vi "Main (1366x768).vi"() -> ()   [LabVIEW 2013]
uses:
  Controls/Enum - SRTRS State.ctl
  <vilib>/Utility/miscctls.llb/LVRowAndColumnTypeDef.ctl
  <vilib>/Utility/config.llb/NI_LVConfig.lvlib
  <vilib>/Utility/miscctls.llb/LVPointTypeDef.ctl
  Controls/Combo Box.ctl
  Controls/ET3500 Program Status.ctl
  <vilib>/nisyscfg/nisyscfg.lvlib
  <vilib>/Utility/miscctls.llb/LVRowAndColumnUnsignedTypeDef.ctl
  <vilib>/event_ctls.llb/eventvkey.ctl
  <vilib>/Utility/miscctls.llb/LVSelectionTypeDef.ctl
  <vilib>/nisyscfg/Close (System).vi
  <vilib>/Utility/config.llb/Write Key (String).vi
panel:
  in  "Tab Header":enum32{"Page 1"}(tab)
  in  "Close":bool
  out "Plant and Furnace Name":string="OneSubsea, Johor / BH0277."
  in  "Setup Load Debug":bool
  in  "Debug Close":bool
  in  "Tab Footer":enum32{"Page 2"}(tab)
  out "date/time string":string="Jan 25, 2014  09:14:11"
  out "File Version":string
  in  "Tab Body":T1(tab)=enum."Master Data"
  in  "User":string
  in  "Setup New":bool
  in  "Setup Edit":bool
  out "Transaction No":string caption="Transaction No."
  in  "Tab Setup":enum32{"Part Details", "Furnace Settings"}(tab)=enum."Furnace Settings" caption="Setup"
  in  "Channel Mapping":T2 caption="Channels Mapping"
  in  "Item Details":T3={"Order No."="", "Oper. No."="", "Qty."=1, "NCR No."="", "NCR Boolean"=FALSE, "Customer No."="", "Customer Name"="", "Project"="", "Sales Order"="", "Item No."="", "Material"="", "Revision"="", "Material Description"="", "Serial No."="", "Material Filename"=""} {"Qty." min=1 max=99}
  in  "Part Details Delete":bool
  in  "Part Details Add":bool
  in  "Notes":string
  in  "No.":i32=1 caption="Item Number" min=1 max=100
  out "Setup Thermocouple Location":picture caption="Thermocouples Position: Outline"
  in  "Part Details":i32(listbox)=-1
  in  "FHS Ramp Rate Units":string="°C"
  in  "cRIO Set Time":bool
  in  "Read ET3500 Program":bool
  in  "FHS Target Temp Units":string="°C"
  in  "MCListBox AWPS Remove Button":bool
  in  "MCListBox AWPS Add Button":bool
  out "CompactRIO Module Details":i32(listbox)=-1
  out "Furnace Calibration":T4={"Furnace Serial No"="100", "Last Inspection Date"="2013-12-05", "Next Inspection Due Date"="2014-12-05"} caption="Furnace Details"
  in  "Additional WPS/Ref":T6 caption="Additional WPS"
  in  "WPS Details Setup":T7={"WPS/Ref"="", "Rev"="", "Hold Temperature"="", "WPS Details Temperature Units"="°C", "Hold Time (HH:MM)"="", "Extra WPS"="", "Extra Rev"=""} caption="WPS Details"
  in  "MCListBox AWPS":i32(listbox)=-1 caption="Additional WPS/Ref MCListBox"
  out "MCListBox FHS Setup":i32(listbox)=-1 caption="Furnace Heating Sequence"
  in  "MCListBox FHS Setup Add Button":bool
  in  "MCListBox FHS Setup Remove Button":bool
  in  "Setup Save":bool
  in  "Parameter":bool
  out "ET3504 Status":string="Offline."
  out "Info.":T8={"Variant Allowed +/-"=5.0, "Hold. Time (hour:minute)"="00:00", "Hold. Temp."="0", "Info. Temperature Units"="°C", "Info. WPS/Ref."="", "Info. Temperature Units 2"="°C", "Variant Allowed"=FALSE} {"Variant Allowed +/-" format="%.1f"}
  out "Hold Time Completed":bool
  out "Process Completed":bool
  out "% Hold. Time Completed":dbl(slide) scale=0.0..100.0
  out "Transaction No 2":string caption="Transaction No."
  out "Key Values":T9={"Recording Duration"=0.0, "Remaining Hold Time"=0.0, "Current Temp"=0.0, "Key Values Temperature Units"="°C"} {"Current Temp" format="%#_4f"; "Remaining Hold Time" format="%<%H:%M>t"; "Recording Duration" format="%<%H:%M:%S>t"}
  out "No. of Items":i32
  out "Raw Data File":string
  out "Chart":dynamicdata(graph)
  in  "Recipe Start":bool
  in  "Recipe Stop":bool
  out "cRIO Status":string="Offline."
  in  "Report Open":bool caption="Report Execute Search"
  in  "Report List":i32(listbox)=-1 caption="List"
  in  "Report Generate":bool
  in  "Raw Data File":path
  in  "Report Selection":T10={"Date Start"=timestamp(0 s since 1904-01-01), "Date End"=timestamp(0 s since 1904-01-01), "Selection Transaction No"="009.*", "Selection Order No"="", "Report Execute Search "=FALSE} caption="Selection" {"Date End" format="%<%d/%m/%Y>T"; "Date Start" format="%<%d/%m/%Y>T"}
  in  "Tab Master Data":enum32{"Material", "WPS"}(tab)
  in  "Material":T11 caption="Header"
  in  "Material New":bool
  in  "Material Browse":bool
  in  "Material Delete":bool
  in  "Material Save":bool caption="Material Add"
  out "Master Data Thermocouple Location":picture caption="Thermocouples Position: Outline"
  in  "MasterData FHS Target Temp Units":string="°C"
  in  "MasterData FHS Ramp Rate Temp Units":string="°C"
  in  "WPS Details Master Data":T12={"Master Data WPS/Ref"="", "Master Data Rev"="", "Master Data Hold Temperature"="", "Master Data Temperature Units"="°C", "Master Data Hold Time (HH:MM)"=""} caption="Header"
  in  "MCListBox FHS Master Data":i32(listbox)=-1 caption="Furnance Heating Sequence"
  in  "Master Data New":bool
  in  "Master Data Save":bool
  in  "MCListBox FHS Master Data Remove Button":bool
  in  "MCListBox FHS Master Data Add Button":bool
  in  "Master Data Delete":bool
  out "Property Node Error":errorcluster
  in  "Mytab":T13(tab)
  in  "Setup":path=path "c:/temp/SRTRS4070/Setup"
  in  "MasterData\\WPS":path=path "c:/temp/SRTRS4070/MasterData/WPS" caption="Master Data WPS"
  in  "MasterData\\JPG":path=path "c:/temp/SRTRS4070/MasterData/JPG"
  in  "Data":path=path "c:/temp/SRTRS4070/Data" caption="Folder Data"
  in  "Excel":path=path "c:/temp/SRTRS4070/Excel" caption="Folder Excel"
  in  "Logs":path=path "c:/temp/SRTRS4070/Logs"
  in  "Reports":path=path "c:/temp/SRTRS4070/Reports" caption="Folder Report"
  in  "Data_Host":path=path "c:/temp/SRTRS4070_Host/Data_Host" caption="Folder Data"
  in  "Logs_Host":path=path "c:/temp/SRTRS4070_Host/Logs_Host"
  out "Lite Version":bool=TRUE
  out "stp file Error Out":errorcluster
  out "Temperature Units (ini)":string="°C"
  out "Furnace Number":string="03"
  out "Running Number":i32=515
  out "Show Debug Tab":bool=TRUE
  out "Show LabVIEW Error":bool
  out "Application:Name":string="LabVIEW.exe"
  out "Metrics:Code Size":u32=647236 format="%#.3p"
  out "MCListBox Ref":refnum<vi>[](array[refnum])
  in  "CellBG ColHdrs":u32(colorbox)=11776947
  in  "CellBG Unused Cells":u32(colorbox)=16777238
  in  "CellBG New Cells":u32(colorbox)=16777225
  out "Latest stp file":path
  out "Channel to Probe Mapping":cluster{"Channel to Probe Mapping":string}={"Channel to Probe Mapping"="1,2,3,0,0,0,0,4,0,0,0,0,0,0,0,0"}
  out "Probe List":i32[](array[numeric])
  out "Probe List Valid":bool
  out "cRIO Channel List":i32[](array[numeric])
  out "Empty String in Mandatory Field":bool
  out "All Cells Filled":bool
  out "FHS Last Row":i32
  out "Final Target Temperature":cluster{"Final Target Temperature":string}
  in  "Parameter Buffer":T14
  out "Parameter (End Dwell Time)":timestamp
  out "Parameter (Start Dwell Time)":timestamp
  out "ET3500 Error":errorcluster
  in  "Simulate ET3500":bool=TRUE
  out "Parameter Cluster (Scaled)":T15={"ProgramNumber"=1, "CurProg"=33, "CurSeg"=1, "ProgStatus"=1, "ProgTimeLeft (min)"=0.0, "PVIn (DegC)"=12000.0, "SPIn (s)"=0.0, "SegTimeLeft (min)"=0.0}
  in  "Simulate ET3500 Error":bool
  in  "Final Target Temp Offset":i32
  in  "Stop On Final Target Temperature":bool
  out "Final Target + Offset\n(Updated Only when active)":i32
  in  "Simulate cRIO No Data":bool
  out "cRIO DAQ Start":bool
  out "cRIO Error":errorcluster
  out "cRIO Cycle Count":i32
  out "cRIO shared variable RT Library":string="ni.var.psp://192.168.1.50/RT Library"
  out "VISA resource name RS232":string="visa://192.168.1.50/ASRL1::INSTR"
  out "Samples/ch Count":i32
  out "Start Cycle":u32
  out "cRIO COM Port":string="visa://192.168.1.50/ASRL1::INSTR"
  out "Host COM Port":string="COM3"
  out "cRIO IP":string="192.168.1.50"
  out "cRIO Folder":string="/c/ni-rt/LabVIEW Data/SRTRS4070"
  in  "Simulate cRIO":bool=TRUE caption="Simulate cRIO Data"
  in  "Use Local COM Port":bool caption="Use Host COM Port"
  out "cRIO Data Retention":i32=3
  out "cRIO Timestamp (only updated when a Shared Variable is Read)":timestamp
  in  "Simulate cRIO Comm Error":bool
  out "Data Path Name":string
  in  "Simulate cRIO Started":bool
  out "Data File Error":errorcluster
  out "Logged File Ref":refnum<file>
  out "Time to next sample (s)":dbl
  out "Host Sampling Interval (s)":dbl=0.1
  in  "Time Target (s)":dbl format="%#_13g"
  out "Data File":path
  out "List Of Files From Selected Reports":string[](array[string])
  out "YYYYmm":string
  out "Details From .stp and Parameters":string[](array[string])
  out "Order No":string[](array[string])
  in  "Report.Create.PDF":bool=TRUE caption="Create PDF file at end of Recipe"
  in  "Report.Create.Excel":bool=TRUE caption="Create EXCEL file at end of Recipe"
  in  "---------------------------------       Master Data (Material)      -----------------------------":string
  out "Temp Array":string[](array[string])
  out "Time has Elapsed":bool
  out "Quit Flag":bool
  out "Recipe Start Flag":bool
  out "Recipe Stop Flag":bool
  out "Time":u32
  out "Process 2 t0":u32=72507500
  out "Process 1 t0":u32=72487300
  out "Image File Path":path
  in  "------------------------------------        Master Data       -----------------------------------":string
  in  "------------------------------------        MCListBox       ------------------------------------":string
  in  "------------------------------------             Report          ------------------------------------":string
  in  "------------------------------------        Part Details       ------------------------------------":string
  out "Enum":T16=enum."QUIT"
  out "Show Scrollbars":bool=TRUE
  out "State":string="QUIT"
  in  "WPS Details Buffer":T7={"WPS/Ref"="", "Rev"="", "Hold Temperature"="", "WPS Details Temperature Units"="°C", "Hold Time (HH:MM)"="", "Extra WPS"="", "Extra Rev"=""}
  out "MessageQ":string="000003\t20140125_091408\t[QUIT] Clicked By User.\n000002\t20140125_091406\t\"c:\\temp\\SRTRS4070_Host\\Logs_Host\\2014\\01\\20140125_091406.log\" Event File Created.\n000001\t20140125_091406\tReady to Start.\n000000\t20140125_091406\t\"C:\\Users\\CK\\workspace\\LabVIEW\\Stress Relief Temperature Recording\\MyEXE.ini\" is Loaded. 27 out of 27 Keys are FOUND.  Code Size = 647236.\n\n\n\n\n\n\n\n\n\n\n\n\n\n\n\n\r\n"
  out "State Machine Error Out":errorcluster
  out "Event File Error":errorcluster
  out "MessageQ Error":errorcluster
  # "Stress Relief Temperature Recording System"
  # "Thermocouple"
  # "Probe No."
  # "EA"
  # "(     )"
  # "(     / Hour )"
  # "System Status"
  # "(hh:mm:ss)"
  # "(hh:mm)"
  # "Probe Number"
  # "Create Report"
  # "Display Report"
  # "to"
  # "Date"
  # "OR"
  # "Material Details"
  # "WPS Details"
  # "(      / Hour )"
  # "(      )"
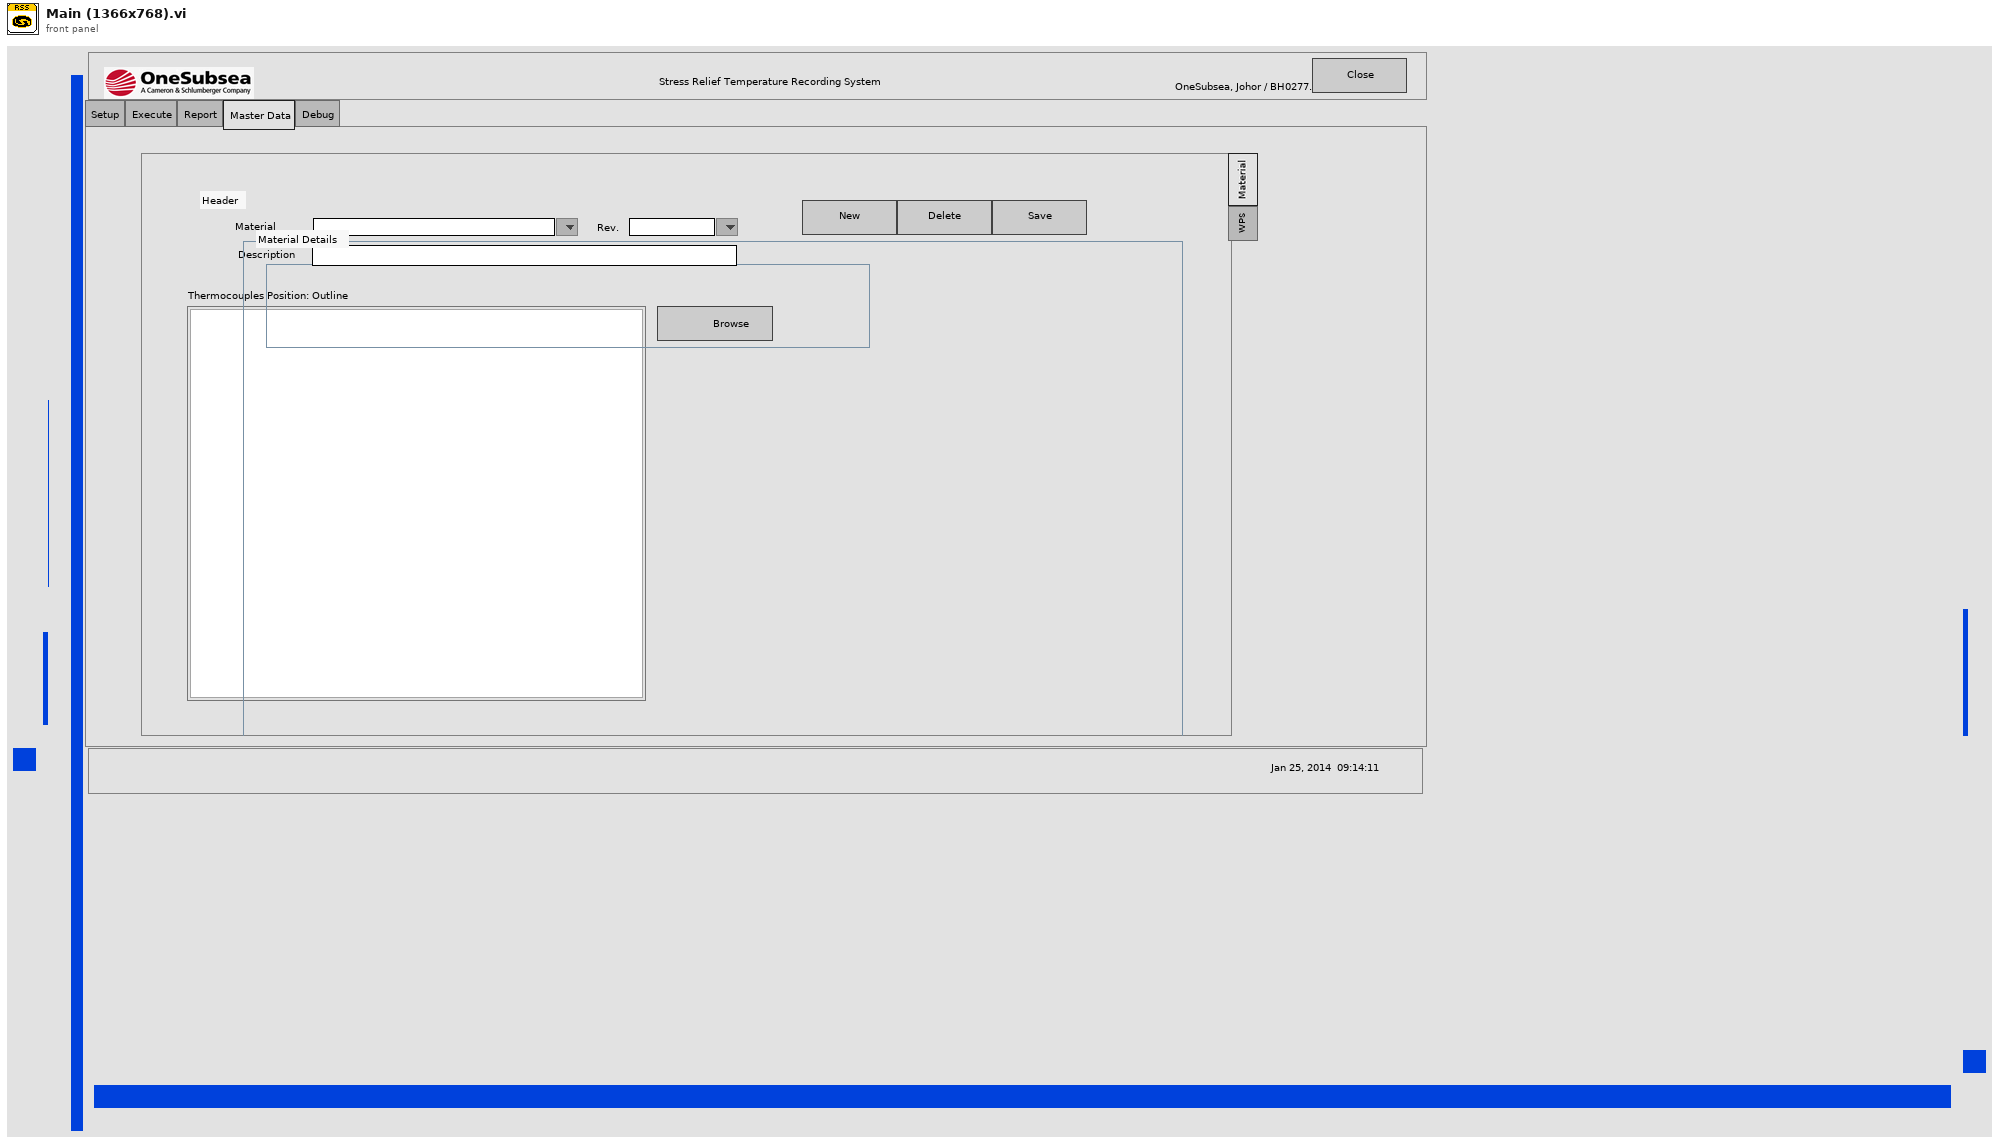
[diagram p1: front panel]
types:
  T1 = enum32{"Setup", "Execute", "Report", "Master Data", "Debug"}
  T2 = cluster{"TC1":string, "TC2":string, "TC3":string, "TC4":string, "TC5":string, "TC6":string}
  T3 = cluster{"Order No.":string, "Oper. No.":string, "Qty.":i32, "NCR No.":string, "NCR Boolean":bool, "Customer No.":string, "Customer Name":string, "Project":string, "Sales Order":string, "Item No.":string, "Material":string, "Revision":string, "Material Description":string, "Serial No.":string, "Material Filename":string}
  T4 = cluster{"Furnace Serial No":string, "Last Inspection Date":string, "Next Inspection Due Date":string}
  T5 = typedef "Combo Box.ctl" = string
  T6 = cluster{"Additional WPS/Ref":T5, "Additional Rev":T5}
  T7 = cluster{"WPS/Ref":T5, "Rev":T5, "Hold Temperature":string, "WPS Details Temperature Units":string, "Hold Time (HH:MM)":string, "Extra WPS":string, "Extra Rev":string}
  T8 = cluster{"Variant Allowed +/-":dbl, "Hold. Time (hour:minute)":string, "Hold. Temp.":string, "Info. Temperature Units":string, "Info. WPS/Ref.":string, "Info. Temperature Units 2":string, "Variant Allowed":bool}
  T9 = cluster{"Recording Duration":dbl, "Remaining Hold Time":dbl, "Current Temp":dbl, "Key Values Temperature Units":string}
  T10 = cluster{"Date Start":timestamp, "Date End":timestamp, "Selection Transaction No":string, "Selection Order No":string, "Report Execute Search ":bool}
  T11 = cluster{"Master Data Material":string, "Master Data Rev":string, "Master Data Material Description":string}
  T12 = cluster{"Master Data WPS/Ref":T5, "Master Data Rev":T5, "Master Data Hold Temperature":string, "Master Data Temperature Units":string, "Master Data Hold Time (HH:MM)":string}
  T13 = enum32{"Paths", "Host Paths", "Settings", "Part Details Add/Edit", "ET3500", "cRIO", "Data File", "Report", "Others", "Recovery"}
  T14 = cluster{"Start Holding Time and Date":string, "End Holding Time and Date":string, "Start Holding Temperature":string, "End Holding Temperature":string}
  T15 = cluster{"ProgramNumber":i16, "CurProg":i16, "CurSeg":i16, "ProgStatus":i16, "ProgTimeLeft (min)":dbl, "PVIn (DegC)":dbl, "SPIn (s)":dbl, "SegTimeLeft (min)":dbl}
  T16 = typedef "Enum - SRTRS State.ctl" = enum16{"READY TO START", "START Recipe", "START Recovery", "BEGIN Process", "RUNNING Process", "END Process", "Spare Enum", "END Recipe", "ERROR Handling", "QUIT"}
  T17 = typedef "ET3500 Program Status.ctl" = enum16{"Wait For RUN", "Running", "Stopped"}
  T18 = enum16{"Always On", "Always Off", "Off While Running"}
  T19 = cluster{"Variant Allowed +/-":dbl, "Hold Time (HH:MM)":string, "Hold Temp.":string, "Info. Temperature Units":string, "Info. WPS/Ref.":string, "Info. Temperature Units 2":string, "Variant Allowed":bool}
  T20 = typedef "LVPointTypeDef.ctl" = cluster{"Horizontal":i16, "Vertical":i16}
  T21 = typedef "LVRowAndColumnTypeDef.ctl" = cluster{"Row":i32, "Column":i32}
  T22 = typedef "LVRowAndColumnUnsignedTypeDef.ctl" = cluster{"Row":u32, "Column":u32}
  T23 = enum32{"Page Enabled", "Page Disabled", "Page Disabled & Grayed"}[]
  T24 = cluster{"SRTRS4070 Folder":string, "cRIO Folder":string, "cRIO IP":string, "Temperature Units":string, "Furnace Number":string, "Plant and Furnace Name":string, "LogoFile":string, "Software Solution Name":string, "Channel to Probe Mapping":string, "Running Number":string, "Permitted Temperature Difference":string, "Permitted Time Difference":string, "Host COM Port":string, "Host Sampling Interval":string, "cRIO Data Retention":string, "cRIO Time Sync Schedule":string, "cRIO Time Sync Tolerance":string, "Date Format":string, "SRTRS4070 Host Folder":string, "Latest stp File":string, "Log Off Timer":string, "Raw Data File":string, "Layout Details":string}
  T25 = cluster{"Furnace Serial No":string, "Last Calibration Date":string, "Next Calibration Due Date":string}
  T26 = typedef "Connection Information Cluster.ctl" = cluster{"Connection ":string, "Username":string, "Password":string}
  T27 = enum8{"Enabled", "Disabled", "Disabled and Grayed Out"}
  T28 = enum16{"open", "replace", "create", "open or create", "replace or create", "replace or create with confirmation"}
  T29 = enum16{"Blank Cells Only", "Exisiting and Blank Cells"}
  T30 = cluster{"Show":bool, "Priority":i32, "Message":string}
  T31 = typedef "eventvkey.ctl" = enum16{"ASCII", "Enter", "Return", "Shift", "Ctrl", "Alt", "Cmd", "Opt", "Caps", "NumLock", "Clear", "Break", "Up", "Down", "Left", "Right", "Insert", "Delete", "Home", "End", "PageUp", "PageDown", "Escape", "Help", "Pause", "ScrollLock", "F1", "F2", "F3", "F4", "F5", "F6", "F7", "F8", "F9", "F10", "F11", "F12", "F13", "F14", "F15", "F16", "F17", "F18", "F19", "F20", "F21", "F22", "F23", "F24", "Play", "VolumeUp", "VolumeDown", "Mute", "Two Byte Char"}
  T32 = typedef "LVSelectionTypeDef.ctl" = cluster{"Selection Start":u32, "Selection End":u32}
  T33 = typedef "NI_LVConfig.lvlib/Config Data RefNum.ctl" = refnum<k1>
  T34 = typedef "imagedata.ctl" = cluster{"image type":i32, "image depth":i32, "image":u8[], "mask":u8[], "colors":u32[], "Rectangle":cluster{"left":i16, "top":i16, "right":i16, "bottom":i16}}
  T35 = cluster{"Numeric Control":i32, "Numeric Control":i32}
  T36 = cluster{"ProgramNumber":i16, "CurProg":i16, "CurSeg":i16, "ProgStatus":i16, "ProgTimeLeft (min)":dbl, "PVIn (degC)":dbl, "SPIn (NA)":dbl, "SegTimeLeft (min)":dbl}
  T37 = cluster{"Start Holding Time & Date":string, "End Holding Time & Date":string, "Start Holding Temperature":string, "End Holding Temperature":string}
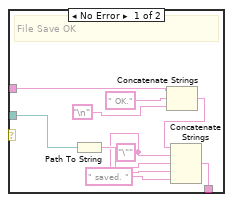
[diagram p2: hidden frame]
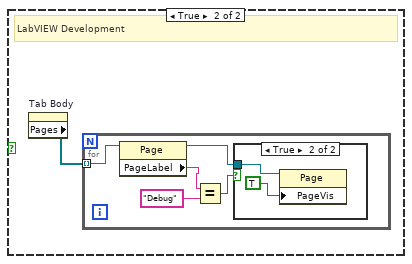
[diagram p4: hidden frame]
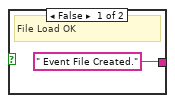
[diagram p6: hidden frame]
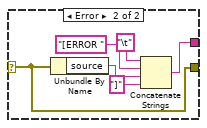
[diagram p9: hidden frame]
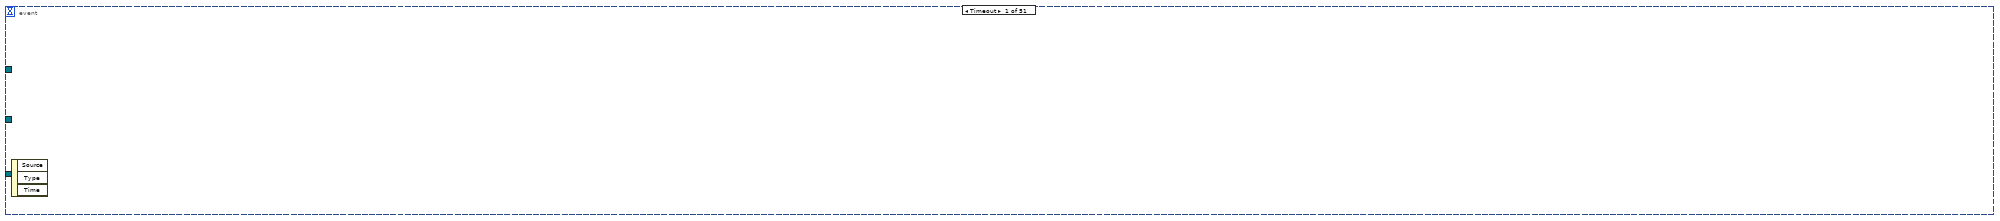
[diagram p10: hidden frame]
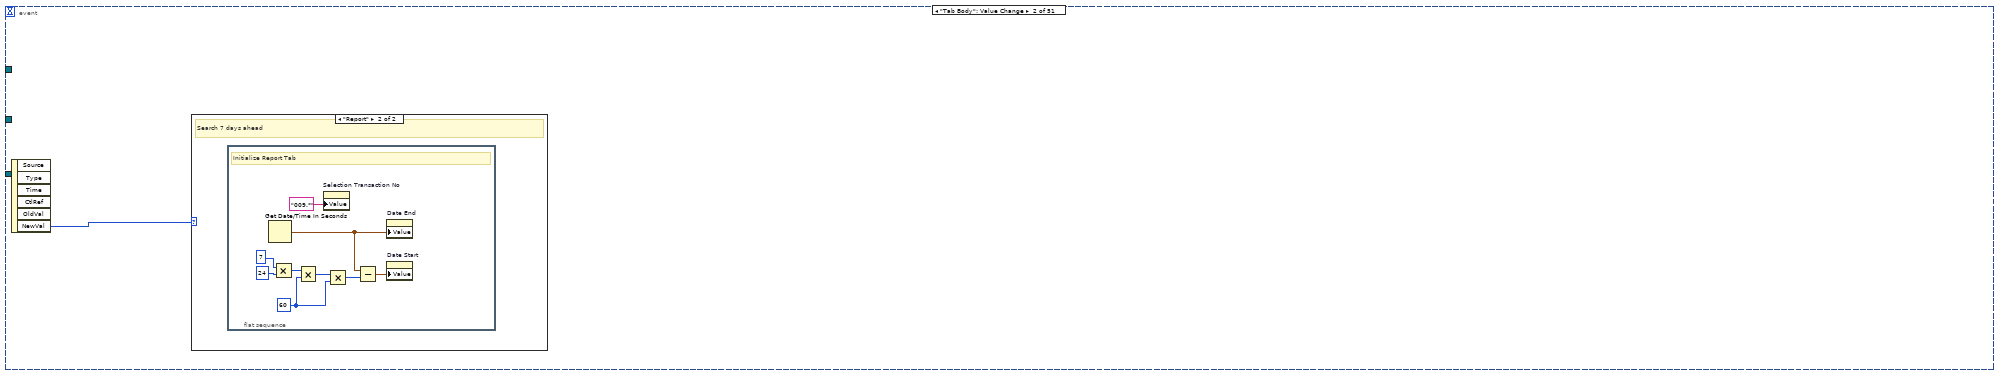
[diagram p11: hidden frame]
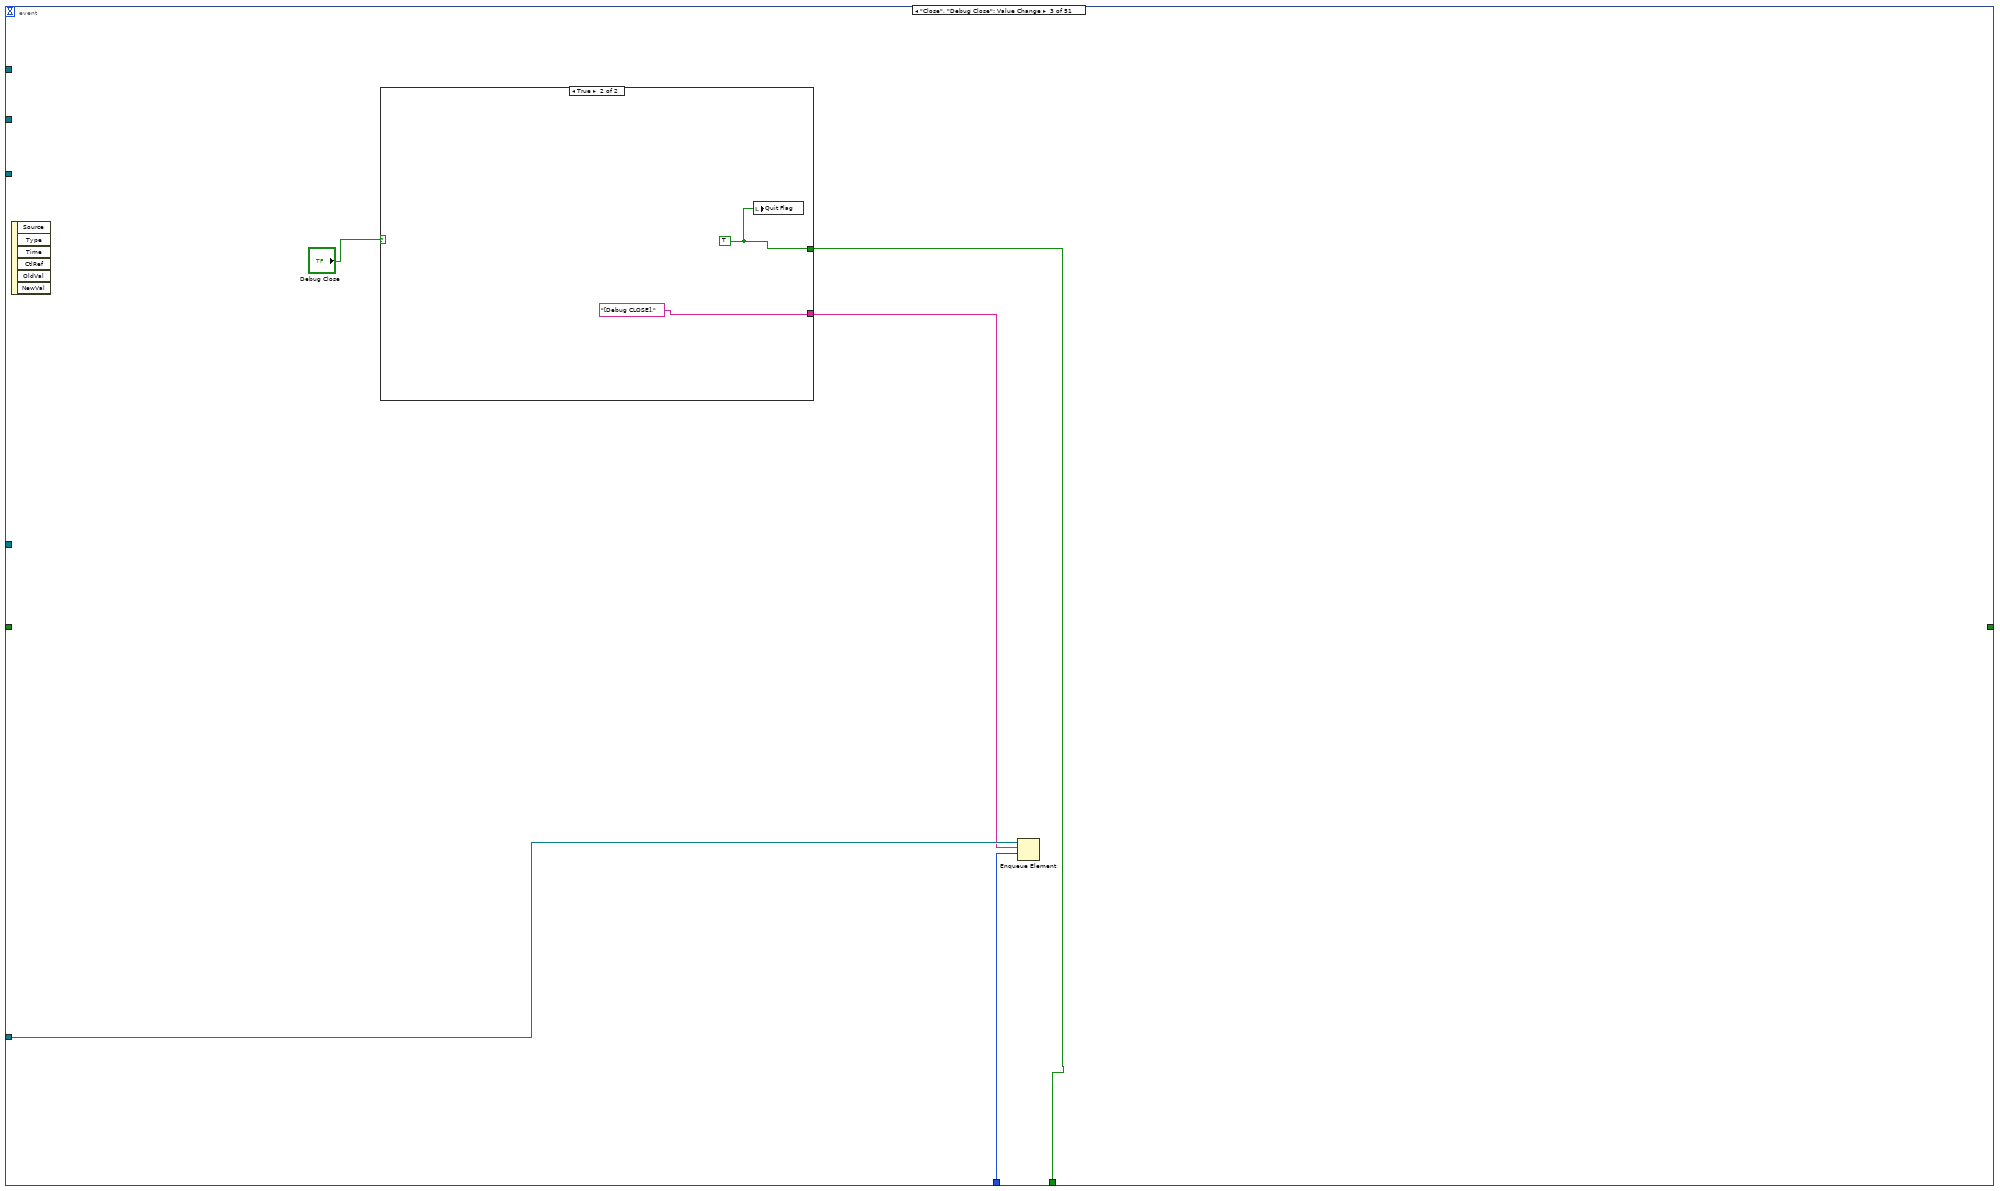
[diagram p13: hidden frame]
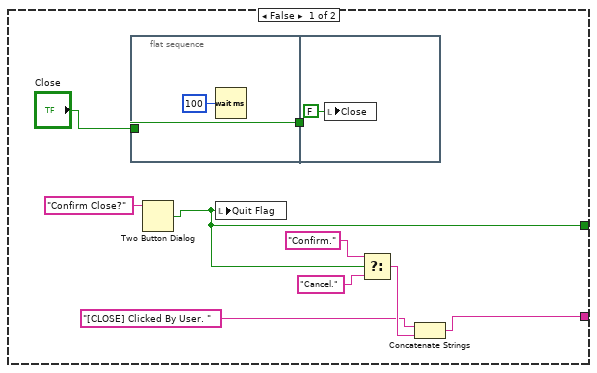
[diagram p14: hidden frame]
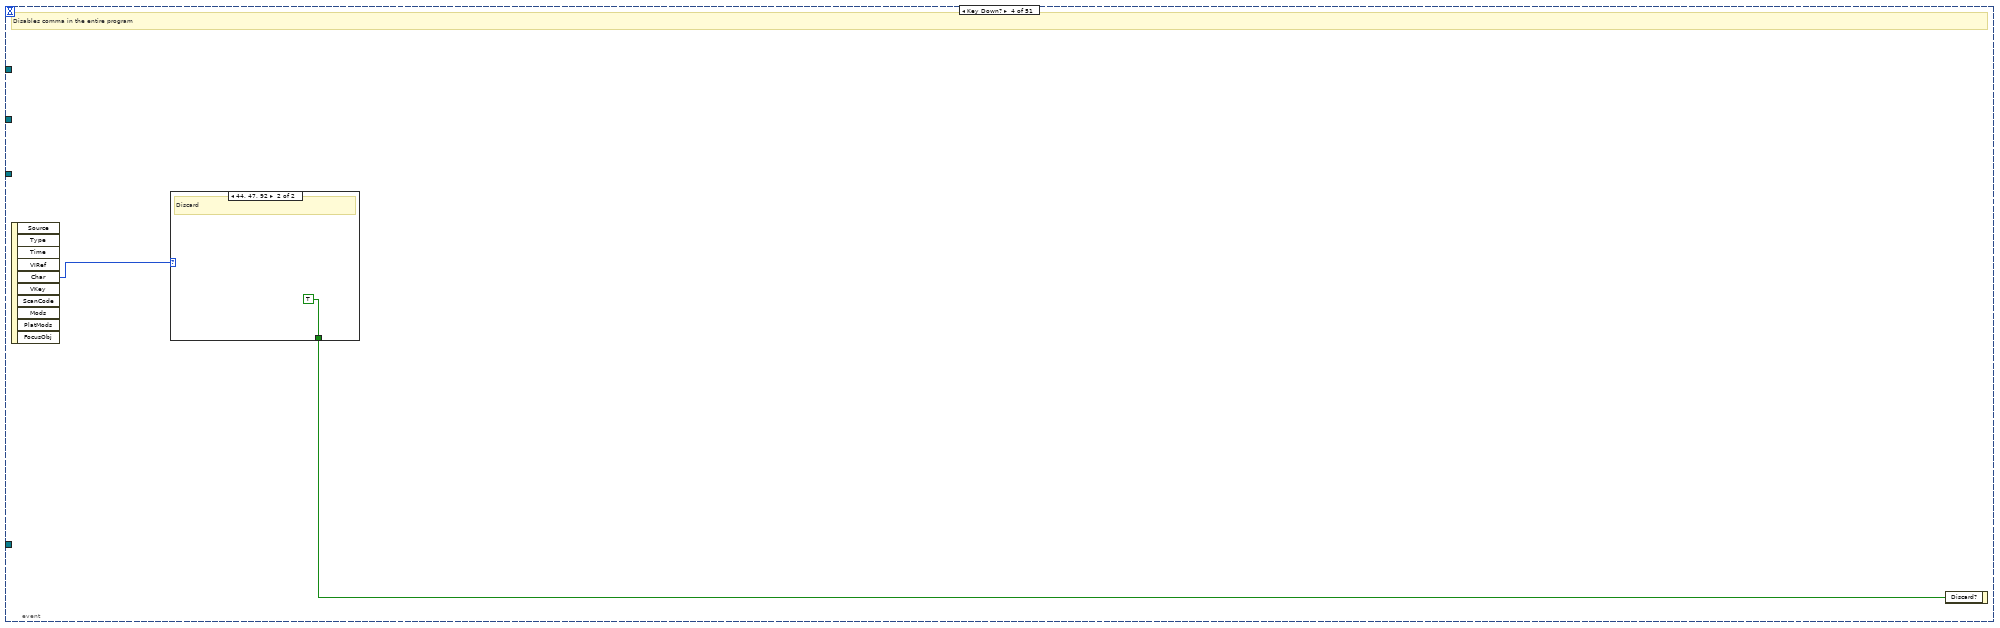
[diagram p15: hidden frame]
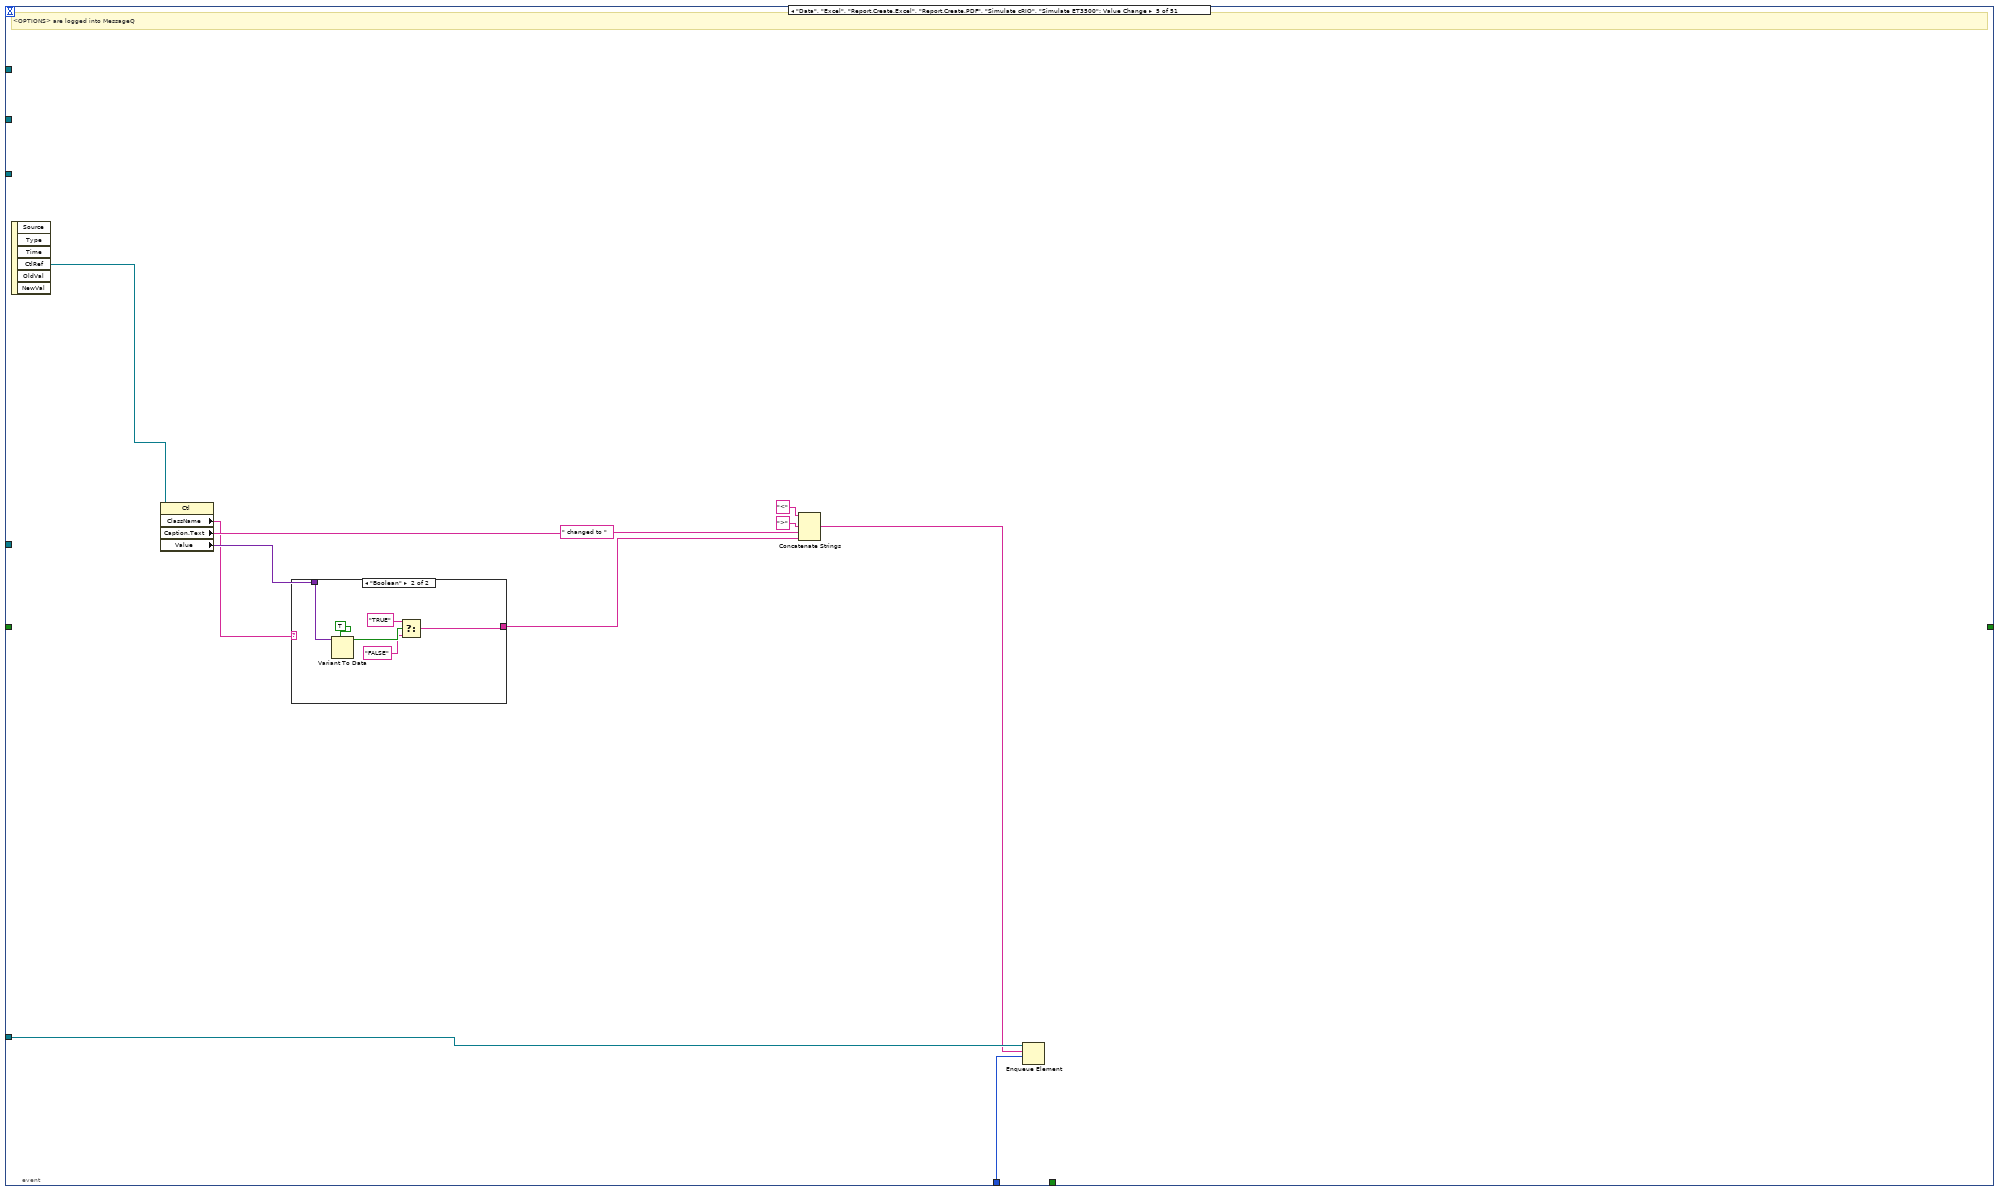
[diagram p17: hidden frame]
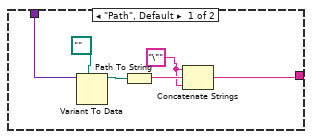
[diagram p18: hidden frame]
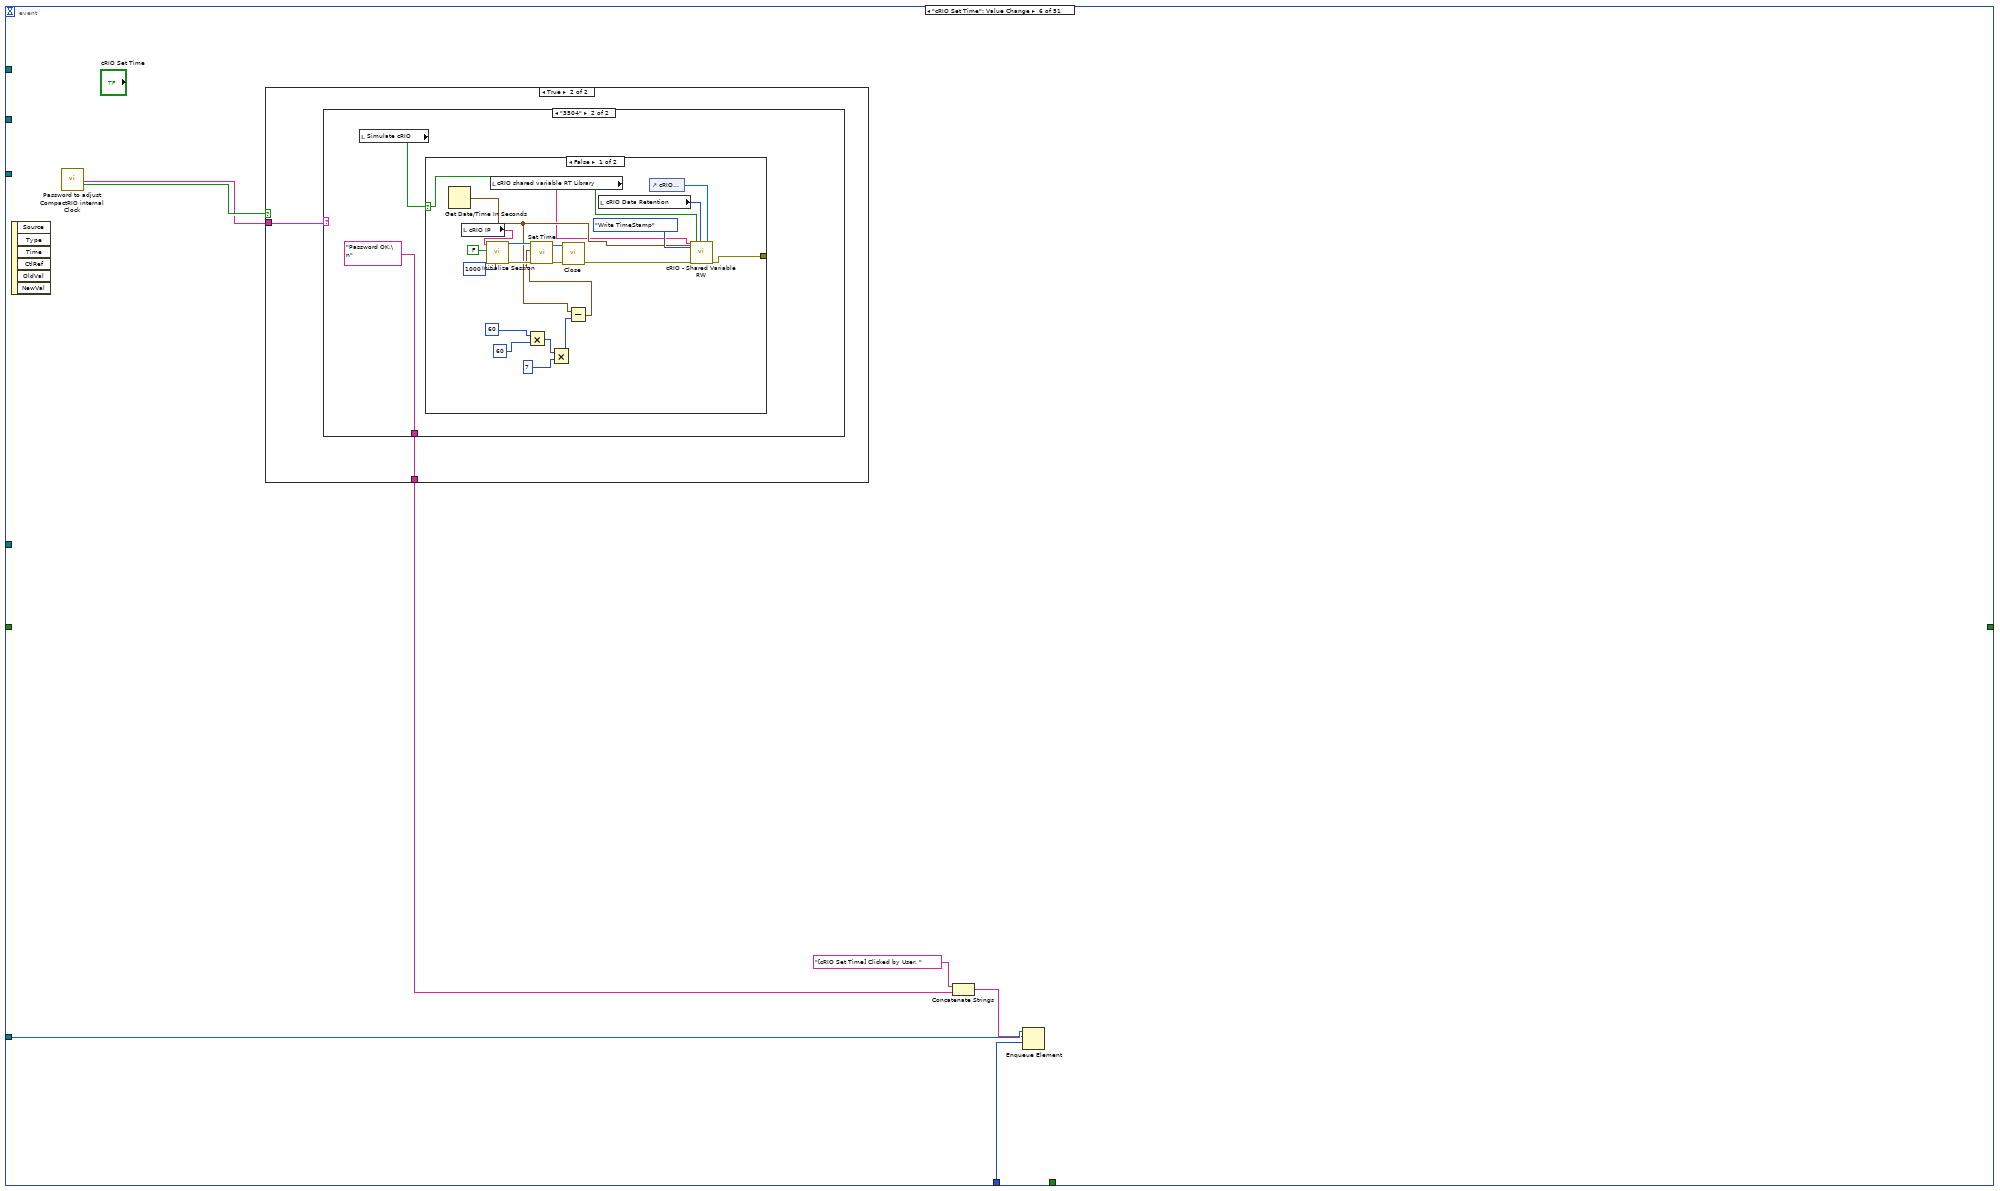
[diagram p19: hidden frame]
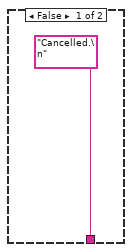
[diagram p20: hidden frame]
diagram:
  w5 = i16 -1  # Segment.Type (unknown)
  w8 = 0  # Sample/ch Count
  w9 = 0  # Cycle Count
  w19 = 20  # Shows Last 20 Events
  n1 = flat-sequence {
    frame #0 {
      # "References [<Functional Specification version>][<Section>]"
    }
  }
  n2 = control-ref of="This VI"() -> (w3:refnum<vi>)
  n3 = invoke class="VI" method="Default Vals.Reinit All"(reference=w3) -> (reference out=w1:refnum<vi>, error out=w7:errorcluster)  [unwired: 2 in, 1 out]
  n4 = flat-sequence {
    tunnel: [errorcluster {"status"=FALSE, "code"=0, "source"=""} ("error out")] -> w24
    tunnel: [w181] -> w17
    tunnel: [w178] -> w13
    tunnel: w7 -> [_]
    tunnel: w1 -> [w78]
    frame #0 {
      w27 = FALSE ("Show Scrollbars")
      w79 = FALSE ("Visible")
      w43 = u32 3 ("Number of Rows")
      w91 = T22 {"Row"=0, "Column"=0} ("Top Left Visible Cell")
      w88 = refnum<vi>[] [] ("ControlsOnPage")
      w123 = string[] ["Sequence Number", "Ramp Rate", "Target Temperature"] ("Column Header Strings[]")
      w126 = T23 [enum."Page Enabled", enum."Page Enabled", enum."Page Enabled", enum."Page Enabled", enum."Page Enabled"] items=["Page Enabled", "Page Disabled", "Page Disabled & Grayed"]
      w160 = 3 ("dimension size")
      w42 = 2 ("dimension size")
      # "Initialization"
      n5 = property class="VI"(reference=w78) -> (reference out=w76:refnum<vi>, "Panel"=w77:refnum<vi>)  [unwired: 1 in, 1 out]
      n6 = control-ref of="MCListBox FHS Setup Remove Button"() -> (w81:refnum<vi>)
      n7 = control-ref of="MCListBox FHS Setup Add Button"() -> (w80:refnum<vi>)
      n8 = property class="Pnl"(reference=w77) -> ("Panes[]"=w75:refnum<vi>[])  [unwired: 1 in, 2 out]
      n9 = Select(t=T18."Always On" ("Vertical Scrollbar Visibility"), s=w27, f=T18."Off While Running" ("Vertical Scrollbar Visibility")) -> (s? t:f=w71:T18)
      n10 = Index Array(array=w75) -> (element=w74:refnum<vi>)  [unwired: 1 in]
      n11 = property class="Bool"(reference=w81, "Visible"=w79) -> ()  [unwired: 1 in, 2 out]
      n12 = property class="Bool"(reference=w80, "Visible"=w79) -> ()  [unwired: 1 in, 2 out]
      n13 = property class="VI"(reference=w76) -> ("Metric.CodeSize"=w104:u32)  [unwired: 1 in, 2 out]
      "Metrics:Code Size" <- w104
      n14 = property class="Pane"(reference=w74, "HorizScrollbarVisibility"=w71, "VertScrollbarVisibility"=w71) -> ()  [unwired: 1 in, 2 out]
      n15 = case shown="\"Debug\"" enum16{"Header", "Body", "Debug"}."Header" {
        tunnel: [T20 {"Horizontal"=0, "Vertical"=0} ("Origin") T20 {"Horizontal"=0, "Vertical"=75} ("Origin") T20 {"Horizontal"=0, "Vertical"=200} ("Origin")] -> w169
        frame "Header", Default {
        }
        frame "Body" {
        }
        frame "Debug" {
        }
      }
      n16 = local write "CompactRIO Module Details"(-1 ("Temperature Module Calibration")) -> ()
      n17 = property on="Tab Body" class="TabCtl (strict)"() -> ("Pages"=w127:refnum<vi>[])  [unwired: 2 in, 2 out]
      n18 = local write "Report Generate"(FALSE ("Report Generate")) -> ()
      n19 = local write "Close"(FALSE ("Quit")) -> ()
      n20 = property on="Pane" class="Pane"("Origin"=w169) -> ()  [unwired: 2 in, 2 out]
      n21 = control-ref of="This Application"() -> (w108:refnum<vi>)
      n22 = for {
        tunnel: w127 -> [w281] mode=indexing
        tunnel: w126 -> [w280] mode=indexing
        n23 = property class="Page"(reference=w281, "PageEnb"=w280) -> ()  [unwired: 1 in, 2 out]
      }
      n24 = Format Into String(format string="%d.", initial string="Code Size = ", w104) -> (resulting string=w101:string)  [unwired: 1 in, 1 out]
      n25 = disable-structure shown="Disabled" {
        frame Disabled {
          n26 = property on="Tab Setup" class="TabCtl (strict)"() -> ("Pages"=w247:refnum<vi>[])  [unwired: 2 in, 2 out]
          n27 = property on="Tab Master Data" class="TabCtl (strict)"() -> ("Pages"=w246:refnum<vi>[])  [unwired: 2 in, 2 out]
          n28 = Build Array (concatenate)(w247, w246) -> (w245:refnum<vi>[])
          n29 = for {
            tunnel: w245 -> [w249] mode=indexing
            tunnel: [w248] -> w244 mode=concatenating
            n30 = property class="Page"(reference=w249) -> ("ControlsOnPage"=w248:refnum<vi>[])  [unwired: 1 in, 2 out]
          }
          n31 = for {
            tunnel: w244 -> [w251] mode=indexing
            # "Show/Hide All Labels"
            n32 = property class="Ctl"(reference=w251, "Label.Visible"=FALSE) -> ()  [unwired: 1 in, 2 out]
          }
        }
        frame Enabled {
        }
      }
      n33 = Initialize Array("", 3 ("dimension size")) -> (w175:string[])
      n34 = Initialize Array("", w160) -> (w163:string[])
      n35 = property class="App"(reference=w108) -> (error out=w51:errorcluster, "App.Dir"=w58:path, "App.Name"=w57:string)  [unwired: 1 in, 1 out]
      "Application:Name" <- w57
      n36 = Initialize Array("", w42) -> (w173:string[])
      n37 = property on="Tab Body" class="TabCtl (strict)" props=["Pages"]() -> ()  [unwired: 2 in, 3 out]
      n38 = property on="Tab Setup" class="TabCtl (strict)" props=["Pages"]() -> ()  [unwired: 2 in, 3 out]
      n39 = property on="Tab Master Data" class="TabCtl (strict)" props=["Pages"]() -> ()  [unwired: 2 in, 3 out]
      n40 = Build Array(w175) -> (w176:string[][])
      n41 = Build Array(w163) -> (w162:string[][])
      n42 = Build Array(w173) -> (w41:string[][])
      n43 = control-ref of="CompactRIO Module Details"() -> (w66:refnum<vi>)
      n44 = control-ref of="Report List"() -> (w62:refnum<vi>)
      n45 = control-ref of="Part Details"() -> (w165:refnum<vi>)
      n46 = property on="MCListBox FHS Setup" class="MCListbox (strict)"("ItemNames"=w162, "NumCols"=w160, "ColHdrString"=w123) -> ()  [unwired: 2 in, 2 out]
      n47 = property on="MCListBox FHS Master Data" class="MCListbox (strict)"("ItemNames"=w176, "NumCols"=3 ("dimension size"), "ColHdrString"=w123) -> ()  [unwired: 2 in, 2 out]
      n48 = property on="MCListBox AWPS" class="MCListbox (strict)"("ItemNames"=w41, "NumCols"=w42) -> ()  [unwired: 2 in, 2 out]
      n49 = Build Path(base path=w58, name or relative path=w57) -> (appended path=w56:path)
      n50 = Path To String(path=w56) -> (string=w55:string)
      n51 = control-ref of="MCListBox FHS Setup"() -> (w90:refnum<vi>)
      n52 = control-ref of="MCListBox FHS Master Data"() -> (w39:refnum<vi>)
      n53 = control-ref of="MCListBox AWPS"() -> (w98:refnum<vi>)
      n54 = invoke class="FileVersionInfo" method="GetVersionInfo"(error in=w51, "fileName"=w55) -> (reference out=w52:refnum<k24>, error out=w50:errorcluster, "GetVersionInfo"=w54:refnum<k24>)  [unwired: 2 in, 1 out]
      n55 = property class="MCListbox (strict)"(reference=w165, "ColHdrString"=string[] ["No.", "Order No.", "Oper. No.", "Qty.", "NCR No.", "Customer Name", "Project", "Sales Order", "Item No.", "Material", "Material Description", "Revision", "Serial No.", "TC1", "TC2", "TC3", "TC4", "TC5", "TC6", "Notes", "User", "Customer No.", "NCR Boolean"] ("Column Header Strings[]"), "NumRows"=w43) -> (reference out=w44:refnum<vi>)  [unwired: 1 in, 1 out]
      n56 = for {
        N: w43 -> [_]
        tunnel: w44 -> [w211]
        i -> [w210]
        n57 = for {
          N: 6 -> [_]
          tunnel: w211 -> [w218]
          tunnel: w210 -> [w215]
          tunnel: 13 -> [w214]
          i -> [w213]
          n58 = Add(x=w214, y=w213) -> (x+y=w212:i32)
          n59 = Bundle(w215, w212) -> (w216:cluster{i32, i32})  [unwired: 1 in]
          n60 = property class="MCListbox (strict)"(reference=w218, "ActiveCell"=w216, "Justify"=enum16{"Left", "Center", "Right"}."Center" ("Active Cell:Cell Justification")) -> ()  [unwired: 1 in, 2 out]
        }
      }
      n61 = property class="MCListbox (strict)"(reference=w62, "ColHdrString"=string[] ["Date and Time", "Transaction No.", "Order No."] ("Column Header Strings[]"), "NumRows"=u32 5 ("Number of Rows")) -> (reference out=w61:refnum<vi>)  [unwired: 1 in, 1 out]
      n62 = property class="MCListbox (strict)"(reference=w66, "ColHdrString"=string[] ["Module Serial No.", "Last Calibration Date", "Next Calibration Due Date"] ("Column Header Strings[]"), "NumRows"=u32 4 ("Number of Rows")) -> (reference out=w65:refnum<vi>)  [unwired: 1 in, 1 out]
      n63 = property on="Part Details Add" class="Bool (strict)"("BoolText.Text"="Add" ("Boolean Text.Text")) -> ()  [unwired: 2 in, 2 out]
      n64 = property on="Property Node" class="MCListbox (strict)"(reference=w39, "NumRows"=6 ("Multicolumn Listbox"), "TopLeft"=w91) -> ()  [unwired: 1 in, 2 out]
      n65 = property on="Property Node" class="MCListbox (strict)"(reference=w90, "NumRows"=6 ("Multicolumn Listbox"), "TopLeft"=w91) -> ()  [unwired: 1 in, 2 out]
      n66 = Build Array(w90, w39, w98) -> (w113:refnum<vi>[])
      "MCListBox Ref" <- w113
      n67 = property class="FileVersionInfo"(reference=w54, error in=w50) -> (reference out=w53:refnum<k24>, error out=w49:errorcluster, "FileVersion"=w46:string)
      n68 = property on="Mytab" class="TabCtl (strict)"() -> ("Pages"=w144:refnum<vi>[])  [unwired: 2 in, 2 out]
      n69 = Concatenate Strings("ver. ", w46) -> (→"File Version":string)
      n70 = for {
        tunnel: w144 -> [w288] mode=indexing
        shift-right: [w282] -> w97
        shift-left: w88 -> [w285]
        shift-right: [w284] -> w86
        shift-left: w88 -> [w283]
        # "Get all Paths's Ref"
        n71 = property class="Page"(reference=w288) -> ("ControlsOnPage"=w286:refnum<vi>[], "PageLabel"=w287:string)  [unwired: 1 in, 2 out]
        n72 = case shown="\"Paths\"" w287 {
          tunnel: w286 -> [_ w292 w294]
          tunnel: w285 -> [w289 _ w293]
          tunnel: [w290 w291 w294] -> w284
          tunnel: w283 -> [w290 w291 _]
          tunnel: [w289 w292 w293] -> w282
          frame "False", Default {
          }
          frame "Paths" {
          }
          frame "Host Paths" {
          }
        }
      }
      n73 = for {
        tunnel: w113 -> [w302] mode=indexing
        tunnel: "CellBG Unused Cells" -> [w305]
        tunnel: "CellBG ColHdrs" -> [w304]
        tunnel: "CellBG New Cells" -> [_]
        n74 = property on="Property Node" class="MCListbox (strict)"(reference=w302, "RowHdrs[]"=string[] ["-1,-1", "", "0,0", "-1,-1", "7"]) -> (reference out=w301:refnum<vi>)  [unwired: 1 in, 1 out]
        n75 = property on="Property Node" class="MCListbox (strict)"(reference=w301, "ActiveCell"=T21 {"Row"=-2, "Column"=-2}, "CellBG"=w305, "ActiveCell"=T21 {"Row"=-1, "Column"=-2}, "CellBG"=w304, "Value"=-1 ("Multicolumn Listbox")) -> ()  [unwired: 1 in, 2 out]
      }
      n76 = local read "CellBG Unused Cells"() -> (w166:u32)
      n77 = Close Reference(reference=w53, error in (no error)=w49) -> (error out=w48:errorcluster)
      n78 = Close Reference(reference=w52, error in (no error)=w48) -> ()  [unwired: 1 out]
      n79 = call "Get INFO from ini FILE - SRTRS.vi"("ini Name"="MyEXE.ini") -> ("Settings"=w141:T24, "Equipment Details (MCListBox)"=w139:string[][], "Furnace Details"=→"Furnace Calibration":T25, "AMS Connection Information"=w128:T26, "MessageQ"=w105:string, "Error Out"=w179:errorcluster)  [unwired: 5 in, 4 out]
      n80 = Unbundle By Name(w141) -> ("cRIO IP"=w120:string, "Host COM Port"=w118:string, "Temperature Units"=w68:string, "cRIO Folder"=→"cRIO Folder":string, "cRIO Data Retention"=w95:string, "Furnace Number"=→"Furnace Number":string, "Plant and Furnace Name"=→"Plant and Furnace Name":string, "Channel to Probe Mapping"=w136:string, "Running Number"=w138:string, "Permitted Temperature Difference"=w125:string, "Host Sampling Interval"=w111:string, "SRTRS4070 Host Folder"=w87:string, "SRTRS4070 Folder"=w89:string, "Latest stp File"=w36:string)
      "cRIO IP" <- w120
      "Temperature Units (ini)" <- w68
      "Host COM Port" <- w118
      n81 = Build Array(w44, w65, w61) -> (w177:refnum<vi>[])
      n82 = Concatenate Strings(w105, " " ("string"), w101) -> (w100:string)
      n83 = Unbundle By Name(w128) -> ("Create EXCEL"=w130:bool, "Create PDF"=w129:bool, "Simulate cRIO"=w31:bool, "Simulate ET3500"=w29:bool, "Use Host COM Port"=w119:bool, "Show LabVIEW Error"=→"Show LabVIEW Error":bool, "Stop On Final Target Temperature"=w34:bool, "Lite Version"=w32:bool)  [unwired: 2 out]
      "Lite Version" <- w32
      n84 = property on="Tab Body" class="TabCtl (strict)"() -> ("Pages"=w107:refnum<vi>[])  [unwired: 2 in, 2 out]
      n85 = flat-sequence "EXECUTE TAB (13 Controls)" {
        frame #0 {
          w223 = T27."Disabled and Grayed Out" ("Disabled")
          # "Initialize"
          n86 = flat-sequence {
            frame #0 {
              n87 = property on="Variant Allowed" class="Bool (strict)"("Colors [4]"=cluster{"Color Box":u32, "Color Box 2":u32}[] [{"Color Box"=16711680, "Color Box 2"=16711680}, {"Color Box"=9868950, "Color Box 2"=9868950}, {"Color Box"=4934475, "Color Box 2"=4934475}, {"Color Box"=6618880, "Color Box 2"=6618880}], "Value"=TRUE) -> ()  [unwired: 2 in, 2 out]
              "Info." <- T19 {"Variant Allowed +/-"=0.0, "Hold Time (HH:MM)"="00:00", "Hold Temp."="0", "Info. Temperature Units"="°C", "Info. WPS/Ref."="", "Info. Temperature Units 2"="°C", "Variant Allowed"=FALSE} ("Info.")
            }
          }
          n88 = control-ref of="ET3504 Status"() -> (w222:refnum<vi>)
          n89 = property class="Str"(reference=w222, "Text.BG Color"=u32 16777216 ("ET3500 Transparent Color")) -> ()  [unwired: 1 in, 2 out]
          n90 = control-ref of="cRIO Status"() -> (w219:refnum<vi>)
          n91 = property class="Str"(reference=w219, "Text.BG Color"=u32 16777216 ("ET3500 Transparent Color")) -> ()  [unwired: 1 in, 2 out]
          n92 = flat-sequence {
            frame #0 {
              n93 = property on="% Hold. Time Completed" class="Slide (strict)"("Scale.Maximum"=100.0 ("Scale.Range:Maximum"), "Scale.Minimum"=0.0 ("Scale.Range:Minimum"), "Fill Color"=u32 16777216 ("Color Box 2"), "Value"=0.0 ("% Hold Time Completed")) -> ()  [unwired: 2 in, 2 out]
              "% Hold. Time Completed" <- 0.0 ("% Hold Time Completed")
            }
          }
          n94 = flat-sequence {
            frame #0 {
              w232 = 12  # 12 Probes Max
              n95 = property on="Chart" class="WFChart (strict)"("History Data"=dynamicdata[] [[{"t0"=timestamp(3471350400 s since 1904-01-01), "dt"=1.0, "Y"=[0.0, 0.0]}]]) -> ()  [unwired: 2 in, 2 out]
              n96 = for {
                N: w232 -> [_]
                i -> [w235]
                n97 = property on="Chart" class="WFChart (strict)"("Active Plot"=w235, "Plot.Plot Name"="") -> ()  [unwired: 2 in, 2 out]
              }
            }
          }
          n98 = property on="Recipe Start" class="Bool"("DisabledEnum"=w223) -> ()  [unwired: 2 in, 2 out]
          n99 = property on="Recipe Stop" class="Bool"("DisabledEnum"=w223) -> ()  [unwired: 2 in, 2 out]
          "Transaction No 2" <- "" ("Transaction No 2")
          "Key Values" <- T9 {"Recording Duration"=0.0, "Remaining Hold Time"=0.0, "Current Temp"=0.0, "Key Values Temperature Units"="°C"} ("Key Values")
          "ET3504 Status" <- "Offline." ("ET3500 Program Status")
          "cRIO Status" <- "Offline." ("cRIO Status")
          "Raw Data File" <- "" ("Raw Data File")
          "Process Completed" <- FALSE ("Overall Status")
          "Hold Time Completed" <- FALSE ("Hold Time Completed")
          "No. of Items" <- 0 ("No. of Items")
        }
      }
      n100 = flat-sequence "RSS Copyright" {
        frame #0 {
          # "Copyright (c) 2014, Reinehold Systems Solutions Pte Ltd. All Rights Reserved.\n\nThis application code (VI) is confidential and/or proprietary and is intended for the express use of the copyright owner and/or IP owner. This code is delivered as part of the Stress Relief Recording System. Any unauthorized re-use of this code outside of the Stress Relief Recording System is prohibited and punishable by law."
        }
      }
      n101 = for {
        tunnel: w177 -> [w329] mode=indexing
        tunnel: w166 -> [w328]
        tunnel: i32[] [19, 3, 3] -> [w327] mode=indexing
        tunnel: string[][] [] ("Item Names") -> [w326]
        w331 = T21 {"Row"=-1, "Column"=-2}  # All ColHdrs
        w332 = T21 {"Row"=-2, "Column"=-2}  # All Rows & Columns (Including Headers)
        n102 = property on="Property Node" class="MCListbox (strict)"(reference=w329, "ActiveCell"=w332, "CellBG"=w328, "ActiveCell"=w331, "CellBG"=u32 12105912, "ItemNames"=w326, "NumCols"=w327) -> ()  [unwired: 1 in, 2 out]
      }
      n103 = for {
        tunnel: w87 -> [w263]
        tunnel: w86 -> [w262] mode=indexing
        tunnel: [w253] -> _
        w260 = refnum<vi> refnum  # Path
        # "Host Paths"
        n104 = property class="Ctl"(reference=w262) -> (reference out=w259:refnum<vi>, "Label.Text"=w261:string)  [unwired: 1 in, 1 out]
        n105 = String To Path(string=w263) -> (path=w252:path)
        n106 = Build Path(base path=w252, name or relative path=w261) -> (appended path=w254:path)
        n107 = To More Specific Class(target class=w260, reference=w259) -> (specific class reference=w258:refnum<vi>)  [unwired: 1 in, 1 out]
        n108 = property class="Path"(reference=w258, "Value"=w254) -> ()  [unwired: 1 in, 2 out]
        n109 = call <vilib>:"Check if File or Folder Exists.vi"("path"=w254) -> ("error out"=w255:errorcluster, "file or folder exists?"=w257:bool, "dup path"=w256:path)  [unwired: 8 in]
        n110 = case shown="False" w257 {
          tunnel: w256 -> [w267 w269]
          tunnel: [w266 w269] -> _
          tunnel: [w265 w268] -> w253
          tunnel: w255 -> [w264 w268]
          frame False {
            # "Create Folder if NOT found\nCreate NEW"
            n111 = Create Folder(path (use dialog)=w267, error in=w264) -> (created path=w266:path, error out=w265:errorcluster)  [unwired: 1 in, 1 out]
          }
          frame True {
            # "Folder Found"
          }
        }
      }
      n112 = for {
        tunnel: w107 -> [w275] mode=indexing
        tunnel: w27 -> [w274]
        tunnel: w32 -> [w271]
        (unwired) "Debug" ("y")
        n113 = property class="Page"(reference=w275) -> (reference out=w270:refnum<vi>, "PageLabel"=w273:string)  [unwired: 1 in, 1 out]
        n114 = case shown="\"Execute\", \"Setup\", Default" w273 {
          tunnel: w274 -> [_ w278 _]
          tunnel: [w276 w278 TRUE] -> w272
          tunnel: w271 -> [w277 _ _]
          frame "Execute", "Setup", Default {
            # "If Lite Version\nthese TAB will be hidden"
            n115 = Not(x=w277) -> (.not. x?=w276:bool)
          }
          frame "Debug" {
            # "Debug dependent of \"Show Report Tab ONLY\""
          }
          frame "Master Data", "Report" {
            # "These Tabs ALWAYS shown"
          }
        }
        n116 = property class="Page"(reference=w270, "PageVis"=w272) -> ()  [unwired: 1 in, 2 out]
      }
      n117 = for {
        tunnel: w89 -> [w319]
        tunnel: w97 -> [w318] mode=indexing
        tunnel: [w309] -> w146
        w316 = refnum<vi> refnum  # Path
        # "Paths"
        n118 = property class="Ctl"(reference=w318) -> (reference out=w315:refnum<vi>, "Label.Text"=w317:string)  [unwired: 1 in, 1 out]
        n119 = String To Path(string=w319) -> (path=w308:path)
        n120 = Build Path(base path=w308, name or relative path=w317) -> (appended path=w310:path)
        n121 = To More Specific Class(target class=w316, reference=w315) -> (specific class reference=w314:refnum<vi>)  [unwired: 1 in, 1 out]
        n122 = property class="Path"(reference=w314, "Value"=w310) -> ()  [unwired: 1 in, 2 out]
        n123 = call <vilib>:"Check if File or Folder Exists.vi"("path"=w310) -> ("error out"=w311:errorcluster, "file or folder exists?"=w313:bool, "dup path"=w312:path)  [unwired: 8 in]
        n124 = case shown="False" w313 {
          tunnel: w312 -> [w323 w325]
          tunnel: [w322 w325] -> _
          tunnel: [w321 w324] -> w309
          tunnel: w311 -> [w320 w324]
          frame False {
            # "Create Folder if NOT found\nCreate NEW"
            n125 = Create Folder(path (use dialog)=w323, error in=w320) -> (created path=w322:path, error out=w321:errorcluster)  [unwired: 1 in, 1 out]
          }
          frame True {
            # "Folder Found"
          }
        }
      }
      n126 = Search and Replace String(input string="ni.var.psp://cRIO IP/RT Library" ("String"), search string="cRIO IP" ("String"), replace string=w120) -> (result string=→"cRIO shared variable RT Library":string)  [unwired: 5 in, 3 out]
      n127 = Search and Replace String(input string="visa://cRIO IP/ASRL1::INSTR" ("String"), search string="cRIO IP" ("String"), replace string=w120) -> (result string=w117:string)  [unwired: 5 in, 3 out]
      "cRIO COM Port" <- w117
      n128 = String To Path(string=w36) -> (path=→"Latest stp file":path)
      n129 = local write "Report.Create.Excel"(w130) -> ()
      n130 = local write "Report.Create.PDF"(w129) -> ()
      n131 = local write "Use Local COM Port"(w119) -> ()
      n132 = property on="CompactRIO Module Details" class="MCListbox (strict)"("ItemNames"=w139) -> ()  [unwired: 2 in, 2 out]
      n133 = Decimal String To Number(string=w95) -> (number=→"cRIO Data Retention":i32)  [unwired: 2 in, 1 out]
      n134 = Decimal String To Number(string=w138) -> (number=→"Running Number":i32)  [unwired: 2 in, 1 out]
      n135 = Fract/Exp String To Number(string=w125) -> (number=w124:dbl)  [unwired: 3 in, 1 out]
      n136 = Fract/Exp String To Number(string=w111, default (0 dbl)=0.0) -> (number=→"Host Sampling Interval (s)":dbl)  [unwired: 2 in, 1 out]
      n137 = property on="Variant Allowed +/-" class="DigNum (strict)"("Value"=w124) -> ()  [unwired: 2 in, 2 out]
      n138 = local write "Stop On Final Target Temperature"(w34) -> ()
      n139 = property on="Property Node" class="MCListbox (strict)"(reference=w39) -> (reference out=w38:refnum<vi>, "NumCols"=w37:u32)  [unwired: 1 in, 1 out]
      n140 = control-ref of="Master Data Temperature Units"() -> (w159:refnum<vi>)
      n141 = control-ref of="Key Values Temperature Units"() -> (w158:refnum<vi>)
      n142 = control-ref of="WPS Details Temperature Units"() -> (w157:refnum<vi>)
      n143 = control-ref of="Info. Temperature Units"() -> (w155:refnum<vi>)
      n144 = control-ref of="Info. Temperature Units 2"() -> (w154:refnum<vi>)
      n145 = control-ref of="FHS Ramp Rate Units"() -> (w134:refnum<vi>)
      n146 = control-ref of="FHS Target Temp Units"() -> (w133:refnum<vi>)
      n147 = control-ref of="MasterData FHS Ramp Rate Temp Units"() -> (w132:refnum<vi>)
      n148 = control-ref of="MasterData FHS Target Temp Units"() -> (w131:refnum<vi>)
      n149 = Bundle("Channel to Probe Mapping"=w136) -> (w84:cluster{"Channel to Probe Mapping":string})  [unwired: 1 in]
      n150 = Select(t=w118, s=w119, f=w117) -> (s? t:f=→"VISA resource name RS232":string)
      n151 = property on="Data" class="Path"(error in=w146) -> (error out=w112:errorcluster, "Value"=w147:path)  [unwired: 1 in, 1 out]
      n152 = property on="Channel to Probe Mapping" class="Clust (strict)"("Value"=w84) -> ()  [unwired: 2 in, 2 out]
      n153 = property on="Setup Load Debug" class="Bool"("Visible"=TRUE) -> ()  [unwired: 2 in, 2 out]
      n154 = flat-sequence {
        frame #0 {
          w192 = 60 ("y")
          # "Initialize Report Tab"
          n155 = Get Date/Time In Seconds() -> (seconds since 1Jan1904=w195:timestamp)
          n156 = Multiply(x=7, y=24) -> (x*y=w190:i32)
          n157 = Multiply(x=w190, y=w192) -> (x*y=w191:i32)
          n158 = property on="Selection Transaction No" class="Str"("Value"="009.*") -> ()  [unwired: 2 in, 2 out]
          n159 = Multiply(x=w191, y=w192) -> (x*y=w193:i32)
          n160 = Subtract(x=w195, y=w193) -> (x-y=w194:timestamp)
          n161 = property on="Date End" class="AbsTime (strict)"("Value"=w195) -> ()  [unwired: 2 in, 2 out]
          n162 = property on="Date Start" class="AbsTime (strict)"("Value"=w194) -> ()  [unwired: 2 in, 2 out]
        }
      }
      n163 = case shown="True" w32 {
        tunnel: [T1."Setup" ("Tab Body") T1."Report" ("Tab Body")] -> w33
        tunnel: w31 -> [w198 _]
        tunnel: [w198 w201] -> w30
        tunnel: w29 -> [w197 _]
        tunnel: [w197 w201] -> w28
        frame False {
          # "Full Version"
          n164 = property on="Tab Setup" class="TabCtl (strict)"("Value"=enum32{"Part Details", "Furnace Settings"}."Part Details" ("Tab Setup")) -> ()  [unwired: 2 in, 2 out]
        }
        frame True {
          w201 = TRUE ("Simulate cRIO")
          # "Lite Version"
        }
      }
      n165 = property on="Raw Data File" class="Path"(error in=w112, "StartPath"=w147) -> ()  [unwired: 1 in, 2 out]
      n166 = for {
        N: w37 -> [_]
        tunnel: "CellBG New Cells" -> [w204]
        tunnel: w38 -> [w203]
        i -> [w206]
        n167 = Bundle("Multicolumn Listbox"=0, w206) -> (w205:cluster{"Multicolumn Listbox":i32, i32})  [unwired: 1 in]
        n168 = property on="Property Node" class="MCListbox (strict)"(reference=w203, "ActiveCell"=w205, "CellBG"=w204) -> ()  [unwired: 1 in, 2 out]
      }
      n169 = Concatenate Strings("Temperature " ("string"), w68) -> (w67:string)
      n170 = Build Array(w159, w158, w157, w155, w154, w134, w133, w132, w131) -> (w156:refnum<vi>[])
      n171 = property on="Chart" class="WFChart (strict)"("YScale.NameLbl.Text"=w67) -> ()  [unwired: 2 in, 2 out]
      n172 = for {
        tunnel: w156 -> [w296] mode=indexing
        tunnel: w68 -> [w295]
        n173 = property class="Str"(reference=w296, "Value"=w295) -> ()  [unwired: 1 in, 2 out]
      }
      n174 = local write "Simulate cRIO"(w30) -> ()
      n175 = local write "Simulate ET3500"(w28) -> ()
      n176 = Obtain Queue(max queue size (-1, unlimited)=10, name (unnamed)="MessageQ", element data type="", error in (no error)=w179) -> (queue out=w182:refnum<queue>, error out=w180:errorcluster)  [unwired: 1 in, 1 out]
      n177 = property on="Tab Body" class="TabCtl (strict)"("Value"=w33) -> ()  [unwired: 2 in, 2 out]
      n178 = Enqueue Element(queue=w182, element=w100, error in (no error)=w180) -> (queue out=w181:refnum<queue>, error out=w178:errorcluster)  [unwired: 1 in, 1 out]
      "Transaction No" <- "" ("Transaction No 2")
      "Recipe Start Flag" <- FALSE ("Recipe Start Flag")
      "Recipe Stop Flag" <- FALSE ("Recipe Stop Flag")
      "Quit Flag" <- FALSE ("Quit Flag")
      "Show Debug Tab" <- w27
      "Show Scrollbars" <- w27
    }
  }
  n179 = Initialize Array("", w19) -> (w18:string[])
  n180 = while {
    tunnel: w17 -> [w340]
    shift-right: [w360] -> _
    shift-left: w18 -> [w362]
    shift-right: [w348] -> w15
    shift-left: _ -> [w347]
    shift-right: [w346] -> w14
    shift-left: _ -> [w345]
    tunnel: w13 -> [w341]
    tunnel: [w338] -> w12
    tunnel: [w333] -> w2
    i -> [w352]
    stop <- w333 stop-if-true
    # "Event Structure For MessageQ"
    n181 = Dequeue Element(queue=w340, error in (no error)=w341) -> (element=w335:string, error out=w339:errorcluster)  [unwired: 1 in, 2 out]
    n182 = flat-sequence {
      tunnel: w352 -> [w414]
      tunnel: [w409] -> w359
      tunnel: w339 -> [w408]
      tunnel: [w408] -> w354
      tunnel: [w407] -> w351
      frame #0 {
        # "SERIAL No + Time Stamp"
        n183 = Format Date/Time String(time format string (%c)="%Y%m%d_%H%M%S") -> (date/time string=w407:string)  [unwired: 2 in]
        n184 = Format Into String(format string="%06d", w414) -> (resulting string=w411:string)  [unwired: 2 in, 1 out]
        n185 = Concatenate Strings(w411, "\t", w407) -> (w409:string)
      }
    }
    n186 = case shown="0" w352 {
      tunnel: w351 -> [w387 _]
      tunnel: [w378 w399] -> w350
      tunnel: [w384 w398] -> w349
      tunnel: w347 -> [_ w399]
      tunnel: w345 -> [_ w398]
      tunnel: w340 -> [w371 _]
      frame 0 {
        w375 = "\"" ("string")
        # "Create .log Event File for 1st and only time"
        n187 = local read "Logs_Host"() -> (w367:path)
        n188 = Format Date/Time String(time format string (%c)="%Y\\%m") -> (date/time string=w370:string)  [unwired: 2 in]
        n189 = Build Path(base path=w367, name or relative path=w370) -> (appended path=w368:path)
        n190 = call <vilib>:"Check if File or Folder Exists.vi"("path"=w368) -> ("error out"=w381:errorcluster, "file or folder exists?"=w383:bool, "dup path"=w382:path)  [unwired: 8 in]
        n191 = case shown="False" w383 {
          tunnel: w382 -> [w395 w397]
          tunnel: [w394 w397] -> w380
          tunnel: [w393 w396] -> w379
          tunnel: w381 -> [w392 w396]
          frame False {
            # "Create Folder if NOT found\nCreate NEW"
            n192 = Create Folder(path (use dialog)=w395, error in=w392) -> (created path=w394:path, error out=w393:errorcluster)  [unwired: 1 in, 1 out]
          }
          frame True {
            # "Folder Found"
          }
        }
        n193 = Concatenate Strings(w387, ".log" ("string")) -> (w385:string)
        n194 = Build Path(base path=w380, name or relative path=w385) -> (appended path=w374:path)
        n195 = Open/Create/Replace File(file path (use dialog)=w374, error in=w379, operation (0:open)=T28."replace or create", access (0:read/write)=enum16{"read/write", "read-only", "write-only"}."write-only") -> (refnum out=w378:refnum<file>, error out=w384:errorcluster)  [unwired: 2 in, 1 out]
        n196 = Not A Number/Path/Refnum?(number/path/refnum=w378) -> (NaN/Path/Refnum?=w377:bool)
        n197 = case shown="True" w377 {
          tunnel: [" Event File Created." ("string") " Event File Not Created." ("string")] -> w373
          frame False {
            # "File Load OK"
          }
          frame True {
            # "File Not Loaded"
          }
        }
        n198 = Path To String(path=w374) -> (string=w376:string)
        n199 = Concatenate Strings(w375, w376, w375, w373) -> (w372:string)
        n200 = Enqueue Element(queue=w371, element=w372) -> ()  [unwired: 2 in, 3 out]
      }
      frame 1, Default {
      }
    }
    n201 = call <vilib>:"Search and Replace Pattern.vi"("string"=w335, "regular expression (\"\")"="\n", "replace all? (F)"=TRUE) -> ("result string"=w334:string)  [unwired: 2 in, 1 out]
    n202 = case shown="No Error" w354 {
      selector: w354 -> [w400 w401]
      tunnel: [_ w402] -> w357
      tunnel: [w400 w401] -> w338
      frame No Error {
      }
      frame Error {
        n203 = Unbundle By Name(w401) -> ("source"=w406:string)
        n204 = Concatenate Strings("\t" ("string"), "[ERROR " ("format string"), w406, "]" ("string")) -> (w402:string)
      }
    }
    n205 = Rotate 1D Array(1:w362, 2:1 ("n")) -> (0:w365:string[])
    n206 = Match Pattern "QUIT is ISSUED"(string=w334, regular expression="QUIT") -> (offset past match=w355:i32)  [unwired: 1 in, 3 out]
    n207 = Concatenate Strings(w359, "\t" ("string"), w334, w357) -> (w344:string)
    n208 = Greater Or Equal To 0?(x=w355) -> (x >= 0?=w353:bool)
    n209 = Replace Array Subset(array=w365, new element=w344) -> (w360:string[])  [unwired: 1 in]
    n210 = Concatenate Strings(w344, "\n" ("delimiter (Tab)")) -> (w342:string)
    n211 = Array To Spreadsheet String(delimiter (Tab)="\n", array=w360, 3:"" ("format string")) -> (spreadsheet string=→"MessageQ":string)
    n212 = Write to Text File(file (use dialog)=w350, text=w342, error in=w349) -> (refnum out=w348:refnum<file>, error out=w346:errorcluster)  [unwired: 1 in, 1 out]
    n213 = Or(x=w338, y=w353) -> (x .or. y?=w333:bool)
  }
  "MessageQ Error" <- w12
  n214 = while {
    tunnel: [w429] -> w23
    tunnel: w17 -> [w428]
    shift-right: [w425] -> _
    shift-left: FALSE -> [w426]
    stop <- w429 stop-if-true
    w427 = 1000  # Timeout for MessageQ
    # "Event Structure For UIEvents"
    n215 = control-ref of="Part Details"() -> (w417:refnum<vi>)
    n216 = control-ref of="MCListBox FHS Setup"() -> (w424:refnum<vi>)
    n217 = control-ref of="MCListBox AWPS"() -> (w423:refnum<vi>)
    n218 = control-ref of="CompactRIO Module Details"() -> (w422:refnum<vi>)
    n219 = control-ref of="WPS Details Setup"() -> (w419:refnum<vi>)
    n220 = control-ref of="Additional WPS/Ref"() -> ()  [unwired: 1 out]
    n221 = control-ref of="Furnace Calibration"() -> (w420:refnum<vi>)
    n222 = control-ref of="Channel to Probe Mapping"() -> (w416:refnum<vi>)
    n223 = local read "MCListBox Ref"() -> (w415:refnum<vi>[])
    n224 = Build Array "Part Details \nMCListbox"(w417, w424, w423, w422) -> (w421:refnum<vi>[])
    n225 = Build Array "Part Details\nClusters"(w419, w420, w416) -> (w418:refnum<vi>[])
    n226 = event shown="[8] \"Setup Load Debug\": Value Change" {
      selector: _ -> [_ _ _ _ _ _ _ _ _ _ _ _ _ _ _ _ _ _ _ _ _ _ _ _ _ _ _ _ _ _ _ _ _ _ _ _ _ _ _ _ _ _ _ _ _ _ _ _ _ _ _]
      dyn-events: _ -> [_ _ _ _ _ _ _ _ _ _ _ _ _ _ _ _ _ _ _ _ _ _ _ _ _ _ _ _ _ _ _ _ _ _ _ _ _ _ _ _ _ _ _ _ _ _ _ _ _ _ _]
      timeout: _ -> [_ _ _ _ _ _ _ _ _ _ _ _ _ _ _ _ _ _ _ _ _ _ _ _ _ _ _ _ _ _ _ _ _ _ _ _ _ _ _ _ _ _ _ _ _ _ _ _ _ _ _]
      tunnel: [_ _ w441 _ _ _ _ _ _ _ _ _ _ _ _ _ _ _ _ _ _ _ _ _ _ _ _ _ _ _ _ _ _ _ _ _ _ _ _ _ _ _ _ _ _ _ _ _ _ _ _] -> w429
      tunnel: w428 -> [_ _ w444 _ w472 w488 w529 w560 w752 _ w795 w820 _ _ w848 w919 w966 _ _ _ _ _ _ _ _ _ _ _ _ _ _ _ _ _ _ _ _ w1567 _ _ _ _ _ _ _ _ w1929 _ _ _ _]
      tunnel: w427 -> [_ _ w443 _ w471 w489 w528 w568 w751 _ w796 w821 _ _ w849 w920 w967 _ _ _ _ _ _ _ _ _ _ _ _ _ _ _ _ _ _ _ _ w1568 _ _ _ _ _ _ _ _ w1930 _ _ _ _]
      tunnel: w426 -> [_ _ _ _ _ _ _ _ _ _ _ _ _ _ _ _ _ _ _ w1174 _ _ _ _ _ _ _ _ _ _ _ _ _ _ _ _ _ _ _ _ _ _ _ _ _ _ _ _ _ _ _]
      tunnel: [_ _ _ _ _ _ _ _ _ _ _ _ _ _ _ _ _ _ _ TRUE _ _ _ _ _ _ _ _ _ _ _ _ _ _ _ _ _ _ _ _ _ _ _ _ _ _ _ _ _ _ _] -> w425
      tunnel: w421 -> [_ _ _ _ _ _ _ w556 w728 _ _ _ _ _ _ _ w993 _ _ _ _ _ _ _ _ _ _ _ _ _ _ _ _ _ _ _ _ _ _ _ _ _ _ _ _ _ _ _ _ _ _]
      tunnel: w418 -> [_ _ _ _ _ _ _ w565 _ _ _ _ _ _ _ _ w979 _ _ _ _ _ _ _ _ _ _ _ _ _ _ _ _ _ _ _ _ _ _ _ _ _ _ _ _ _ _ _ _ _ _]
      tunnel: w417 -> [_ _ _ _ _ _ _ _ _ _ _ _ _ _ _ _ _ _ _ _ _ _ _ _ _ _ w1444 _ _ _ _ _ _ _ _ _ _ _ _ _ _ _ _ _ _ _ _ _ _ _ _]
      tunnel: w415 -> [_ _ _ _ _ _ _ _ _ _ _ _ _ _ _ _ _ _ w1151 _ _ _ _ _ _ _ _ _ _ _ _ _ _ _ _ _ _ _ _ _ _ _ _ _ _ _ _ _ _ _ _]
      event Timeout {
        n227 = event-data() -> ()  [unwired: 1 in, 3 out]
      }
      event "Tab Body": Value Change {
        n228 = event-data() -> ("NewVal"=w430:T1)  [unwired: 1 in, 5 out]
        n229 = case shown="\"Report\"" w430 {
          frame "Setup", Default {
          }
          frame "Report" {
            # "Search 7 days ahead"
            n230 = flat-sequence {
              frame #0 {
                w435 = 60 ("y")
                # "Initialize Report Tab"
                n231 = Get Date/Time In Seconds() -> (seconds since 1Jan1904=w438:timestamp)
                n232 = Multiply(x=7, y=24) -> (x*y=w433:i32)
                n233 = Multiply(x=w433, y=w435) -> (x*y=w434:i32)
                n234 = property on="Selection Transaction No" class="Str"("Value"="009.*") -> ()  [unwired: 2 in, 2 out]
                n235 = Multiply(x=w434, y=w435) -> (x*y=w436:i32)
                n236 = Subtract(x=w438, y=w436) -> (x-y=w437:timestamp)
                n237 = property on="Date End" class="AbsTime (strict)"("Value"=w438) -> ()  [unwired: 2 in, 2 out]
                n238 = property on="Date Start" class="AbsTime (strict)"("Value"=w437) -> ()  [unwired: 2 in, 2 out]
              }
            }
          }
        }
      }
      event "Close", "Debug Close": Value Change {
        n239 = event-data() -> ()  [unwired: 1 in, 6 out]
        n240 = case shown="True" "Debug Close" {
          tunnel: [w447 "[Debug CLOSE]." ("string")] -> w442
          tunnel: [w445 w457] -> w441
          frame False {
            n241 = flat-sequence {
              tunnel: [w454] -> w453
              tunnel: "Close" -> [w454]
              tunnel: w453 -> [_]
              frame #0 {
                n242 = Wait (ms)(milliseconds to wait=u32 100) -> ()  [unwired: 1 out]
              }
              frame #1 {
                n243 = local write "Close"(FALSE ("Quit")) -> ()
              }
            }
            n244 = Two Button Dialog(message="Confirm Close?") -> (T button?=w445:bool)  [unwired: 2 in]
            n245 = local write "Quit Flag"(w445) -> ()
            n246 = Select(t="Confirm." ("string"), s=w445, f="Cancel." ("string")) -> (s? t:f=w449:string)
            n247 = Concatenate Strings("[CLOSE] Clicked By User. " ("string"), w449) -> (w447:string)
          }
          frame True {
            w457 = TRUE ("T button?")
            n248 = local write "Quit Flag"(w457) -> ()
          }
        }
        n249 = Enqueue Element(queue=w444, element=w442, timeout in ms (-1)=w443) -> ()  [unwired: 1 in, 3 out]
      }
      event Key Down? {
        # "Disables comma in the entire program"
        n250 = event-data() -> ("Char"=w460:i16)  [unwired: 1 in, 9 out]
        n251 = case shown="44, 47, 92" w460 {
          tunnel: [_ TRUE] -> w459
          frame 0, Default {
          }
          frame 44, 47, 92 {
            # "Discard"
          }
        }
        n252 = event-data("Discard?"=w459) -> ()  [unwired: 1 in, 1 out]
      }
      event "Data", "Excel", "Report.Create.Excel", "Report.Create.PDF", "Simulate cRIO", "Simulate ET3500": Value Change {
        # "<OPTIONS> are logged into MessageQ"
        n253 = event-data() -> ("CtlRef"=w470:refnum<vi>)  [unwired: 1 in, 5 out]
        n254 = property class="Ctl"(reference=w470) -> ("ClassName"=w462:string, "Caption.Text"=w463:string, "Value"=w467:variant)  [unwired: 1 in, 2 out]
        n255 = case shown="\"Boolean\"" w462 {
          tunnel: w467 -> [w478 w484]
          tunnel: [w473 w479] -> w466
          frame "Path", Default {
            w474 = "\"" ("string")
            n256 = Variant To Data(type=path "", Variant=w478) -> (data=w476:path)  [unwired: 1 in, 1 out]
            n257 = Path To String(path=w476) -> (string=w475:string)
            n258 = Concatenate Strings(w474, w475, w474) -> (w473:string)
          }
          frame "Boolean" {
            n259 = Variant To Data(type=TRUE, Variant=w484) -> (data=w482:bool)  [unwired: 1 in, 1 out]
            n260 = Select(t="TRUE" ("string"), s=w482, f="FALSE" ("string")) -> (s? t:f=w479:string)
          }
        }
        n261 = Concatenate Strings("<", w463, ">", " changed to " ("string"), w466) -> (w468:string)
        n262 = Enqueue Element(queue=w472, element=w468, timeout in ms (-1)=w471) -> ()  [unwired: 1 in, 3 out]
      }
      event "cRIO Set Time": Value Change {
        n263 = event-data() -> ()  [unwired: 1 in, 6 out]
        n264 = call "Password to adjust CompactRIO internal Clock"() -> ("Password"=w490:string, "OK"=w491:bool)  [unwired: 17 in, 1 out]
        n265 = case shown="True" w491 {
          tunnel: w490 -> [_ w494]
          tunnel: ["Cancelled.\n" ("message") w493] -> w487
          frame False {
          }
          frame True {
            n266 = case shown="\"3504\"" w494 {
              tunnel: [w495 "Password OK.\n"] -> w493
              frame "False", Default {
                w495 = "Wrong Password.\n" ("message")
                n267 = One Button Dialog(message=w495) -> ()  [unwired: 1 in, 1 out]
              }
              frame "3504" {
                n268 = local read "Simulate cRIO"() -> (w497:bool)
                n269 = case shown="False" w497 {
                  selector: w497 -> [w507 _]
                  tunnel: [w508 _] -> _
                  frame False {
                    n270 = Get Date/Time In Seconds() -> (seconds since 1Jan1904=w501:timestamp)
                    n271 = local read "cRIO IP"() -> (w512:string)
                    n272 = call <vilib>:"Initialize Session.vi"("connect timeout in ms (4s)"=u32 1000, "force property refresh (T)"=FALSE, "target (localhost)"=w512) -> ("error out"=w516:errorcluster, "session out"=w517:refnum<k21>)  [unwired: 7 in]
                    n273 = local read "cRIO shared variable RT Library"() -> (w498:string)
                    n274 = Multiply(x=60, y=60) -> (x*y=w504:i32)
                    n275 = Multiply(x=w504, y=7) -> (x*y=w502:i32)
                    n276 = Subtract(x=w501, y=w502) -> (x-y=w500:timestamp)
                    n277 = call <vilib>:"Set Time.vi"("error in (no error)"=w516, "time"=w500, "session in (localhost)"=w517) -> ("error out"=w515:errorcluster, "session out"=w518:refnum<k21>)  [unwired: 5 in, 2 out]
                    n278 = call-poly <vilib>:"Close.vi"("error in (no error)"=w515, "session in"=w518) -> ("error out"=w509:errorcluster)  [unwired: 9 in]
                    n279 = local read "cRIO Data Retention"() -> (w511:i32)
                    n280 = control-ref of="cRIO Status"() -> (w499:refnum<vi>)
                    n281 = call "cRIO - Shared Variable RW.vi"("shared variable RT Library"=w498, "Read/Write"=enum16{"Write", "Read", "Write TimeStamp"}."Write TimeStamp", 2:w501, "Error In"=w509, "Simulate cRIO"=w507, "cRIO Data Retention"=w511, "cRIO Status"=w499) -> ("Error Out"=w508:errorcluster)  [unwired: 4 in, 8 out]
                  }
                  frame True {
                    n282 = One Button Dialog(message="cRIO Simulate Set Time OK.") -> ()  [unwired: 1 in, 1 out]
                  }
                }
              }
            }
          }
        }
        n283 = Concatenate Strings("[cRIO Set Time] Clicked by User. " ("element"), w487) -> (w485:string)
        n284 = Enqueue Element(queue=w488, element=w485, timeout in ms (-1)=w489) -> ()  [unwired: 1 in, 3 out]
      }
      event "Recipe Stop", "Recipe Start": Value Change {
        # "[BUTTON ACTIONS] are logged into MessageQ"
        n285 = event-data() -> ("CtlRef"=w527:refnum<vi>)  [unwired: 1 in, 5 out]
        n286 = property class="Bool"(reference=w527) -> ("Label.Text"=w524:string)  [unwired: 1 in, 2 out]
        n287 = local write "Recipe Start Flag"("Recipe Start") -> ()
        n288 = local write "Recipe Stop Flag"("Recipe Stop") -> ()
        n289 = Concatenate Strings("[" ("string"), w524, "]" ("string"), " Clicked By User." ("string")) -> (w522:string)
        n290 = Enqueue Element(queue=w529, element=w522, timeout in ms (-1)=w528) -> ()  [unwired: 1 in, 3 out]
      }
      event "Setup Save": Value Change {
        n291 = event-data() -> ()  [unwired: 1 in, 1 out]
        n292 = Index Array "MCListBox Part Details"(array=w556, index=0) -> (element=w558:refnum<vi>)
        n293 = Index Array "MCListBox FHS Setup"(array=w556, index=1) -> (element=w555:refnum<vi>)
        n294 = property class="MCListbox (strict)"(reference=w555) -> (reference out=w549:refnum<vi>, "ItemNames"=w540:string[][])  [unwired: 1 in, 1 out]
        n295 = property class="MCListbox (strict)"(reference=w558) -> ("ItemNames"=w564:string[][])  [unwired: 1 in, 2 out]
        n296 = Array Size(array=w540) -> (size(s)=w554:i32[])
        n297 = Array Size(array=w564) -> (size(s)=w562:i32[])
        n298 = Index Array(array=w554) -> (element #1=w553:i32, element #2=w552:i32)  [unwired: 2 in]
        n299 = Decrement(x=w553) -> (x-1=w541:i32)
        "FHS Last Row" <- w541
        n300 = Initialize Array("", w552) -> (w550:string[])
        n301 = Index Array(array=w562, index=0) -> (element=w561:i32)
        n302 = Replace Array Subset(array=w540, new element=w550, index (row)=w541) -> (w537:string[][])  [unwired: 1 in]
        n303 = Greater Than 0?(x=w561) -> (x > 0?=w547:bool)
        n304 = local read "WPS Details Setup"() -> (w536:T7)
        n305 = property class="MCListbox (strict)"(reference=w549, "ItemNames"=w537) -> (reference out=w545:refnum<vi>)  [unwired: 1 in, 1 out]
        n306 = Unbundle By Name(w536) -> ("Hold Temperature"=w535:string, "Hold Time (HH:MM)"=w534:string)
        n307 = call "String - Check Hold Parameters.vi"("Master Data Hold Time (HH:MM)"=w534, "Master Data Hold Temperature"=w535, "2D Array in"=w537) -> ("Found"=w533:bool, "Message"=w532:string)  [unwired: 6 in, 1 out]
        n308 = call "String - Check Empty Cells.vi"("ItemNames"=w540) -> ("Empty Cell(s)"=w539:bool)  [unwired: 8 in, 2 out]
        n309 = Greater Than 0?(x=w541) -> (x > 0?=w544:bool)
        n310 = Not(x=w539) -> (.not. x?=w538:bool)
        "All Cells Filled" <- w538
        n311 = Compound Arithmetic op=AND(w538, w547, w544, w533) -> (w548:bool)
        n312 = case shown="True" w548 {
          tunnel: [TRUE w643] -> w569
          tunnel: [_ w637] -> w566
          tunnel: w556 -> [_ w636]
          tunnel: w565 -> [_ w600]
          tunnel: w538 -> [w582 _]
          tunnel: w547 -> [w573 _]
          tunnel: w545 -> [_ w614]
          tunnel: [w583 w615] -> w542
          tunnel: w544 -> [w576 _]
          tunnel: w533 -> [_ _]
          tunnel: w532 -> [w570 _]
          frame False {
            # "Not Valid"
            n313 = Select(t="", s=w573, f="Part Details Table is Empty. \n" ("message")) -> (s? t:f=w575:string)
            n314 = Select(t="", s=w576, f="Furnance Heating Sequence has insufficient Sequences. \n" ("message")) -> (s? t:f=w578:string)
            n315 = Select(t="", s=w582, f="Furnance Heating Sequence contains incomplete Sequence.\n" ("message")) -> (s? t:f=w577:string)
            n316 = Concatenate Strings(w577, w578, w575, w570) -> (w583:string)
          }
          frame True {
            w592 = "Settings" ("section")
            # "All Cells Filled, MCListBox Part Details >0, MCListBox FHS Setup>0, Hold Parameters Valid"
            n317 = local read "VISA resource name RS232"() -> (w613:string)
            n318 = local read "Furnace Number"() -> (w634:string)
            n319 = local read "Running Number"() -> (w631:i32)
            n320 = local read "WPS Details Setup"() -> (w616:T7)
            n321 = local read "Simulate ET3500"() -> (w612:bool)
            n322 = Increment(x=w631) -> (x+1=w619:i32)
            n323 = Format Into String(format string="%05d", w631) -> (resulting string=w632:string)  [unwired: 2 in, 1 out]
            n324 = control-ref of="Parameter Buffer"() -> (w599:refnum<vi>)
            n325 = Format Date/Time String(time format string (%c)="%Y%m%d_%H%M%S") -> (date/time string=w622:string)  [unwired: 2 in]
            n326 = call "ET3500 - Write Program.vi"("Simulate"=w612, 7:TRUE ("subVI"), "MCListBox FHS Setup"=w614, "WPS Details Setup"=w616, "VISA resource name RS232"=w613) -> ("ET3500"=w611:errorcluster, "Final Target Temperture"=w588:i32)  [unwired: 1 in, 4 out]
            n327 = Concatenate Strings("009" ("string"), w634, w632) -> (w610:string)
            n328 = Build Array (concatenate)(w600, w599, w585) -> (w598:refnum<vi>[])
            n329 = flat-sequence {
              tunnel: w588 -> [w647]
              tunnel: [w644] -> w585
              frame #0 {
                n330 = Number To Decimal String(number=w647) -> (decimal integer string=w646:string)  [unwired: 1 in]
                n331 = Bundle(w646) -> (→"Final Target Temperature":cluster{string})  [unwired: 1 in]
                n332 = control-ref of="Final Target Temperature"() -> (w644:refnum<vi>)
              }
            }
            n333 = Concatenate Strings(w610, "_" ("string"), w622, ".stp" ("string")) -> (w642:string)
            n334 = local write "Transaction No 2"(w610) -> ()
            n335 = local write "Transaction No"(w610) -> ()
            n336 = call "Folder - Create Year-Month.vi"("Folder Name"="Setup") -> ("Folder with Year\\Month"=w608:path)  [unwired: 9 in, 1 out]
            n337 = Build Path(base path=w608, name or relative path=w642) -> (appended path=w590:path)
            n338 = call <vilib>:"Open Config Data.vi"("configuration file path"=w590) -> ("error out"=w640:errorcluster, "refnum"=w641:T33)  [unwired: 8 in, 1 out]
            n339 = for {
              tunnel: w641 -> [w680]
              tunnel: w640 -> [w679]
              tunnel: [w678] -> w638
              tunnel: [w677] -> w639
              tunnel: w636 -> [w676] mode=indexing
              n340 = call "Key - MCListbox Write.vi"("error in (no error)"=w679, "MulticolumnListbox Ref in"=w676, "refnum"=w680) -> ("error out"=w677:errorcluster, "Refnum out"=w678:T33)  [unwired: 5 in, 2 out]
            }
            n341 = for {
              tunnel: w598 -> [w675] mode=indexing
              tunnel: w639 -> [w674]
              tunnel: w638 -> [w673]
              tunnel: [w672] -> w587
              tunnel: [w671] -> w586
              n342 = call "Key - Cluster Write.vi"("error in (no error)"=w674, "Cluster Ref in"=w675, "Refnum in"=w673) -> ("error out"=w671:errorcluster, "Refnum out"=w672:T33)  [unwired: 7 in]
            }
            n343 = local write "Latest stp file"(w590) -> ()
            n344 = local write "Running Number"(w619) -> ()
            n345 = call <vilib>:"Application Directory.vi"() -> ("Application Directory"=w628:path)
            n346 = call <vilib>:"Close Config Data.vi"("error in (no error)"=w586, "refnum"=w587) -> ("file path"=w637:path)  [unwired: 8 in, 1 out]
            n347 = Build Path(base path=w628, name or relative path="MyEXE.ini" ("ini Name")) -> (appended path=w626:path)
            n348 = case shown="No Error" w611 {
              tunnel: [w668 "Upload to ET3504 Failed.\nCheck if ET3504 is already Running a Program.\nCheck communication cable to ET3504." ("message")] -> w615
              tunnel: w612 -> [w669 _]
              frame No Error {
                n349 = Select(t="Simulate Upload to ET3504 OK." ("message"), s=w669, f="Upload to ET3504 OK." ("message")) -> (s? t:f=w668:string)
              }
              frame Error {
              }
            }
            n350 = Number To Decimal String(number=w619) -> (decimal integer string=w618:string)  [unwired: 1 in]
            n351 = call <vilib>:"Open Config Data.vi"("create file if necessary (T)"=FALSE, "configuration file path"=w626) -> ("error out"=w630:errorcluster, "refnum"=w629:T33)  [unwired: 7 in, 1 out]
            n352 = Not A Number/Path/Refnum?(number/path/refnum=w637) -> (NaN/Path/Refnum?=w643:bool)
            n353 = Path To String(path=w590) -> (string=w591:string)
            n354 = call-poly <vilib>:"Write Key.vi"("section"=w592, "error in (no error)"=w630, "value"=w618, "key"="Running Number", "refnum"=w629) -> ("error out"=w595:errorcluster, "refnum out"=w597:T33)  [unwired: 4 in, 1 out]
            n355 = call-poly <vilib>:"Write Key.vi"("write raw string? (F)"=TRUE, "section"=w592, "error in (no error)"=w595, "value"=w591, "key"="Latest stp File", "refnum"=w597) -> ("error out"=w594:errorcluster, "refnum out"=w596:T33)  [unwired: 3 in, 1 out]
            n356 = Unbundle By Name("WPS Details Setup") -> ("WPS/Ref"=w605:T5, "WPS Details Temperature Units"=w606:string, "Hold Temperature"=w607:string, "Hold Time (HH:MM)"=w602:string)
            n357 = local write "ET3500 Error"(w611) -> ()
            n358 = call <vilib>:"Close Config Data.vi"("error in (no error)"=w594, "refnum"=w596) -> ()  [unwired: 8 in, 2 out]
            n359 = local read "Info."() -> (w603:T8)
            n360 = Bundle By Name(cluster=w603, "Info. WPS/Ref."=w605, "Info. Temperature Units"=w606, "Info. Temperature Units 2"=w606, "Hold. Temp."=w607, "Hold. Time (hour:minute)"=w602) -> (w601:T8)
            n361 = local write "Info."(w601) -> ()
            n362 = flat-sequence "EXECUTE TAB" {
              tunnel: w601 -> [_]
              frame #0 {
                w650 = timestamp(3471350400 s since 1904-01-01) ("Parameter (Start Dwell Time)")
                # "Clear Data on EXECUTE TAB"
                n363 = property on="Hold. Time (hour:minute)" class="Str"() -> ("Value"=w655:string)  [unwired: 2 in, 2 out]
                n364 = invoke on="Chart" class="WFChart (strict)" method="Reinit To Default"() -> ()  [unwired: 3 in, 3 out]
                n365 = local write "Process Completed"(FALSE ("Overall Status")) -> ()
                n366 = call "String - Format to (HH_colon_MM).vi"("xx:xx"=w655) -> ("seconds"=w656:dbl)  [unwired: 9 in, 1 out]
                n367 = property on="% Hold. Time Completed" class="Slide (strict)"("Scale.Maximum"=100.0 ("Scale.Range:Maximum"), "Scale.Minimum"=0.0 ("Scale.Range:Minimum"), "Fill Color"=u32 16777216 ("Color Box 2"), "Value"=0.0 ("% Hold Time Completed")) -> ()  [unwired: 2 in, 2 out]
                n368 = local write "Hold Time Completed"(FALSE ("Hold Time Completed")) -> ()
                n369 = local write "Parameter (End Dwell Time)"(w650) -> ()
                n370 = local write "Parameter (Start Dwell Time)"(w650) -> ()
                n371 = property on="Recording Duration" class="DigNum (strict)"("Value"=0.0) -> ()  [unwired: 2 in, 2 out]
                n372 = property on="Remaining Hold Time" class="DigNum (strict)"("Value"=w656) -> ()  [unwired: 2 in, 2 out]
                n373 = property on="Variant Allowed" class="Bool (strict)"("Colors [4]"=cluster{"Color Box":u32, "Color Box 2":u32}[] [{"Color Box"=16711680, "Color Box 2"=16711680}, {"Color Box"=9868950, "Color Box 2"=9868950}, {"Color Box"=4934475, "Color Box 2"=4934475}, {"Color Box"=6618880, "Color Box 2"=6618880}], "Value"=TRUE) -> ()  [unwired: 2 in, 2 out]
                n374 = To Double Precision Float(number=w650) -> (double precision float=w652:dbl)
                n375 = Format Into String(w652) -> (resulting string=w651:string)  [unwired: 3 in, 1 out]
                n376 = Bundle By Name(cluster=T14 {"Start Holding Time and Date"="", "End Holding Time and Date"="", "Start Holding Temperature"="", "End Holding Temperature"=""} ("Parameter Buffer"), "Start Holding Time and Date"=w651, "End Holding Time and Date"=w651) -> (w649:T14)
                n377 = local write "Raw Data File"("") -> ()
                n378 = local write "Parameter Buffer"(w649) -> ()
                n379 = property on="Chart" class="WFChart (strict)"("History Data"=dynamicdata[] [[{"t0"=timestamp(3471350400 s since 1904-01-01), "dt"=1.0, "Y"=[0.0, 0.0]}]]) -> ()  [unwired: 2 in, 2 out]
              }
            }
          }
        }
        n380 = case shown="True" w569 {
          tunnel: w566 -> [w691 _]
          tunnel: [w687 w694] -> w546
          tunnel: "[Save Setup]" ("string") -> [w684 w693]
          tunnel: w561 -> [w686 _]
          tunnel: [w686 _] -> w530
          frame False {
            w689 = "\"" ("string")
            # "File Save OK"
            n381 = Path To String(path=w691) -> (string=w690:string)
            n382 = Concatenate Strings(w684, " OK. " ("string"), "\n") -> (w683:string)
            n383 = Concatenate Strings(w683, w689, w690, w689, " saved. " ("string"), "\n") -> (w687:string)
          }
          frame True {
            # "File Save Not OK"
            n384 = Concatenate Strings(w693, " Cancelled. ", "\n") -> (w694:string)
          }
        }
        n385 = Concatenate Strings(w546, "\n", w542) -> (w543:string)
        n386 = Enqueue Element(queue=w560, element=w543, timeout in ms (-1)=w568) -> ()  [unwired: 1 in, 3 out]
        n387 = One Button Dialog(message=w543) -> ()  [unwired: 1 in, 1 out]
        n388 = local write "No. of Items"(w530) -> ()
      }
      event "Setup Load Debug": Value Change {
        w720 = string[] ["TC1", "TC2", "TC3", "TC4", "TC5", "TC6"]  # Channel to Probe Cluster Label
        # "For Debug ONLY"
        n389 = event-data() -> ()  [unwired: 1 in, 6 out]
        n390 = control-ref of="WPS Details Setup"() -> (w703:refnum<vi>)
        n391 = Index Array(array=w728, index #1=0 ("index"), index #2=1 ("index"), index #3=2 ("index")) -> (element #1=w715:refnum<vi>, element #2=w727:refnum<vi>, element #3=w726:refnum<vi>)
        n392 = local read "Setup"() -> (w699:path)
        n393 = Build Array(w715, w727, w726) -> (w725:refnum<vi>[])
        n394 = Format Date/Time String(time format string (%c)="%Y\\%m") -> (date/time string=w698:string)  [unwired: 2 in]
        n395 = local read "Channel to Probe Mapping"() -> (w721:cluster{"Channel to Probe Mapping":string})
        n396 = Unbundle By Name(w721) -> ("Channel to Probe Mapping"=w719:string)
        n397 = Build Array "Part Details\nClusters"(w703) -> (w729:refnum<vi>[])
        n398 = Build Path(base path=w699, name or relative path=w698) -> (appended path=w697:path)
        n399 = call "File Dialog"("start path"=w697, "prompt"="Select SETUP file", "pattern (all files)"="*.stp" ("pattern label")) -> ("selected path"=w742:path, "error out"=w746:errorcluster)  [unwired: 9 in, 2 out]
        n400 = call <vilib>:"Open Config Data.vi"("error in (no error)"=w746, "configuration file path"=w742) -> ("error out"=w745:errorcluster, "refnum"=w747:T33)  [unwired: 7 in, 1 out]
        n401 = Strip Path(path=w742) -> (name=w741:string)  [unwired: 1 out]
        n402 = for {
          tunnel: w725 -> [w764] mode=indexing
          tunnel: w747 -> [w768]
          tunnel: w745 -> [w767]
          tunnel: [w766] -> w744
          tunnel: [w765] -> w743
          n403 = call "Key - MCListbox Read.vi"("error in (no error)"=w767, "New MulticolumnListbox Ref"=w764, "Original MulticolumnListbox Ref"=w764, "refnum"=w768) -> ("error out"=w765:errorcluster, "Refnum out"=w766:T33)  [unwired: 4 in, 2 out]
        }
        n404 = Match Pattern(string=w741, regular expression="[_]") -> (before substring=w735:string)  [unwired: 1 in, 3 out]
        n405 = local write "Transaction No 2"(w735) -> ()
        n406 = local write "Transaction No"(w735) -> ()
        n407 = for {
          tunnel: w729 -> [w759] mode=indexing
          tunnel: w744 -> [w763]
          tunnel: w743 -> [w762]
          tunnel: [w761] -> w736
          tunnel: [w760] -> w737
          n408 = call "Key - Cluster Read.vi"("error in (no error)"=w762, "New Ctl Ref"=w759, "Original Ctl Ref"=w759, "Refnum in"=w763) -> ("error out"=w761:errorcluster, "Refnum out"=w760:T33)  [unwired: 5 in, 1 out]
        }
        n409 = call <vilib>:"Close Config Data.vi"("error in (no error)"=w736, "refnum"=w737) -> ("error out"=w713:errorcluster, "file path"=w748:path)  [unwired: 8 in]
        n410 = property class="MCListbox (strict)"(reference=w715, error in=w713) -> (error out=w701:errorcluster, "ColHdrString"=w714:string[], "ItemNames"=w706:string[][])  [unwired: 1 out]
        n411 = property class="Clust (strict)"(reference=w703, error in=w701) -> (error out=→"Property Node Error":errorcluster, "Value"=w702:T7)  [unwired: 1 out]
        n412 = Array Size(array=w706) -> (size(s)=w705:i32[])
        n413 = Unbundle By Name(w702) -> ("WPS/Ref"=w710:T5, "WPS Details Temperature Units"=w709:string, "Hold Temperature"=w708:string, "Hold Time (HH:MM)"=w707:string)
        n414 = Index Array(array=w705) -> (element=w704:i32)  [unwired: 1 in]
        n415 = call "String - Channel to Probe Mappings.vi"("Channel to Probe Mapping"=w719, "Channel to Probe Cluster Label"=w720, "ColHdrString"=w714, "ItemNames"=w706) -> ("Probe List Valid"=w717:bool, "Probe List"=w718:i32[], "cRIO Channel List"=w716:i32[])  [unwired: 1 in, 4 out]
        n416 = local write "Probe List Valid"(w717) -> ()
        n417 = local write "Probe List"(w718) -> ()
        n418 = local write "No. of Items"(w704) -> ()
        n419 = local write "cRIO Channel List"(w716) -> ()
        n420 = Index Array(array=w728, index #1=1 ("index"), index #2=2 ("index")) -> (element #1=w732:refnum<vi>, element #2=w731:refnum<vi>)
        n421 = Build Array(w732, w731) -> (w730:refnum<vi>[])
        n422 = local read "Info."() -> (w712:T8)
        n423 = Bundle By Name(cluster=w712, "Info. WPS/Ref."=w710, "Info. Temperature Units"=w709, "Info. Temperature Units 2"=w709, "Hold. Temp."=w708, "Hold. Time (hour:minute)"=w707) -> (w711:T8)
        n424 = local write "Info."(w711) -> ()
        n425 = Not A Number/Path/Refnum?(number/path/refnum=w748) -> (NaN/Path/Refnum?=w749:bool)
        n426 = for {
          tunnel: w730 -> [w758] mode=indexing
          tunnel: w713 -> [w757]
          n427 = local read "CellBG Unused Cells"() -> (w754:u32)
          n428 = call "MCListbox Refresh.vi"("Which Cells"=T29."Exisiting and Blank Cells", "Error In"=w757, "color of New Cells"=w754, "color of Blank cells"=w754, "MulticolumnListbox in"=w758) -> ("Error Out"=w755:errorcluster)  [unwired: 5 in, 1 out]
          n429 = local write "Property Node Error"(w755) -> ()
        }
        n430 = case "MessageQ" shown="False" w749 {
          tunnel: w748 -> [w775 _]
          tunnel: [w772 w776] -> w753
          tunnel: "[Load Setup]" ("result string") -> [w770 w778]
          frame False {
            w773 = "\"" ("string")
            # "File Load OK"
            n431 = Path To String(path=w775) -> (string=w774:string)
            n432 = Concatenate Strings(w770, " OK. " ("string"), w773, w774, w773, " loaded." ("string")) -> (w772:string)
          }
          frame True {
            # "File Not Loaded"
            n433 = Concatenate Strings(w778, " Cancelled.") -> (w776:string)
          }
        }
        n434 = Enqueue Element(queue=w752, element=w753, timeout in ms (-1)=w751) -> ()  [unwired: 1 in, 3 out]
      }
      event "Simulate cRIO Started": Value Change {
        n435 = event-data() -> ()  [unwired: 1 in, 6 out]
        n436 = case shown="False" FALSE {
          tunnel: [100 ("Start Temp") 25 ("Start Temp")] -> w783
          tunnel: [i32[][] [[2, 0, 0, 3], [3, 50, 80, 1], [4, 0, 0, 0]] ("Final Segments") i32[][] [[1, 100, 100, 1], [2, 0, 0, 3], [3, 50, 80, 1], [4, 0, 0, 0]] ("Final Segments")] -> w781
          frame False {
            # "From Hold at 100° to Ramp Down"
          }
          frame True {
            # "All Segments (Ramp Up, Hold, Ramp Down)"
          }
        }
        n437 = local read "cRIO shared variable RT Library"() -> (w779:string)
        n438 = control-ref of="cRIO Status"() -> (w786:refnum<vi>)
        n439 = call "cRIO - Shared Variable RW.vi"("shared variable RT Library"=w779, "Read/Write"=enum16{"Write", "Read", "Write TimeStamp"}."Write", "Simulate cRIO"=TRUE, "Probe List In"=i32[] [1, 2], "DAQ Start"=TRUE, "cRIO Status"=w786) -> ()  [unwired: 5 in, 9 out]
        n440 = call "ET3500 - Simulate Profile.vi"("Popup"=FALSE, "Set (T) / Get (F)"=TRUE, 9:30 ("Dwell Time (min)"), "Start Temp"=w783, "Final Segments"=w781) -> ()  [unwired: 2 in, 5 out]
      }
      event "Use Local COM Port": Value Change {
        # "Set COM Port to either Local PC or via cRIO"
        n441 = event-data() -> ("CtlRef"=w807:refnum<vi>)  [unwired: 1 in, 5 out]
        n442 = property class="Bool (strict)"(reference=w807) -> ("Label.Text"=w805:string)  [unwired: 1 in, 2 out]
        n443 = local read "Host COM Port"() -> (w810:string)
        n444 = local read "cRIO COM Port"() -> (w809:string)
        n445 = Select(t="TRUE.", s="Use Local COM Port", f="FALSE.") -> (s? t:f=w800:string)
        n446 = Concatenate Strings("[" ("string"), w805, "]" ("string")) -> (w803:string)
        n447 = Select(t=w810, s="Use Local COM Port", f=w809) -> (s? t:f=w808:string)
        n448 = Concatenate Strings(w803, " is Changed to " ("string"), w800) -> (w797:string)
        n449 = local write "VISA resource name RS232"(w808) -> ()
        n450 = Enqueue Element(queue=w795, element=w797, timeout in ms (-1)=w796) -> ()  [unwired: 1 in, 3 out]
      }
      event "Parameter": Value Change {
        n451 = event-data() -> ()  [unwired: 1 in, 6 out]
        n452 = local read "Latest stp file"() -> (w817:path)
        n453 = control-ref of="Parameter Buffer"() -> (w812:refnum<vi>)
        n454 = call <vilib>:"Open Config Data.vi"("create file if necessary (T)"=FALSE, "configuration file path"=w817) -> ("error out"=w819:errorcluster, "refnum"=w816:T33)  [unwired: 7 in, 1 out]
        n455 = call "Key - Cluster Read.vi"("error in (no error)"=w819, "New Ctl Ref"=w812, "Original Ctl Ref"=w812, "Refnum in"=w816) -> ("error out"=w818:errorcluster, "Refnum out"=w814:T33)  [unwired: 5 in, 1 out]
        n456 = call <vilib>:"Close Config Data.vi"("error in (no error)"=w818, "write file if changed (T)"=FALSE, "refnum"=w814) -> ("error out"=w813:errorcluster)  [unwired: 7 in, 1 out]
        n457 = case shown="No Error" w813 {
          frame No Error {
            n458 = local read "Parameter Buffer"() -> (w833:T14)
            n459 = Unbundle By Name(w833) -> ("Start Holding Time and Date"=w831:string, "End Holding Time and Date"=w829:string, "Start Holding Temperature"=w828:string, "End Holding Temperature"=w827:string)
            n460 = Fract/Exp String To Number(string=w831) -> (number=w832:dbl)  [unwired: 3 in, 1 out]
            n461 = Fract/Exp String To Number(string=w829) -> (number=w830:dbl)  [unwired: 3 in, 1 out]
            n462 = Fract/Exp String To Number(string=w828) -> (number=w824:dbl)  [unwired: 3 in, 1 out]
            n463 = Fract/Exp String To Number(string=w827) -> (number=w823:dbl)  [unwired: 3 in, 1 out]
            n464 = To Time Stamp(1:w832) -> (0:w826:timestamp)
            n465 = To Time Stamp(1:w830) -> (0:w825:timestamp)
            n466 = local read "Info."() -> (w835:T8)
            n467 = call "Parameters - Update.vi"("Parameter (End Dwell Temp)"=w823, "Parameter (Start Dwell Temp)"=w824, "Parameter (End Dwell Time)"=w825, "Parameter (Start Dwell Time)"=w826, "Info."=w835) -> ("Parameters"=w834:string[][])  [unwired: 3 in, 3 out]
            n468 = call "Parameters UI - Dialog Box.vi"("Parameters"=w834) -> ()  [unwired: 10 in]
          }
          frame Error {
          }
        }
        n469 = Enqueue Element(queue=w820, element="[Key Parameters] Clicked By User." ("string"), timeout in ms (-1)=w821) -> ()  [unwired: 1 in, 3 out]
      }
      event "Read ET3500 Program": Value Change {
        n470 = event-data() -> ()  [unwired: 1 in, 6 out]
        n471 = local read "VISA resource name RS232"() -> (w839:string)
        n472 = local read "Simulate ET3500"() -> (w836:bool)
        n473 = call "ET3500 - Read Program.vi"("subVI"=TRUE, "Simulate"=w836, "VISA resource name"=w839) -> ("error out"=w837:errorcluster)  [unwired: 6 in, 2 out]
        n474 = local write "ET3500 Error"(w837) -> ()
      }
      event "------------------------------------             Report          ------------------------------------": Value Change {
        n475 = event-data() -> ()  [unwired: 1 in, 6 out]
      }
      event "Report Selection.Report Execute Search": Value Change {
        n476 = event-data() -> ()  [unwired: 1 in, 6 out]
        n477 = Unbundle By Name("Report Selection") -> ("Date Start"=w865:timestamp, "Date End"=w864:timestamp, "Selection Transaction No"=w861:string, "Selection Order No"=w862:string)
        n478 = call "String - Get Dates.vi"("End Date"=w864, "Start Date"=w865) -> ("List of Dates YYYYmmDD"=w860:string[])  [unwired: 8 in, 1 out]
        n479 = Empty String/Path?(string/path=w861) -> (empty?=w863:bool)
        n480 = case shown="False" w863 {
          tunnel: w862 -> [_ w902]
          tunnel: w861 -> [w899 _]
          tunnel: [w897 w900] -> w859
          frame False {
            # "Use Transaction No."
            n481 = property on="Selection Order No" class="Str"("Value"="") -> ()  [unwired: 2 in, 2 out]
            n482 = Concatenate Strings(w899, "_", ".*_" ("string")) -> (w897:string)
          }
          frame True {
            # "Selection Order No"
            n483 = Concatenate Strings(".*_" ("string"), w902, "_" ("string")) -> (w900:string)
          }
        }
        n484 = local read "Reports"() -> (w846:path)
        n485 = call "Folder - Subtract Number of Months.vi"("- # of Months"=0, "YYYYmm"="201301", "Folder"=w846) -> (">= Range (Folder\\YYYY\\mm)"=w844:path[])  [unwired: 6 in, 2 out]
        n486 = for {
          tunnel: [w868] -> w843 mode=concatenating
          tunnel: w844 -> [w867] mode=indexing
          n487 = List Folder(path=w867) -> (filenames=w868:string[])  [unwired: 3 in, 3 out]
        }
        n488 = for {
          tunnel: w860 -> [w892] mode=indexing
          tunnel: w859 -> [w894]
          tunnel: [w893] -> w858 mode=indexing
          n489 = Concatenate Strings(w894, w892) -> (w893:string)
        }
        n490 = for {
          tunnel: w858 -> [w881] mode=indexing
          tunnel: w843 -> [w880]
          shift-right: [w879] -> w856
          shift-left: string[] [] -> [w878]
          n491 = for {
            tunnel: w881 -> [w883]
            tunnel: w880 -> [w884] mode=indexing
            shift-right: [w886] -> w879
            shift-left: w878 -> [w885]
            n492 = Match Pattern(string=w884, regular expression=w883) -> (offset past match=w882:i32)  [unwired: 1 in, 3 out]
            n493 = Greater Or Equal To 0?(x=w882) -> (x >= 0?=w887:bool)
            n494 = case shown="True" w887 {
              tunnel: w884 -> [_ w889]
              tunnel: [w888 w891] -> w886
              tunnel: w885 -> [w888 w890]
              frame False {
              }
              frame True {
                n495 = Build Array (concatenate)(w890, w889) -> (w891:string[])
              }
            }
          }
        }
        "List Of Files From Selected Reports" <- w856
        n496 = for {
          tunnel: w856 -> [w877] mode=indexing
          tunnel: [w876] -> w855 mode=indexing
          tunnel: [w873] -> w854 mode=indexing
          tunnel: [w869] -> w851 mode=indexing
          w874 = "_" ("regular expression")
          n497 = Match Pattern(string=w877, regular expression=w874) -> (before substring=w876:string, after substring=w875:string)  [unwired: 1 in, 2 out]
          n498 = Match Pattern(string=w875, regular expression=w874) -> (before substring=w873:string, after substring=w872:string)  [unwired: 1 in, 2 out]
          n499 = Match Pattern(string=w872, regular expression="\\.") -> (before substring=w870:string)  [unwired: 1 in, 3 out]
          n500 = call "String - Convert String Only TimeStamp.vi"("YYYYmmdd_HHMMSS"=w870) -> ("YYYY-mm-dd HH:MM:SS"=w869:string)  [unwired: 10 in]
        }
        n501 = Enqueue Element(queue=w848, element="[Report Search Execute]. " ("string"), timeout in ms (-1)=w849) -> ()  [unwired: 1 in, 3 out]
        n502 = Build Array(w851, w855, w854) -> (w853:string[][])
        n503 = Transpose 2D Array(2D array=w853) -> (transposed array=w852:string[][])
        n504 = property on="Report List" class="MCListbox (strict)"("ItemNames"=w852) -> (error out=w840:errorcluster)  [unwired: 2 in, 1 out]
        n505 = property on="Report List" class="MCListbox (strict)"(error in=w840, "TopLeft"=T22 {"Row"=0, "Column"=0} ("Top Left Visible Cell"), "Value"=-1 ("Report List")) -> ()  [unwired: 1 in, 2 out]
      }
      event "Report Open": Value Change {
        w921 = "\"" ("string")
        n506 = event-data() -> ()  [unwired: 1 in, 6 out]
        n507 = local read "List Of Files From Selected Reports"() -> (w932:string[])
        n508 = local read "Report List"() -> (w931:i32)
        n509 = Index Array(array=w932, index=w931) -> (element=w925:string)
        n510 = Match Pattern(string=w925, regular expression="_") -> (after substring=w929:string)  [unwired: 1 in, 3 out]
        n511 = Match Pattern(string=w929, regular expression="_") -> (after substring=w910:string)  [unwired: 1 in, 3 out]
        n512 = local read "Reports"() -> (w911:path)
        n513 = String Subset(string=w910, length (rest)=4 ("length (rest)")) -> (substring=w906:string)  [unwired: 1 in]
        n514 = String Subset(string=w910, offset (0)=4, length (rest)=2 ("length (rest)")) -> (substring=w907:string)
        n515 = Concatenate Strings(w906, "\\" ("string"), w907) -> (w904:string)
        n516 = Build Path(base path=w911, name or relative path=w904) -> (appended path=w930:path)
        n517 = Build Path(base path=w930, name or relative path=w925) -> (appended path=w924:path)
        n518 = Path To String(path=w924) -> (string=w918:string)
        n519 = Concatenate Strings(w921, w918, w921) -> (w913:string)
        n520 = Concatenate Strings("[OPEN REPORT] Clicked By User. " ("string"), w913, " is selected." ("string")) -> (w914:string)
        n521 = Enqueue Element(queue=w919, element=w914, timeout in ms (-1)=w920) -> ()  [unwired: 1 in, 3 out]
        n522 = Concatenate Strings("cmd  /c  start acrord32.exe " ("string"), w913) -> (w916:string)
        n523 = call <vilib>:"System Exec.vi"("run minimized? (F)"=TRUE, "wait until completion? (T)"=FALSE, "command line"=w916) -> ()  [unwired: 5 in, 4 out]
      }
      event "Report Generate": Value Change {
        # "Create Report File from Raw Data File and Setup File"
        n524 = event-data() -> ()  [unwired: 1 in, 1 out]
        n525 = local read "Raw Data File"() -> (w939:path)
        n526 = Format Date/Time String "Date_Time"(time format string (%c)="%Y%m%d_%H%M%S") -> (date/time string=w973:string)  [unwired: 2 in]
        n527 = Array Subset "The Other 3 MCListbox"(array=w993, index=1) -> (w980:refnum<vi>[])  [unwired: 1 in]
        n528 = Build Array (concatenate)(w980, w979) -> (w978:refnum<vi>[])
        n529 = Index Array(array=w993, index=0) -> (element=w977:refnum<vi>)
        n530 = Strip Path(path=w939) -> (name=w1001:string)  [unwired: 1 out]
        n531 = Match Pattern(string=w1001, regular expression="_") -> (before substring=w948:string, after substring=w1000:string)  [unwired: 1 in, 2 out]
        n532 = local read "Setup"() -> (w956:path)
        n533 = Concatenate Strings(w948, "_*.stp" ("string")) -> (w996:string)
        n534 = Match Pattern(string=w1000, regular expression="_") -> (before substring=w961:string)  [unwired: 1 in, 3 out]
        n535 = String Subset(string=w961, length (rest)=4 ("length (rest)")) -> (substring=w958:string)  [unwired: 1 in]
        n536 = String Subset(string=w961, offset (0)=4, length (rest)=2 ("length (rest)")) -> (substring=w957:string)
        n537 = Concatenate Strings(w958, w957) -> (w954:string)
        "YYYYmm" <- w954
        n538 = call "Folder - Subtract Number of Months.vi"("- # of Months"=3, "YYYYmm"=w954, "Folder"=w956) -> (">= Range (Folder\\YYYY\\mm)"=w953:path[])  [unwired: 6 in, 2 out]
        n539 = for {
          tunnel: w996 -> [w1033]
          tunnel: w953 -> [w1032] mode=indexing
          tunnel: [w1031] -> w952
          tunnel: [w1028] -> w951
          stop <- w1029 stop-if-true
          n540 = List Folder(path=w1032, pattern=w1033) -> (path out=w1031:path, filenames=w1030:string[])  [unwired: 2 in, 2 out]
          n541 = for {
            tunnel: w1030 -> [w1036] mode=indexing
            tunnel: [w1034] -> w1029
            tunnel: [w1036] -> w1028
            stop <- w1034 stop-if-true
            n542 = Empty String/Path?(string/path=w1036) -> (empty?=w1035:bool)
            n543 = Not(x=w1035) -> (.not. x?=w1034:bool)
          }
        }
        n544 = Build Path(base path=w952, name or relative path=w951) -> (appended path=w950:path)
        n545 = Not A Number/Path/Refnum?(number/path/refnum=w950) -> (NaN/Path/Refnum?=w949:bool)
        n546 = case shown="False" w949 {
          tunnel: w948 -> [_ w1027]
          tunnel: [_ errorcluster {"status"=TRUE, "code"=-8001, "source"=" setup file (.stp) not found."} ("error in (no error)")] -> w937
          frame False {
          }
          frame True {
            n547 = Concatenate Strings("Transaction Number " ("string"), w1027, " setup file (.stp) not found." ("string")) -> (w1024:string)
            n548 = One Button Dialog(message=w1024) -> ()  [unwired: 1 in, 1 out]
          }
        }
        n549 = call <vilib>:"Open Config Data.vi"("error in (no error)"=w937, "create file if necessary (T)"=FALSE, "configuration file path"=w950) -> ("error out"=w933:errorcluster, "refnum"=w934:T33)  [unwired: 6 in, 1 out]
        n550 = for {
          tunnel: w978 -> [w1122] mode=indexing
          tunnel: w934 -> [w1123]
          tunnel: w933 -> [w1126]
          shift-right: [w1124] -> w983
          shift-left: "" -> [w1125]
          tunnel: [w1121] -> w971 mode=indexing
          n551 = call "Key - Read to Spreadsheet String.vi"("error in (no error)"=w1126, "String in"=w1125, "Control in"=w1122, "ini File Ref num"=w1123) -> ("error out"=w1121:errorcluster, "String out"=w1124:string)  [unwired: 6 in]
        }
        n552 = call "Key - Read to Spreadsheet String.vi"("error in (no error)"=w933, "Control in"=w977, "ini File Ref num"=w934) -> ("error out"=w972:errorcluster, "String out"=w986:string)  [unwired: 7 in]
        n553 = Spreadsheet String To Array(delimiter (Tab)=",", format string="", spreadsheet string=w986, array type (2D Dbl)=string[][] []) -> (array=w984:string[][])
        n554 = Merge Errors(w972, w971) -> (w970:errorcluster)
        n555 = Array Size(array=w984) -> (size(s)=w991:i32[])
        n556 = Index Array(array=w991, index=1) -> (element=w989:i32)
        n557 = Decrement(x=w989) -> (x-1=w988:i32)
        n558 = case shown="No Error" w933 {
          tunnel: [w1014 _] -> w962
          tunnel: w934 -> [w1003 _]
          frame No Error {
            n559 = flat-sequence {
              tunnel: w1003 -> [w1019]
              tunnel: [w1021] -> w1002
              frame #0 {
                n560 = control-ref of="Parameter Buffer"() -> (w1020:refnum<vi>)
                n561 = call "Key - Cluster Read.vi"("New Ctl Ref"=w1020, "Original Ctl Ref"=w1020, "Refnum in"=w1019) -> ()  [unwired: 6 in, 3 out]
              }
              frame #1 {
                n562 = local read "Parameter Buffer"() -> (w1021:T14)
              }
            }
            n563 = Unbundle By Name(w1002) -> ("Start Holding Time and Date"=w1012:string, "End Holding Time and Date"=w1010:string, "Start Holding Temperature"=w1009:string, "End Holding Temperature"=w1008:string)
            n564 = Fract/Exp String To Number(string=w1012) -> (number=w1013:dbl)  [unwired: 3 in, 1 out]
            n565 = Fract/Exp String To Number(string=w1010) -> (number=w1011:dbl)  [unwired: 3 in, 1 out]
            n566 = Fract/Exp String To Number(string=w1009) -> (number=w1005:dbl)  [unwired: 3 in, 1 out]
            n567 = Fract/Exp String To Number(string=w1008) -> (number=w1004:dbl)  [unwired: 3 in, 1 out]
            n568 = local read "Info."() -> (w1018:T8)
            n569 = To Time Stamp(1:w1013) -> (0:w1007:timestamp)
            n570 = To Time Stamp(1:w1011) -> (0:w1006:timestamp)
            n571 = call "Parameters - Update.vi"("Parameter (End Dwell Temp)"=w1004, "Parameter (Start Dwell Temp)"=w1005, "Parameter (End Dwell Time)"=w1006, "Parameter (Start Dwell Time)"=w1007, "Info."=w1018) -> ("Parameters"=w1017:string[][])  [unwired: 3 in, 3 out]
            n572 = Array To Spreadsheet String(delimiter (Tab)=",", array=w1017, 3:"" ("format string")) -> (spreadsheet string=w1014:string)
          }
          frame Error {
          }
        }
        n573 = for {
          N: w988 -> [_]
          tunnel: w984 -> [w1138]
          tunnel: w983 -> [w1134]
          tunnel: [w1133] -> w974 mode=indexing
          tunnel: [w1128] -> w965 mode=indexing
          tunnel: w962 -> [w1127]
          i -> [w1142]
          # "List by Order Number"
          n574 = Increment(x=w1142) -> (x+1=w1141:i32)
          n575 = Index Array(array=w1138, index (col) #1=0 ("disabled index (col)"), index (col) #2=w1141) -> (element #1=w1139:string[], element #2=w1130:string[])  [unwired: 2 in]
          n576 = Build Array(w1139, w1130) -> (w1132:string[][])
          n577 = Index Array(array=w1130, index=1) -> (element=w1128:string)
          n578 = Transpose 2D Array(2D array=w1132) -> (transposed array=w1131:string[][])
          n579 = Array To Spreadsheet String(delimiter (Tab)=",", array=w1131, 3:"" ("format string")) -> (spreadsheet string=w1135:string)
          n580 = Concatenate Strings(w1135, w1134, w1127) -> (w1133:string)
        }
        "Details From .stp and Parameters" <- w974
        "Order No" <- w965
        n581 = for {
          tunnel: w974 -> [w1067] mode=indexing
          tunnel: w965 -> [w1072] mode=indexing
          tunnel: w948 -> [w1073]
          tunnel: w973 -> [w1070]
          shift-right: [w1063] -> w969
          shift-left: w970 -> [w1053]
          tunnel: [w1059] -> w936 mode=indexing
          shift-right: [w1049] -> w938
          shift-left: _ -> [w1048]
          i -> [w1050]
          w1062 = "\"" ("string")
          w1071 = "_" ("string")
          # "List by Order Number"
          n582 = case shown="0" w1050 {
            tunnel: [w1074 w1075] -> w1049
            tunnel: w1048 -> [w1074 _]
            frame 1, Default {
            }
            frame 0 {
              n583 = local read "Parameter (End Dwell Time)"() -> (w1078:timestamp)
              n584 = Equal?(x=w1078, y=timestamp(3471350400 s since 1904-01-01) ("Parameter (Start Dwell Time)")) -> (x = y?=w1076:bool)
              n585 = case shown="True" w1076 {
                tunnel: [TRUE ("T button?") w1081] -> w1075
                frame False {
                }
                frame True {
                  # "Prompts on 1st Order No only"
                  n586 = Two Button Dialog(message="\"Hold\" did not complete. Do you still want to generate the Excel (and PDF) file?", 1:"No" ("F button name (\"Cancel\")"), 2:"Yes" ("T button name (\"OK\")")) -> (T button?=w1081:bool)
                }
              }
              n587 = case shown="True" w1075 {
                frame False {
                }
                frame True {
                  n588 = call "Msgbox - Add OR Remove.vi"("MsgBox"=T30 {"Show"=TRUE, "Priority"=0, "Message"="Generating Report..."}) -> ()  [unwired: 9 in, 2 out]
                }
              }
            }
          }
          n589 = local read "Reports"() -> (w1052:path)
          n590 = local read "Excel"() -> (w1057:path)
          n591 = Concatenate Strings(w1073, w1071, w1072, w1071, w1070, ".xls" ("string")) -> (w1061:string)
          n592 = call "Folder - Create Year-Month.vi"("error in (no error)"=w1053, "Folder Name"=w1052) -> ("error out"=w1054:errorcluster)  [unwired: 8 in, 1 out]
          n593 = call "Folder - Create Year-Month.vi"("error in (no error)"=w1053, "Folder Name"=w1057) -> ("error out"=w1055:errorcluster, "Folder with Year\\Month"=w1056:path)  [unwired: 8 in]
          n594 = Merge Errors(w1055, w1054) -> (w1058:errorcluster)
          n595 = local read "Raw Data File"() -> (w1068:path)
          n596 = Build Path(base path=w1056, name or relative path=w1061) -> (appended path=w1066:path)
          n597 = local read "MasterData\\JPG"() -> (w1064:path)
          n598 = case shown="True" w1049 {
            tunnel: w1068 -> [_ w1094]
            tunnel: w1067 -> [_ w1093]
            tunnel: w1066 -> [_ w1092]
            tunnel: "Report.Create.PDF" -> [_ w1091]
            tunnel: w1064 -> [_ w1090]
            tunnel: [w1085 w1089] -> w1063
            tunnel: w1058 -> [w1085 w1088]
            tunnel: w1057 -> [_ w1087]
            tunnel: w1052 -> [_ w1086]
            frame False {
            }
            frame True {
              n599 = while {
                tunnel: w1094 -> [w1106]
                tunnel: w1093 -> [w1105]
                tunnel: [w1096] -> w1089
                tunnel: w1088 -> [w1104]
                tunnel: w1087 -> [w1103]
                tunnel: w1092 -> [w1102]
                tunnel: w1091 -> [w1101]
                tunnel: w1090 -> [w1100]
                tunnel: w1086 -> [w1095]
                i -> [w1097]
                stop <- w1098 stop-if-true
                n600 = call "Report - Excel.vi"("pdf"=w1101, "Chart Seperation by Order#"=w1095, "Details from .stp and Parameters"=w1105, "Use DB for Picture (Material)"=w1100, "error in (no error)"=w1104, "Include MetaData"=w1106, "Report Additional Details"=w1102, "Report Files Cluster"=w1103) -> ("error out"=w1099:errorcluster)  [unwired: 1 in, 2 out]
                n601 = case shown="Error" w1099 {
                  selector: w1099 -> [w1107 w1109]
                  tunnel: [TRUE w1110] -> w1098
                  tunnel: w1097 -> [_ w1112]
                  tunnel: [w1107 w1111] -> w1096
                  frame No Error {
                  }
                  frame Error {
                    n602 = Greater Or Equal?(x=w1112, y=2) -> (x >= y?=w1110:bool)
                    n603 = case shown="True" w1110 {
                      tunnel: [errorcluster {"status"=FALSE, "code"=0, "source"=""} ("error out") w1115] -> w1111
                      tunnel: w1109 -> [_ w1115]
                      frame False {
                      }
                      frame True {
                      }
                    }
                  }
                }
              }
            }
          }
          n604 = Concatenate Strings(w1062, w1061, w1062) -> (w1060:string)
          n605 = case shown="Error" w1063 {
            tunnel: [w1116 " create ERROR." ("string")] -> w1051
            tunnel: w1049 -> [w1119 _]
            frame No Error {
              n606 = Select(t=" created OK. " ("string"), s=w1119, f=" skipped. ") -> (s? t:f=w1116:string)
            }
            frame Error {
            }
          }
          n607 = Concatenate Strings(w1060, w1051) -> (w1059:string)
        }
        n608 = case shown="True" w938 {
          frame False {
          }
          frame True {
            n609 = call "Msgbox - Add OR Remove.vi"("MsgBox"=T30 {"Show"=FALSE, "Priority"=0, "Message"=""}) -> ()  [unwired: 9 in, 2 out]
          }
        }
        n610 = case shown="Error" w969 {
          selector: w969 -> [_ w1041]
          tunnel: [_ FALSE] -> w968
          tunnel: w936 -> [w1037 w1039]
          tunnel: [w1037 w1038] -> w935
          frame No Error {
          }
          frame Error {
            n611 = Unbundle By Name(w1041) -> ("code"=w1040:i32)
            n612 = case shown="0, Default" w1040 {
              tunnel: w1041 -> [w1044 _]
              tunnel: w1039 -> [w1043 _]
              tunnel: [w1043 w1046] -> w1038
              frame 0, Default {
                n613 = call <vilib>:"Simple Error Handler.vi"("error source (\" \")"="Create xls file" ("error source (\" \")"), "error in (no error)"=w1044) -> ()  [unwired: 3 in, 5 out]
              }
              frame -8001 {
                n614 = Build Array("Failed") -> (w1046:string[])
              }
            }
          }
        }
        n615 = Array To Spreadsheet String(delimiter (Tab)="\n", array=w935, 3:"" ("format string")) -> (spreadsheet string=w941:string)
        n616 = Concatenate Strings("[Generate Report]. \n" ("string"), w941) -> (w943:string)
        n617 = Search and Replace String(replace all?=TRUE ("replace all? (F)"), case sensitive?=TRUE ("ignore case? (F)"), input string=w943, search string="xls", replace string="pdf" ("replace string (\"\")")) -> (result string=w942:string)  [unwired: 3 in, 3 out]
        n618 = One Button Dialog(message=w942) -> ()  [unwired: 1 in, 1 out]
        n619 = Enqueue Element(queue=w966, element=w943, timeout in ms (-1)=w967) -> ()  [unwired: 1 in, 3 out]
        n620 = local write "Report Generate"(w968) -> ()
      }
      event "------------------------------------        MCListBox       ------------------------------------": Value Change {
        n621 = event-data() -> ()  [unwired: 1 in, 6 out]
      }
      event "MCListBox FHS Setup Add Button", "MCListBox FHS Setup Remove Button", "MCListBox AWPS Add Button", "MCListBox AWPS Remove Button", "MCListBox FHS Master Data Add Button", "MCListBox FHS Master Data Remove Button": Value Change {
        n622 = event-data() -> ("CtlRef"=w1153:refnum<vi>)  [unwired: 1 in, 5 out]
        n623 = local read "CellBG Unused Cells"() -> (w1144:u32)
        n624 = local read "CellBG New Cells"() -> (w1145:u32)
        n625 = Or(x="MCListBox FHS Master Data Add Button", y="MCListBox FHS Master Data Remove Button") -> (x .or. y?=w1146:bool)
        n626 = Select(t=w1145, s=w1146, f=w1144) -> (s? t:f=w1143:u32)
        n627 = case shown="True" "MCListBox AWPS Add Button" {
          tunnel: [T5[] [] w1165] -> w1152
          tunnel: [_ w1163] -> w1150
          frame False {
          }
          frame True {
            w1155 = ""
            # "To Add via ComboBox"
            n628 = control-ref of="Additional Rev"() -> (w1166:refnum<vi>)
            n629 = control-ref of="Additional WPS/Ref"() -> (w1167:refnum<vi>)
            n630 = property class="CmbBox (strict)"(reference=w1167) -> (reference out=w1157:refnum<vi>, "Value"=w1164:T5)  [unwired: 1 in, 1 out]
            n631 = property class="CmbBox (strict)"(reference=w1166) -> (reference out=w1156:refnum<vi>, "Value"=w1159:T5)  [unwired: 1 in, 1 out]
            n632 = Empty String/Path?(string/path=w1164) -> (empty?=w1162:bool)
            n633 = Empty String/Path?(string/path=w1159) -> (empty?=w1161:bool)
            n634 = call <vilib>:"Space Constant.vi"() -> ("String"=w1160:string)
            n635 = Select(t=w1160, s=w1161, f=w1159) -> (s? t:f=w1158:T5)
            n636 = Build Array(w1164, w1158) -> (w1165:T5[])
            n637 = case shown="True" w1162 {
              tunnel: [_ errorcluster {"status"=TRUE, "code"=0, "source"=""} ("error constant")] -> w1163
              frame False {
              }
              frame True {
                n638 = One Button Dialog(message="Empty Field. Additional WPS/Ref and Rev are not Added.") -> ()  [unwired: 1 in, 1 out]
              }
            }
            n639 = property class="CmbBox (strict)"(reference=w1157, "Value"=w1155) -> ()  [unwired: 1 in, 2 out]
            n640 = property class="CmbBox (strict)"(reference=w1156, "Value"=w1155) -> ()  [unwired: 1 in, 2 out]
          }
        }
        n641 = call "MCListbox Event - Add and Remove Buttons.vi"("CellBG New Cells"=w1143, "CellBG Unused Cells"=w1144, "new element/subarray"=w1152, "Error In"=w1150, "MCListBox Ref"=w1151, "CtlRef Boolean"=w1153) -> ()  [unwired: 5 in, 1 out]
      }
      event "MCListBox FHS Setup", "MCListBox FHS Master Data": Key Down? {
        # "Only the 2 FHS (Furnace Heating Sequence) have direct Keyboard Entries"
        n642 = event-data() -> ("CtlRef"=w1175:refnum<vi>, "Char"=w1170:i16, "VKey"=w1172:T31)  [unwired: 1 in, 7 out]
        n643 = call "MCListbox Event - Key Down QuestionMark.vi"("Key Down?"=w1174, "CtlRef"=w1175) -> ()  [unwired: 9 in, 1 out]
        n644 = case "Only NUMBERS, BackSpace and (Return, Enter, Up, Down, Right, Left, Delete)" shown="0, Default" w1170 {
          tunnel: [w1177 w1180] -> w1171
          tunnel: w1172 -> [w1176 _]
          frame 0, Default {
            # "Exception"
            n645 = case shown="\"Enter\", \"Return\", \"Up\"..\"Right\", \"Delete\"" w1176 {
              tunnel: [w1178 w1179] -> w1177
              frame Default {
                w1178 = TRUE  # Discard
              }
              frame "Enter", "Return", "Up".."Right", "Delete" {
                w1179 = FALSE  # Do Not Discard
                # "Up, Down, Left, Right, Delete"
              }
            }
          }
          frame 8, 48..57 {
            w1180 = FALSE  # Do not discard
            # "Backspace, decimal point, Numbers, colon"
          }
        }
        n646 = event-data("Discard?"=w1171) -> ()  [unwired: 1 in, 1 out]
      }
      event "MCListBox FHS Setup", "MCListBox FHS Master Data": Key Down {
        # "Only the 2 FHS (Furnace Heating Sequence) have direct Keyboard Entries"
        n647 = event-data() -> ("CtlRef"=w1183:refnum<vi>, "Char"=w1182:i16, "VKey"=w1181:T31)  [unwired: 1 in, 7 out]
        n648 = call "MCListbox Event - Key Down.vi"("VKey"=w1181, "Char"=w1182, "CtlRef"=w1183) -> ()  [unwired: 7 in, 2 out]
      }
      event "MCListBox AWPS", "MCListBox FHS Setup", "MCListBox FHS Master Data": Mouse Down {
        # "Only the 2 FHS (Furnace Heating Sequence) AND AWPS  have selection of Row Cells Keyboard"
        n649 = event-data() -> ("CtlRef"=w1184:refnum<vi>)  [unwired: 1 in, 7 out]
        n650 = call "MCListbox Event - Mouse Down.vi"("CtlRef"=w1184) -> ()  [unwired: 10 in, 1 out]
      }
      event "------------------------------------        Part Details       ------------------------------------": Value Change {
        n651 = event-data() -> ()  [unwired: 1 in, 6 out]
      }
      event "Part Details Add": Value Change {
        w1201 = string[] ["TC1", "TC2", "TC3", "TC4", "TC5", "TC6"]  # Channel to Probe Cluster Label
        w1193 = string[] ["Order No.", "Oper. No.", "Customer Name", "Project", "Material", "Material Description", "User"]  # Mandatory Fields
        n652 = event-data() -> ()  [unwired: 1 in, 6 out]
        n653 = control-ref of="Channel Mapping"() -> (w1222:refnum<vi>)
        n654 = control-ref of="Item Details"() -> (w1225:refnum<vi>)
        n655 = property on="Part Details" class="MCListbox (strict)"() -> ("ColHdrString"=w1202:string[], "ItemNames"=w1209:string[][])  [unwired: 2 in, 2 out]
        n656 = Array Size(array=w1202) -> (size(s)=w1219:i32)
        n657 = property class="Clust (strict)"(reference=w1222) -> ("Controls[]"=w1221:refnum<vi>[])  [unwired: 1 in, 2 out]
        n658 = property class="Clust (strict)"(reference=w1225) -> ("Controls[]"=w1206:refnum<vi>[])  [unwired: 1 in, 2 out]
        n659 = Initialize Array("", w1219) -> (w1217:string[])
        n660 = flat-sequence {
          frame #0 {
            n661 = Wait (ms)(milliseconds to wait=u32 100) -> ()  [unwired: 1 out]
          }
          frame #1 {
            n662 = local write "Part Details Add"(FALSE ("Part Details Add")) -> ()
          }
        }
        n663 = control-ref of="Channel to Probe Mapping"() -> (w1204:refnum<vi>)
        n664 = control-ref of="No."() -> (w1207:refnum<vi>)
        n665 = control-ref of="User"() -> (w1216:refnum<vi>)
        n666 = control-ref of="Notes"() -> (w1205:refnum<vi>)
        n667 = Index Array(array=w1209, index (col)=0 ("disabled index (col)")) -> (element=w1214:string[])  [unwired: 1 in]
        n668 = Number To Decimal String(number="No.") -> (decimal integer string=w1212:string)  [unwired: 1 in]
        n669 = Build Array (concatenate)(w1216, w1207, w1206, w1205, w1221, w1204) -> (w1223:refnum<vi>[])
        n670 = Search 1D Array(1D array=w1214, element=w1212) -> (index of element=w1203:i32)  [unwired: 1 in]
        n671 = case shown="-1" w1203 {
          selector: w1203 -> [w1278 _]
          tunnel: [w1278 w1283] -> w1224
          tunnel: [w1279 w1282] -> w1220
          tunnel: w1217 -> [_ w1281]
          tunnel: w1209 -> [w1279 w1280]
          frame 0, Default {
            # "Found"
          }
          frame -1 {
            # "Not Found, Add new row"
            n672 = Build Array (concatenate)(w1280, w1281) -> (w1282:string[][])
            n673 = Array Size(array=w1282) -> (size(s)=w1285:i32[])
            n674 = Index Array(array=w1285) -> (element=w1284:i32)  [unwired: 1 in]
            n675 = Decrement(x=w1284) -> (x-1=w1283:i32)
          }
        }
        n676 = Array Size(array=w1193) -> (size(s)=w1192:i32)
        n677 = Decrement(x=w1192) -> (x-1=w1191:i32)
        n678 = for {
          tunnel: w1223 -> [w1295] mode=indexing
          tunnel: w1202 -> [w1293]
          shift-right: [w1288] -> w1194
          shift-left: w1220 -> [w1290]
          tunnel: w1224 -> [w1289]
          # "Updates to MCListBox"
          n679 = property class="Ctl"(reference=w1295) -> ("ClassName"=w1292:string, "Label.Text"=w1287:string, "Value"=w1294:variant)  [unwired: 1 in, 2 out]
          n680 = Search 1D Array(1D array=w1293, element=w1287) -> (index of element=w1291:i32)  [unwired: 1 in]
          n681 = case shown="0, Default" w1291 {
            selector: w1291 -> [w1299 _]
            tunnel: w1294 -> [w1302 _]
            tunnel: w1292 -> [w1301 _]
            tunnel: w1290 -> [w1300 w1314]
            tunnel: w1289 -> [w1298 _]
            tunnel: [w1296 w1314] -> w1288
            frame 0, Default {
              n682 = case shown="\"Boolean\"" w1301 {
                tunnel: w1302 -> [w1306 w1309 w1313]
                tunnel: [w1303 w1307 w1310] -> w1297
                frame "Digital" {
                  n683 = Variant To Data(type=0, Variant=w1306) -> (data=w1304:i32)  [unwired: 1 in, 1 out]
                  n684 = Format Into String(w1304) -> (resulting string=w1303:string)  [unwired: 3 in, 1 out]
                }
                frame "ComboBox", "String", Default {
                  n685 = Variant To Data(type="", Variant=w1309) -> (data=w1307:string)  [unwired: 1 in, 1 out]
                }
                frame "Boolean" {
                  n686 = Variant To Data(type=TRUE, Variant=w1313) -> (data=w1311:bool)  [unwired: 1 in, 1 out]
                  n687 = Format Into String(w1311) -> (resulting string=w1310:string)  [unwired: 3 in, 1 out]
                }
              }
              n688 = Replace Array Subset(array=w1300, new element=w1297, index (row)=w1298, index (col)=w1299) -> (w1296:string[][])
            }
            frame -1 {
            }
          }
        }
        n689 = while {
          tunnel: w1202 -> [w1236]
          tunnel: w1193 -> [w1228] mode=indexing
          tunnel: w1194 -> [w1237]
          tunnel: [w1235] -> _
          tunnel: [w1234] -> _
          tunnel: w1191 -> [w1233]
          tunnel: [w1229] -> w1190
          tunnel: [w1228] -> w1189
          i -> [w1232]
          stop <- w1231 stop-if-true
          # "Check Mandatory Fields"
          n690 = Search 1D Array(1D array=w1236, element=w1228) -> (index of element=w1238:i32)  [unwired: 1 in]
          n691 = Equal?(x=w1233, y=w1232) -> (x = y?=w1230:bool)
          n692 = case shown="0, Default" w1238 {
            selector: w1238 -> [w1239 _]
            tunnel: w1237 -> [w1244 _]
            tunnel: [w1241 FALSE] -> w1229
            tunnel: [w1240 -1 ("index of element")] -> w1235
            tunnel: [w1239 -1 ("index of element")] -> w1234
            frame 0, Default {
              # "Mandatory Field"
              n693 = Index Array(array=w1244, index (col)=w1239) -> (element=w1243:string[])  [unwired: 1 in]
              n694 = Search 1D Array(1D array=w1243, element="") -> (index of element=w1240:i32)  [unwired: 1 in]
              n695 = Greater Or Equal To 0?(x=w1240) -> (x >= 0?=w1241:bool)
            }
            frame -1 {
            }
          }
          n696 = Or(x=w1229, y=w1230) -> (x .or. y?=w1231:bool)
        }
        "Empty String in Mandatory Field" <- w1190
        n697 = Array Size(array=w1209) -> (size(s)=w1210:i32[])
        n698 = Add Array Elements(numeric array=w1210) -> (sum=w1211:i32)
        n699 = Equal To 0?(x=w1211) -> ()  [unwired: 1 out]
        n700 = local read "Channel to Probe Mapping"() -> (w1199:cluster{"Channel to Probe Mapping":string})
        n701 = Unbundle By Name(w1199) -> ("Channel to Probe Mapping"=w1198:string)
        n702 = call "String - Channel to Probe Mappings.vi"("Channel to Probe Mapping"=w1198, "Channel to Probe Cluster Label"=w1201, "ColHdrString"=w1202, "ItemNames"=w1194) -> ("Probe List Valid"=w1188:bool, "Probe List"=→"Probe List":i32[], "Available Probe List"=w1195:string, "cRIO Channel List"=→"cRIO Channel List":i32[], "Duplicate"=w1187:bool, "Duplicated Probe #"=w1186:i32)  [unwired: 1 in, 1 out]
        "Probe List Valid" <- w1188
        n703 = Not(x=w1188) -> (.not. x?=w1197:bool)
        n704 = Or(x=w1190, y=w1197) -> (x .or. y?=w1208:bool)
        n705 = case shown="False" w1208 {
          tunnel: w1194 -> [w1286 _]
          frame False {
            n706 = property on="Part Details" class="MCListbox (strict)"("ItemNames"=w1286) -> ()  [unwired: 2 in, 2 out]
          }
          frame True {
          }
        }
        n707 = case shown="True" w1190 {
          tunnel: w1189 -> [_ w1273]
          tunnel: [_ w1270] -> w1185
          frame False {
            # "No Empty Field"
          }
          frame True {
            # "Empty Field"
            n708 = property on="Part Details Add" class="Bool (strict)"() -> ("BoolText.Text"=w1276:string)  [unwired: 2 in, 2 out]
            n709 = Concatenate Strings("[" ("string"), w1273, "]" ("string"), " cannot be empty.\n" ("message"), "Part Details Not " ("string"), w1276, "ed." ("string")) -> (w1270:string)
          }
        }
        n710 = case shown="False" w1188 {
          tunnel: w1195 -> [w1253 _]
          tunnel: w1187 -> [w1255 _]
          tunnel: w1186 -> [w1254 _]
          tunnel: w1185 -> [w1248 w1267]
          frame False {
            # "Probe List NOT valid"
            n711 = case shown="True" w1255 {
              tunnel: w1254 -> [_ w1265]
              tunnel: w1253 -> [w1261 _]
              tunnel: [w1260 w1263] -> w1252
              frame False {
                n712 = Concatenate Strings("Available Probe List " ("message"), w1261) -> (w1260:string)
              }
              frame True {
                n713 = Format Into String(format string="%d is duplicated. ", initial string="Probe Number ", w1265) -> (resulting string=w1263:string)  [unwired: 1 in, 1 out]
              }
            }
            n714 = property on="Part Details Add" class="Bool (strict)"() -> ("BoolText.Text"=w1259:string)  [unwired: 2 in, 2 out]
            n715 = Empty String/Path?(string/path=w1248) -> (empty?=w1251:bool)
            n716 = Select(t=w1248, s=w1251, f="\n\n") -> (s? t:f=w1249:string)
            n717 = Concatenate Strings(w1248, w1249, w1252, "Part Details Not " ("message"), w1259, "ed." ("string")) -> (w1256:string)
            n718 = One Button Dialog(message=w1256) -> ()  [unwired: 1 in, 1 out]
          }
          frame True {
            # "Probe List Valid"
            n719 = Empty String/Path?(string/path=w1267) -> (empty?=w1268:bool)
            n720 = case shown="False" w1268 {
              tunnel: w1267 -> [w1269 _]
              frame False {
                n721 = One Button Dialog(message=w1269) -> ()  [unwired: 1 in, 1 out]
              }
              frame True {
              }
            }
          }
        }
      }
      event "Part Details Delete", "Setup New": Value Change {
        n722 = event-data() -> ("CtlRef"=w1326:refnum<vi>)  [unwired: 1 in, 5 out]
        n723 = property class="Bool"(reference=w1326) -> ("Label.Text"=w1325:string)  [unwired: 1 in, 2 out]
        n724 = local read "No."() -> (w1318:i32)
        n725 = Format Into String(format string="%d?", initial string="Delete Item ", w1318) -> (resulting string=w1315:string)  [unwired: 1 in, 1 out]
        n726 = Select(t="New Setup?", s="Setup New", f=w1315) -> (s? t:f=w1321:string)
        n727 = Concatenate Strings("Confirm " ("message"), w1321) -> (w1320:string)
        n728 = Two Button Dialog(message=w1320) -> (T button?=w1319:bool)  [unwired: 2 in]
        n729 = case shown="True" w1319 {
          tunnel: w1325 -> [_ w1328]
          tunnel: "Setup New" -> [_ w1327]
          frame False {
          }
          frame True {
            n730 = case shown="\"Setup New\", Default" w1328 {
              tunnel: [_ w1350] -> w1329
              frame "Setup New", Default {
                w1338 = 2 ("dimension size")
                w1339 = 3 ("dimension size")
                n731 = control-ref of="MCListBox AWPS"() -> (w1336:refnum<vi>)
                n732 = control-ref of="Additional WPS/Ref"() -> (w1332:refnum<vi>)
                n733 = control-ref of="WPS Details Setup"() -> (w1333:refnum<vi>)
                n734 = control-ref of="MCListBox FHS Setup"() -> (w1337:refnum<vi>)
                n735 = control-ref of="Part Details"() -> (w1347:refnum<vi>)
                n736 = Initialize Array("", w1339) -> (w1344:string[])
                n737 = Initialize Array("", w1338) -> (w1342:string[])
                n738 = invoke class="Clust (strict)" method="Reinit To Default"(reference=w1333) -> ()  [unwired: 2 in, 3 out]
                n739 = invoke class="Clust (strict)" method="Reinit To Default"(reference=w1332) -> ()  [unwired: 2 in, 3 out]
                n740 = Build Array(w1344) -> (w1343:string[][])
                n741 = Build Array(w1342) -> (w1341:string[][])
                n742 = property class="MCListbox (strict)"(reference=w1347, "ItemNames"=string[][] [] ("Item Names")) -> ()  [unwired: 1 in, 2 out]
                n743 = property on="Property Node" class="MCListbox (strict)"(reference=w1336, "ItemNames"=w1341, "NumCols"=w1338) -> (reference out=w1334:refnum<vi>)  [unwired: 1 in, 1 out]
                n744 = property on="Property Node" class="MCListbox (strict)"(reference=w1337, "ItemNames"=w1343, "NumCols"=w1339) -> (reference out=w1335:refnum<vi>)  [unwired: 1 in, 1 out]
                n745 = disable-structure shown="Disabled" {
                  frame Disabled {
                    n746 = control-ref of="User"() -> (w1349:refnum<vi>)
                    n747 = invoke class="Str" method="Reinit To Default"(reference=w1349) -> ()  [unwired: 2 in, 3 out]
                  }
                  frame Enabled {
                  }
                }
                n748 = flat-sequence {
                  frame #0 {
                    # "Only Default if NEW"
                    n749 = control-ref of="No."() -> (w1348:refnum<vi>)
                    n750 = invoke class="DigNum (strict)" method="Reinit To Default"(reference=w1348) -> ()  [unwired: 2 in, 3 out]
                  }
                }
                n751 = local read "CellBG Unused Cells"() -> (w1331:u32)
                n752 = call "MCListbox Refresh.vi"("color of New Cells"=w1331, "color of Blank cells"=w1331, "MulticolumnListbox in"=w1335) -> ()  [unwired: 7 in, 2 out]
                n753 = call "MCListbox Refresh.vi"("color of New Cells"=w1331, "color of Blank cells"=w1331, "MulticolumnListbox in"=w1334) -> ()  [unwired: 7 in, 2 out]
              }
              frame "Part Details Delete" {
                n754 = local read "No."() -> (w1357:i32)
                n755 = property on="Part Details" class="MCListbox (strict)"() -> ("ItemNames"=w1353:string[][])  [unwired: 2 in, 2 out]
                n756 = Format Into String(w1357) -> (resulting string=w1354:string)  [unwired: 3 in, 1 out]
                n757 = Index Array(array=w1353, index (col)=0 ("disabled index (col)")) -> (element=w1355:string[])  [unwired: 1 in]
                n758 = for {
                  tunnel: w1355 -> [w1367] mode=indexing
                  tunnel: w1354 -> [w1365]
                  shift-right: [w1361] -> w1351
                  shift-left: w1353 -> [w1363]
                  shift-right: [w1358] -> _
                  shift-left: 0 ("disabled index (col)") -> [w1359]
                  i -> [w1362]
                  n759 = call <vilib>:"Trim Whitespace.vi"("string"=w1367) -> ("trimmed string"=w1366:string)  [unwired: 1 in]
                  n760 = call <vilib>:"Trim Whitespace.vi"("string"=w1365) -> ("trimmed string"=w1364:string)  [unwired: 1 in]
                  n761 = Equal?(x=w1366, y=w1364) -> (x = y?=w1360:bool)
                  n762 = case shown="True" w1360 {
                    tunnel: w1363 -> [w1368 w1375]
                    tunnel: w1362 -> [_ w1373]
                    tunnel: [w1368 w1374] -> w1361
                    tunnel: w1359 -> [w1369 w1371]
                    tunnel: [w1369 w1370] -> w1358
                    frame False {
                    }
                    frame True {
                      n763 = Subtract(x=w1373, y=w1371) -> (x-y=w1372:i32)
                      n764 = Delete From Array(array=w1375, index (row)=w1372) -> (array with subset deleted=w1374:string[][])  [unwired: 2 in, 1 out]
                      n765 = Increment(x=w1371) -> (x+1=w1370:i32)
                    }
                  }
                }
                n766 = property on="Part Details" class="MCListbox (strict)"("ItemNames"=w1351) -> (error out=w1350:errorcluster)  [unwired: 2 in, 1 out]
              }
            }
            n767 = case shown="True" w1327 {
              frame False {
              }
              frame True {
                w1330 = "" ("Transaction No")
                n768 = local write "Transaction No 2"(w1330) -> ()
                n769 = local write "Transaction No"(w1330) -> ()
              }
            }
            n770 = flat-sequence {
              tunnel: w1329 -> [_]
              frame #0 {
                # "Reset ALL to default after delete"
                n771 = control-ref of="Setup Thermocouple Location"() -> (w1378:refnum<vi>)
                n772 = control-ref of="Channel Mapping"() -> (w1380:refnum<vi>)
                n773 = control-ref of="Notes"() -> (w1379:refnum<vi>)
                n774 = control-ref of="Item Details"() -> (w1381:refnum<vi>)
                n775 = invoke class="Str" method="Reinit To Default"(reference=w1379) -> ()  [unwired: 2 in, 3 out]
                n776 = local write "Part Details"(-1 ("Part Details")) -> ()
                n777 = property on="Part Details Add" class="Bool (strict)"("BoolText.Text"="Add" ("Boolean Text.Text")) -> ()  [unwired: 2 in, 2 out]
                n778 = invoke class="Clust (strict)" method="Reinit To Default"(reference=w1380) -> ()  [unwired: 2 in, 3 out]
                n779 = invoke class="Clust (strict)" method="Reinit To Default"(reference=w1381) -> ()  [unwired: 2 in, 3 out]
                n780 = invoke class="Pict" method="Reinit To Default"(reference=w1378) -> ()  [unwired: 2 in, 3 out]
              }
            }
          }
        }
      }
      event "Part Details": Value Change {
        # "Update Edit Fields on Top"
        n781 = event-data() -> ("CtlRef"=w1388:refnum<vi>)  [unwired: 1 in, 5 out]
        n782 = property class="MCListbox (strict)"(reference=w1388) -> ("ColHdrString"=w1386:string[], "ItemNames"=w1387:string[][], "Value"=w1382:i32)  [unwired: 1 in, 2 out]
        n783 = Index Array(array=w1387, index (row)=w1382) -> (element=w1385:string[])  [unwired: 1 in]
        n784 = case shown="0, Default" w1382 {
          tunnel: w1386 -> [w1399 _]
          tunnel: w1385 -> [w1391 _]
          frame 0, Default {
            n785 = control-ref of="Item Details"() -> (w1398:refnum<vi>)
            n786 = control-ref of="Channel Mapping"() -> (w1394:refnum<vi>)
            n787 = property class="Clust (strict)"(reference=w1398) -> ("Controls[]"=w1397:refnum<vi>[])  [unwired: 1 in, 2 out]
            n788 = property class="Clust (strict)"(reference=w1394) -> ("Controls[]"=w1393:refnum<vi>[])  [unwired: 1 in, 2 out]
            n789 = control-ref of="No."() -> (w1395:refnum<vi>)
            n790 = control-ref of="Notes"() -> (w1396:refnum<vi>)
            n791 = control-ref of="User"() -> (w1389:refnum<vi>)
            n792 = Build Array (concatenate)(w1389, w1397, w1396, w1395, w1393) -> (w1392:refnum<vi>[])
            n793 = for {
              tunnel: w1392 -> [w1426] mode=indexing
              tunnel: w1399 -> [w1423]
              tunnel: w1391 -> [w1420]
              tunnel: [w1419] -> w1390
              i -> [w1419]
              n794 = property class="Ctl"(reference=w1426) -> (reference out=w1424:refnum<vi>, "Label.Text"=w1422:string, "ClassName"=w1425:string)  [unwired: 1 in, 1 out]
              n795 = Search 1D Array(1D array=w1423, element=w1422) -> (index of element=w1421:i32)  [unwired: 1 in]
              n796 = case shown="0, Default" w1421 {
                selector: w1421 -> [w1427 _]
                tunnel: w1420 -> [w1431 _]
                tunnel: w1425 -> [w1430 _]
                tunnel: w1424 -> [w1428 _]
                frame 0, Default {
                  n797 = Index Array(array=w1431, index=w1427) -> (element=w1429:string)
                  n798 = case shown="\"Boolean\"" w1430 {
                    tunnel: w1429 -> [w1433 w1436 w1439]
                    tunnel: w1428 -> [w1432 w1435 w1440]
                    frame "Digital" {
                      n799 = Decimal String To Number(string=w1433) -> (number=w1434:i32)  [unwired: 2 in, 1 out]
                      n800 = property class="Ctl"(reference=w1432, "Value"=w1434) -> ()  [unwired: 1 in, 2 out]
                    }
                    frame "ComboBox", "String", Default {
                      n801 = property class="Ctl"(reference=w1435, "Value"=w1436) -> ()  [unwired: 1 in, 2 out]
                    }
                    frame "Boolean" {
                      n802 = Equal?(x=w1439, y="TRUE") -> (x = y?=w1437:bool)
                      n803 = property class="Ctl"(reference=w1440, "Value"=w1437) -> ()  [unwired: 1 in, 2 out]
                    }
                  }
                }
                frame -1 {
                  # "Control Label not found in MCListBox ColHdrs"
                }
              }
            }
            n804 = flat-sequence {
              tunnel: w1390 -> [_]
              frame #0 {
                w1407 = "_"
                n805 = control-ref of="Material"() -> (w1412:refnum<vi>)
                n806 = control-ref of="Revision"() -> (w1411:refnum<vi>)
                n807 = control-ref of="Material Description"() -> (w1410:refnum<vi>)
                n808 = property class="CmbBox"(reference=w1412) -> ("Value"=w1409:string)  [unwired: 1 in, 2 out]
                n809 = property class="CmbBox"(reference=w1411) -> ("Value"=w1408:string)  [unwired: 1 in, 2 out]
                n810 = property class="Str"(reference=w1410) -> ("Value"=w1406:string)  [unwired: 1 in, 2 out]
                n811 = Concatenate Strings(w1409, w1407, w1408, w1407, w1406, ".jpg" ("string")) -> (w1401:string)
                n812 = local read "MasterData\\JPG"() -> (w1402:path)
                n813 = Build Path(base path=w1402, name or relative path=w1401) -> (appended path=w1400:path)
                n814 = call <vilib>:"Check if File or Folder Exists.vi"("path"=w1400) -> ("file or folder exists?"=w1404:bool, "dup path"=w1403:path)  [unwired: 8 in, 1 out]
                n815 = case shown="True" w1404 {
                  tunnel: w1403 -> [_ w1414]
                  frame False {
                  }
                  frame True {
                    n816 = control-ref of="Setup Thermocouple Location"() -> (w1416:refnum<vi>)
                    n817 = call <vilib>:"Read JPEG File.vi"("path to JPEG file"=w1414) -> ("image data"=w1418:T34)  [unwired: 8 in, 2 out]
                    n818 = Path To String(path=w1414) -> (string=w1413:string)
                    n819 = call <vilib>:"Draw Flattened Pixmap.vi"("image data"=w1418, "picture"=picture data[5B]) -> ("new picture"=w1415:picture)  [unwired: 7 in]
                    n820 = property class="Pict"(reference=w1416, "Desc"=w1413, "Value"=w1415) -> ()  [unwired: 1 in, 2 out]
                  }
                }
              }
            }
          }
          frame -1 {
          }
        }
        n821 = case shown="-1" w1382 {
          tunnel: ["Edit" "Add"] -> w1384
          frame 0, Default {
          }
          frame -1 {
          }
        }
        n822 = control-ref of="Part Details Add"() -> (w1383:refnum<vi>)
        n823 = property on="Property Node" class="Bool (strict)"(reference=w1383, "BoolText.Text"=w1384) -> ()  [unwired: 1 in, 2 out]
      }
      event "No.": Value Change {
        n824 = event-data() -> ()  [unwired: 1 in, 6 out]
        n825 = property class="MCListbox (strict)"(reference=w1444) -> ("ItemNames"=w1447:string[][])  [unwired: 1 in, 2 out]
        n826 = local read "No."() -> (w1448:i32)
        n827 = Index Array(array=w1447, index (col)=0 ("disabled index (col)")) -> (element=w1450:string[])  [unwired: 1 in]
        n828 = Number To Decimal String(number=w1448) -> (decimal integer string=w1449:string)  [unwired: 1 in]
        n829 = Search 1D Array(1D array=w1450, element=w1449) -> (index of element=w1446:i32)  [unwired: 1 in]
        n830 = case shown="0, Default" w1446 {
          selector: w1446 -> [w1452 w1454]
          tunnel: ["Edit" "Add"] -> w1445
          tunnel: [w1452 w1454] -> w1443
          frame 0, Default {
          }
          frame -1 {
          }
        }
        n831 = property on="Part Details Add" class="Bool (strict)"("BoolText.Text"=w1445) -> ()  [unwired: 2 in, 2 out]
        n832 = property class="MCListbox (strict)"(reference=w1444, "Val(Sgnl)"=w1443) -> ()  [unwired: 1 in, 2 out]
      }
      event "No.": Key Down {
        n833 = event-data() -> ("Char"=w1457:i16, "VKey"=w1458:T31)  [unwired: 1 in, 8 out]
        n834 = case shown="\"Enter\", \"Return\"" w1458 {
          tunnel: w1457 -> [w1461 _]
          tunnel: [w1460 TRUE] -> w1456
          frame "ASCII", Default {
            n835 = Equal?(x=w1461, y=i16 9) -> (x = y?=w1460:bool)
          }
          frame "Enter", "Return" {
          }
        }
        n836 = case shown="True" w1456 {
          frame False {
          }
          frame True {
            n837 = property on="Order No." class="Str"("Key Focus"=TRUE) -> ()  [unwired: 2 in, 2 out]
          }
        }
      }
      event "Item Details.NCR No.": Value Change {
        n838 = event-data() -> ("NewVal"=w1466:string)  [unwired: 1 in, 5 out]
        n839 = Empty String/Path?(string/path=w1466) -> (empty?=w1465:bool)
        n840 = Not(x=w1465) -> (.not. x?=w1464:bool)
        n841 = property on="NCR Boolean" class="Bool (strict)"("Value"=w1464) -> ()  [unwired: 2 in, 2 out]
      }
      event "Channel Mapping", "Channel Mapping.TC1", "Channel Mapping.TC2", "Channel Mapping.TC3", "Channel Mapping.TC4", "Channel Mapping.TC5", "Channel Mapping.TC6": Key Down? {
        n842 = event-data() -> ("Char"=w1469:i16, "VKey"=w1470:T31)  [unwired: 1 in, 8 out]
        n843 = case "Only NUMBERS, BackSpace, TAB and (Up, Down, Right, Left, Delete)" shown="8, 9, 48..57" w1469 {
          tunnel: [w1477 w1480] -> w1471
          tunnel: w1470 -> [w1476 _]
          frame 0, Default {
            # "Exception"
            n844 = case shown="\"Enter\", \"Return\", \"Up\"..\"Right\", \"Delete\"" w1476 {
              tunnel: [w1478 w1479] -> w1477
              frame Default {
                w1478 = TRUE  # Discard
              }
              frame "Enter", "Return", "Up".."Right", "Delete" {
                w1479 = FALSE  # Do Not Discard
                # "Up, Down, Left, Right, Delete, Enter Return"
              }
            }
          }
          frame 8, 9, 48..57 {
            w1480 = FALSE  # Do not discard
            # "Numbers and Backspace"
          }
        }
        n845 = case shown="\"Enter\", \"Return\"" w1470 {
          selector: w1470 -> [w1472 _]
          tunnel: [w1473 w1475] -> w1468
          tunnel: w1469 -> [w1473 _]
          tunnel: [w1472 eventvkey."ASCII" ("VKey")] -> w1467
          frame "ASCII", Default {
          }
          frame "Enter", "Return" {
            w1475 = i16 9  # TAB
          }
        }
        n846 = event-data("Discard?"=w1471, "Char"=w1468, "VKey"=w1467) -> ()  [unwired: 1 in, 1 out]
      }
      event "Item Details.Order No.", "Item Details.Qty.", "Item Details.Oper. No.", "Item Details.NCR No.", "Item Details.Customer No.", "Item Details.Customer Name", "Item Details.Project", "Item Details.Sales Order", "Item Details.Item No.", "Item Details.Material", "Item Details.Revision", "Item Details.Material Description", "Item Details.Serial No.": Key Down {
        # "Move Cursor to a different field when Return, Enter or TAB is pressed"
        n847 = event-data() -> ("CtlRef"=w1481:refnum<vi>, "Char"=w1484:i16, "VKey"=w1483:T31)  [unwired: 1 in, 7 out]
        n848 = case shown="\"ASCII\", Default" w1483 {
          tunnel: w1484 -> [w1506 _]
          tunnel: [w1505 TRUE] -> w1482
          frame "ASCII", Default {
            n849 = Equal?(x=w1506, y=i16 9) -> (x = y?=w1505:bool)
          }
          frame "Enter", "Return" {
          }
        }
        n850 = case shown="True" w1482 {
          tunnel: w1481 -> [_ w1489]
          frame False {
          }
          frame True {
            n851 = disable-structure shown="Disabled" {
              frame Disabled {
                n852 = property on="Part Details Add" class="Bool (strict)"() -> ("BoolText.Text"=w1494:string)  [unwired: 2 in, 2 out]
                n853 = case shown="\"Edit\"" w1494 {
                  frame "False", Default {
                  }
                  frame "Edit" {
                    n854 = property on="Part Details Add" class="Bool (strict)"("Val(Sgnl)"=TRUE) -> ()  [unwired: 2 in, 2 out]
                  }
                }
              }
              frame Enabled {
              }
            }
            n855 = control-ref of="Item Details"() -> (w1493:refnum<vi>)
            n856 = property class="Clust (strict)"(reference=w1493) -> ("Controls[]"=w1486:refnum<vi>[])  [unwired: 1 in, 2 out]
            n857 = Search 1D Array(1D array=w1486, element=w1489) -> (index of element=w1492:i32)  [unwired: 1 in]
            n858 = property class="Ctl"(reference=w1489) -> (reference out=w1491:refnum<vi>, "Label.Text"=w1490:string)  [unwired: 1 in, 1 out]
            n859 = Increment(x=w1492) -> (x+1=w1485:i32)
            n860 = case shown="Default" w1490 {
              tunnel: w1491 -> [_ _ _]
              tunnel: [w1498 w1501 w1504] -> w1487
              tunnel: w1486 -> [w1500 w1503 _]
              tunnel: w1485 -> [w1499 w1502 _]
              frame "NCR No." {
                # "SKIP NCR Boolean and Customer No."
                n861 = Add(x=2, y=w1499) -> (x+y=w1497:i32)
                n862 = Index Array(array=w1500, index=w1497) -> (element=w1498:refnum<vi>)
              }
              frame Default {
                # "TAB to next"
                n863 = Index Array(array=w1503, index=w1502) -> (element=w1501:refnum<vi>)
              }
              frame "Serial No." {
                # "Last"
                n864 = control-ref of="TC1"() -> (w1504:refnum<vi>)
              }
            }
            n865 = property class="Ctl"(reference=w1487, "Key Focus"=TRUE) -> ()  [unwired: 1 in, 2 out]
          }
        }
      }
      event "Item Details.Material": Key Down? {
        n866 = event-data() -> ("VKey"=w1509:T31)  [unwired: 1 in, 9 out]
        n867 = case shown="\"Down\"" w1509 {
          frame "ASCII", Default {
          }
          frame "Down" {
            # "If user clicks on DOWN arrow key"
            n868 = local read "MasterData\\JPG"() -> (w1511:path)
            n869 = control-ref of="Material"() -> (w1510:refnum<vi>)
            n870 = List Folder(path=w1511, pattern="*.jpg") -> (filenames=w1512:string[])  [unwired: 2 in, 3 out]
            n871 = local write "Temp Array"(w1512) -> ()
            n872 = call "String - Extract Unique Headers_.vi"("Array In"=w1512) -> ("Array Out"=w1513:string[])  [unwired: 10 in]
            n873 = property class="CmbBox"(reference=w1510, "Strings[]"=w1513) -> ()  [unwired: 1 in, 2 out]
          }
        }
        n874 = event-data() -> ()  [unwired: 2 in, 1 out]
      }
      event "Item Details", "Channel Mapping", "Notes": Value Change {
        # "To cater for Mouse Click outside of Editing Fields"
        n875 = event-data() -> ()  [unwired: 1 in, 6 out]
        n876 = property on="Part Details Add" class="Bool (strict)"() -> ("BoolText.Text"=w1515:string)  [unwired: 2 in, 2 out]
        n877 = case shown="\"Edit\"" w1515 {
          frame "False", Default {
          }
          frame "Edit" {
            n878 = property on="Part Details Add" class="Bool (strict)"("Val(Sgnl)"=TRUE) -> ()  [unwired: 2 in, 2 out]
          }
        }
      }
      event "Channel Mapping.TC1", "Channel Mapping.TC2", "Channel Mapping.TC3", "Channel Mapping.TC4", "Channel Mapping.TC5", "Channel Mapping.TC6": Key Down {
        # "Move Cursor to a different field when Return, Enter or TAB is pressed"
        n879 = event-data() -> ("CtlRef"=w1518:refnum<vi>, "Char"=w1520:i16, "VKey"=w1519:T31)  [unwired: 1 in, 7 out]
        n880 = case shown="\"Enter\", \"Return\"" w1519 {
          tunnel: w1520 -> [w1537 _]
          tunnel: [w1536 TRUE] -> w1517
          frame "ASCII", Default {
            n881 = Equal?(x=w1537, y=i16 9) -> (x = y?=w1536:bool)
          }
          frame "Enter", "Return" {
          }
        }
        n882 = case shown="True" w1517 {
          tunnel: w1518 -> [_ w1524]
          frame False {
          }
          frame True {
            n883 = control-ref of="Channel Mapping"() -> (w1529:refnum<vi>)
            n884 = property class="Clust (strict)"(reference=w1529) -> ("Controls[]"=w1523:refnum<vi>[])  [unwired: 1 in, 2 out]
            n885 = Search 1D Array(1D array=w1523, element=w1524) -> (index of element=w1530:i32)  [unwired: 1 in]
            n886 = property class="Str"(reference=w1524) -> (reference out=w1528:refnum<vi>, "Label.Text"=w1526:string)  [unwired: 1 in, 1 out]
            n887 = Increment(x=w1530) -> (x+1=w1522:i32)
            n888 = property on="Part Details Add" class="Bool (strict)"() -> ("BoolText.Text"=w1521:string)  [unwired: 2 in, 2 out]
            n889 = case shown="Default" w1526 {
              tunnel: [w1532 w1533] -> w1525
              tunnel: w1528 -> [_ _]
              tunnel: w1523 -> [_ w1535]
              tunnel: w1522 -> [_ w1534]
              frame "TC6" {
                (unwired) TRUE ("Key Focus")
                # "Last"
                n890 = control-ref of="Notes"() -> (w1532:refnum<vi>)
              }
              frame Default {
                n891 = Index Array(array=w1535, index=w1534) -> (element=w1533:refnum<vi>)
              }
            }
            n892 = case shown="\"Edit\"" w1521 {
              frame "False", Default {
              }
              frame "Edit" {
                n893 = property on="Part Details Add" class="Bool (strict)"("Val(Sgnl)"=TRUE) -> ()  [unwired: 2 in, 2 out]
              }
            }
            n894 = property class="Ctl"(reference=w1525, "Key Focus"=TRUE) -> ()  [unwired: 1 in, 2 out]
          }
        }
      }
      event "Notes", "User": Key Down {
        # "Move Cursor to a different field when Return, Enter or TAB is pressed"
        n895 = event-data() -> ("CtlRef"=w1541:refnum<vi>, "Char"=w1543:i16, "VKey"=w1542:T31)  [unwired: 1 in, 7 out]
        n896 = case shown="\"Enter\", \"Return\"" w1542 {
          tunnel: w1543 -> [w1548 _]
          tunnel: [w1547 TRUE] -> w1540
          frame "ASCII", Default {
            n897 = Equal?(x=w1548, y=i16 9) -> (x = y?=w1547:bool)
          }
          frame "Enter", "Return" {
          }
        }
        n898 = case shown="True" w1540 {
          tunnel: w1541 -> [_ _]
          frame False {
          }
          frame True {
            n899 = property on="Part Details Add" class="Bool (strict)"() -> ("BoolText.Text"=w1544:string)  [unwired: 2 in, 2 out]
            n900 = case shown="\"Edit\"" w1544 {
              frame "False", Default {
                n901 = property on="Part Details Add" class="Bool (strict)"("Key Focus"=TRUE) -> ()  [unwired: 2 in, 2 out]
              }
              frame "Edit" {
                n902 = property on="Part Details Add" class="Bool (strict)"("Val(Sgnl)"=TRUE) -> ()  [unwired: 2 in, 2 out]
              }
            }
          }
        }
      }
      event "------------------------------------        Master Data       -----------------------------------": Value Change {
        n903 = event-data() -> ()  [unwired: 1 in, 6 out]
      }
      event "Master Data New": Value Change {
        w1561 = 3 ("dimension size")
        n904 = event-data() -> ()  [unwired: 1 in, 6 out]
        n905 = control-ref of="MCListBox FHS Master Data"() -> (w1559:refnum<vi>)
        n906 = control-ref of="WPS Details Master Data"() -> (w1558:refnum<vi>)
        n907 = property on="Master Data Temperature Units" class="Str"() -> (error out=w1557:errorcluster, "Value"=w1555:string)  [unwired: 2 in, 1 out]
        n908 = Initialize Array("", w1561) -> (w1564:string[])
        n909 = Build Array(w1564) -> (w1563:string[][])
        n910 = invoke class="Clust (strict)" method="Reinit To Default"(reference=w1558, error in=w1557) -> (error out=w1556:errorcluster)  [unwired: 1 in, 2 out]
        n911 = property on="Property Node" class="MCListbox (strict)"(reference=w1559, "ItemNames"=w1563, "NumCols"=w1561) -> (reference out=w1560:refnum<vi>)  [unwired: 1 in, 1 out]
        n912 = property on="Master Data Temperature Units" class="Str"(error in=w1556, "Value"=w1555) -> ()  [unwired: 1 in, 2 out]
        n913 = local read "CellBG Unused Cells"() -> (w1553:u32)
        n914 = local read "CellBG New Cells"() -> (w1552:u32)
        n915 = property on="Master Data Rev" class="CmbBox (strict)"("Strings[]"=string[] [] ("Strings []")) -> ()  [unwired: 2 in, 2 out]
        n916 = call "MCListbox Refresh.vi"("Which Cells"=T29."Exisiting and Blank Cells", "color of New Cells"=w1552, "color of Blank cells"=w1553, "MulticolumnListbox in"=w1560) -> ()  [unwired: 6 in, 2 out]
      }
      event "Master Data Save", "Master Data Delete": Value Change {
        n917 = event-data() -> ("CtlRef"=w1573:refnum<vi>)  [unwired: 1 in, 5 out]
        n918 = property class="Bool"(reference=w1573) -> ("Label.Text"=w1572:string)  [unwired: 1 in, 2 out]
        n919 = Unbundle By Name("WPS Details Master Data") -> ("Master Data WPS/Ref"=w1571:T5, "Master Data Rev"=w1570:T5)
        n920 = Empty String/Path?(string/path=w1571) -> (empty?=w1569:bool)
        n921 = case shown="False" w1569 {
          tunnel: w1572 -> [w1581 w1730]
          tunnel: w1571 -> [w1580 _]
          tunnel: w1570 -> [w1579 _]
          tunnel: [w1577 w1731] -> w1566
          tunnel: [w1576 FALSE ("Skip Final Prompt")] -> w1565
          frame False {
            n922 = local read "MasterData\\WPS"() -> (w1582:path)
            n923 = Concatenate Strings(w1580, "_" ("string"), w1579, ".wps" ("string")) -> (w1578:string)
            n924 = Build Path(base path=w1582, name or relative path=w1578) -> (appended path=w1585:path)
            n925 = case shown="\"Master Data Save\"" w1581 {
              tunnel: w1585 -> [w1590 w1663]
              tunnel: w1578 -> [w1588 _]
              tunnel: [w1587 w1662] -> w1577
              tunnel: [w1586 TRUE ("Skip Final Prompt")] -> w1576
              frame "Master Data Delete", Default {
                # "Master Data Delete. Same as Master Data New - need to clear everything"
                n926 = call <vilib>:"Check if File or Folder Exists.vi"("path"=w1590) -> ("file or folder exists?"=w1589:bool)  [unwired: 8 in, 2 out]
                n927 = case shown="True" w1589 {
                  tunnel: w1590 -> [w1593 w1607]
                  tunnel: w1588 -> [_ w1605]
                  tunnel: [w1592 w1602] -> w1587
                  tunnel: [TRUE ("Skip Final Prompt") w1601] -> w1586
                  frame False {
                    w1598 = "\"" ("string")
                    # "File to Delete not found"
                    n928 = Path To String(path=w1593) -> (string=w1599:string)
                    n929 = Concatenate Strings("[Delete WPS]" ("string"), " Not OK." ("string"), "\n") -> (w1595:string)
                    n930 = Concatenate Strings(w1595, w1598, w1599, w1598, " Not Found. " ("string")) -> (w1592:string)
                  }
                  frame True {
                    # "File to be deleted is found"
                    n931 = Concatenate Strings("Confirm Delete " ("string"), w1605) -> (w1604:string)
                    n932 = Two Button Dialog(message=w1604) -> (T button?=w1603:bool)  [unwired: 2 in]
                    n933 = case shown="True" w1603 {
                      tunnel: w1607 -> [_ w1632]
                      tunnel: [w1611 w1617] -> w1602
                      tunnel: [w1610 TRUE ("Skip Final Prompt")] -> w1601
                      frame False {
                        w1610 = FALSE  # Skip Final Prompt
                        # "User Cancels Delete"
                        n934 = Concatenate Strings("[Delete WPS]" ("string"), " Cancelled.", "\n") -> (w1611:string)
                      }
                      frame True {
                        w1628 = 3 ("dimension size")
                        # "User OKs delete"
                        n935 = Delete(path (use dialog)=w1632) -> (deleted path=w1618:path, error out=w1619:errorcluster)  [unwired: 4 in, 1 out]
                        n936 = control-ref of="WPS Details Master Data"() -> (w1625:refnum<vi>)
                        n937 = property on="Master Data Temperature Units" class="Str"() -> (error out=w1624:errorcluster, "Value"=w1622:string)  [unwired: 2 in, 1 out]
                        n938 = control-ref of="MCListBox FHS Master Data"() -> (w1626:refnum<vi>)
                        n939 = Initialize Array("", w1628) -> (w1631:string[])
                        n940 = Build Array(w1631) -> (w1630:string[][])
                        n941 = invoke class="Clust (strict)" method="Reinit To Default"(reference=w1625, error in=w1624) -> (error out=w1623:errorcluster)  [unwired: 1 in, 2 out]
                        n942 = property on="Property Node" class="MCListbox (strict)"(reference=w1626, "ItemNames"=w1630, "NumCols"=w1628) -> (reference out=w1627:refnum<vi>)  [unwired: 1 in, 1 out]
                        n943 = local read "CellBG Unused Cells"() -> (w1615:u32)
                        n944 = local read "CellBG New Cells"() -> (w1614:u32)
                        n945 = property on="Master Data Rev" class="CmbBox (strict)"("Strings[]"=string[] [] ("Strings []")) -> ()  [unwired: 2 in, 2 out]
                        n946 = property on="Master Data Temperature Units" class="Str"(error in=w1623, "Value"=w1622) -> ()  [unwired: 1 in, 2 out]
                        n947 = call "MCListbox Refresh.vi"("Which Cells"=T29."Exisiting and Blank Cells", "color of New Cells"=w1614, "color of Blank cells"=w1615, "MulticolumnListbox in"=w1627) -> ()  [unwired: 6 in, 2 out]
                        n948 = case shown="Error" w1619 {
                          tunnel: w1618 -> [w1641 _]
                          tunnel: [w1637 w1644] -> w1617
                          tunnel: "[Delete WPS]" ("string") -> [w1635 w1643]
                          frame No Error {
                            w1639 = "\"" ("string")
                            # "File Delete OK"
                            n949 = Path To String(path=w1641) -> (string=w1640:string)
                            n950 = Concatenate Strings(w1635, " OK." ("string"), "\n") -> (w1634:string)
                            n951 = Concatenate Strings(w1634, w1639, w1640, w1639, " deleted. " ("string")) -> (w1637:string)
                          }
                          frame Error {
                            # "File Delete Not OK"
                            n952 = Concatenate Strings(w1643, " Not OK.", "\n") -> (w1644:string)
                          }
                        }
                      }
                    }
                  }
                }
              }
              frame "Master Data Save" {
                n953 = control-ref of="MCListBox FHS Master Data"() -> (w1648:refnum<vi>)
                n954 = property class="MCListbox (strict)"(reference=w1648) -> (reference out=w1658:refnum<vi>, "ItemNames"=w1660:string[][])  [unwired: 1 in, 1 out]
                n955 = call "String - Sort Array.vi"("Check and Add Empty Row if Needed"=TRUE, "2D Array in"=w1660) -> ("2D Array out"=w1646:string[][])  [unwired: 7 in, 2 out]
                n956 = property class="MCListbox (strict)"(reference=w1658, "ItemNames"=w1646) -> (reference out=w1652:refnum<vi>)  [unwired: 1 in, 1 out]
                n957 = call "String - Check Empty Cells.vi"("ItemNames"=w1646) -> ("Rows > 0"=w1647:bool, "Location of Empty Cell (R,C)"=w1649:i32[][], "Empty Cell(s)"=w1650:bool)  [unwired: 8 in]
                n958 = call "MCListbox Event - Key Down.vi"("VKey"=eventvkey."Enter", "CtlRef"=w1652) -> ("Error Out"=w1651:errorcluster)  [unwired: 8 in, 1 out]
                n959 = local read "CellBG Unused Cells"() -> (w1654:u32)
                n960 = local read "CellBG New Cells"() -> (w1655:u32)
                n961 = call "MCListbox Refresh.vi"("Which Cells"=T29."Exisiting and Blank Cells", "Error In"=w1651, "color of New Cells"=w1655, "color of Blank cells"=w1654, "MulticolumnListbox in"=w1652) -> ("MulticolumnListbox out"=w1653:refnum<vi>)  [unwired: 5 in, 1 out]
                n962 = case shown="False" w1650 {
                  tunnel: w1663 -> [w1676 _]
                  tunnel: [w1664 w1703] -> w1662
                  tunnel: w1653 -> [w1675 _]
                  tunnel: w1649 -> [_ w1717]
                  tunnel: w1648 -> [w1669 w1718]
                  tunnel: w1647 -> [_ w1706]
                  tunnel: w1646 -> [w1671 _]
                  frame False {
                    # "No Empty Cells"
                    n963 = control-ref of="WPS Details Master Data"() -> (w1673:refnum<vi>)
                    n964 = property class="Clust (strict)"(reference=w1673) -> ("Value"=w1672:T12)  [unwired: 1 in, 2 out]
                    n965 = property class="MCListbox (strict)"(reference=w1669, "Value"=-1) -> ()  [unwired: 1 in, 2 out]
                    n966 = Unbundle By Name(w1672) -> ("Master Data Hold Temperature"=w1674:string, "Master Data Hold Time (HH:MM)"=w1668:string)
                    n967 = call "String - Check Hold Parameters.vi"("Master Data Hold Time (HH:MM)"=w1668, "Master Data Hold Temperature"=w1674, "2D Array in"=w1671) -> ("Found"=w1667:bool, "Message"=w1665:string)  [unwired: 6 in, 1 out]
                    n968 = case shown="True" w1667 {
                      tunnel: w1676 -> [_ w1681]
                      tunnel: w1675 -> [_ w1680]
                      tunnel: w1673 -> [_ w1679]
                      tunnel: ["[Save WPS] Cancelled. \n" ("string") w1678] -> w1666
                      frame False {
                      }
                      frame True {
                        n969 = call <vilib>:"Open Config Data.vi"("configuration file path"=w1681) -> ("error out"=w1688:errorcluster, "refnum"=w1689:T33)  [unwired: 8 in, 1 out]
                        n970 = call "Key - Cluster Write.vi"("error in (no error)"=w1688, "Cluster Ref in"=w1679, "Refnum in"=w1689) -> ("error out"=w1686:errorcluster, "Refnum out"=w1687:T33)  [unwired: 7 in]
                        n971 = call "Key - MCListbox Write.vi"("error in (no error)"=w1686, "MulticolumnListbox Ref in"=w1680, "refnum"=w1687) -> ("error out"=w1684:errorcluster, "Refnum out"=w1685:T33)  [unwired: 5 in, 2 out]
                        n972 = call <vilib>:"Close Config Data.vi"("error in (no error)"=w1684, "refnum"=w1685) -> ("error out"=w1682:errorcluster)  [unwired: 8 in, 1 out]
                        n973 = case shown="No Error" w1682 {
                          tunnel: w1681 -> [w1698 _]
                          tunnel: [w1694 w1701] -> w1678
                          tunnel: "[Save WPS]" ("string") -> [w1692 w1700]
                          frame No Error {
                            w1696 = "\"" ("string")
                            # "File Save OK"
                            n974 = Path To String(path=w1698) -> (string=w1697:string)
                            n975 = Concatenate Strings(w1692, " OK. " ("string"), "\n") -> (w1691:string)
                            n976 = Concatenate Strings(w1691, w1696, w1697, w1696, " saved. " ("string")) -> (w1694:string)
                          }
                          frame Error {
                            # "File Save Not OK"
                            n977 = Concatenate Strings(w1700, " Cancelled.", "\n") -> (w1701:string)
                          }
                        }
                      }
                    }
                    n978 = Concatenate Strings(w1666, w1665) -> (w1664:string)
                  }
                  frame True {
                    w1711 = 0 ("index (row)")
                    # "Empty Cells - No Saving"
                    n979 = Index Array(array=w1717, index (row) #1=w1711, index (col) #1=w1711, index (row) #2=w1711, index (col) #2=1 ("disabled index (col)")) -> (element #1=w1709:i32, element #2=w1708:i32)
                    n980 = Bundle("Numeric Control"=w1709, "Numeric Control"=w1708) -> (w1707:T35)  [unwired: 1 in]
                    n981 = property class="MCListbox (strict)"(reference=w1718, "Value"=w1709, "EditPos"=w1707) -> ()  [unwired: 1 in, 2 out]
                    n982 = for {
                      tunnel: w1717 -> [w1728] mode=indexing
                      shift-right: [w1719] -> w1715
                      shift-left: "[Save WPS] Cancelled.\nEmpty fields found in" ("string") -> [w1721]
                      n983 = Increment(x=w1728) -> (x+1=w1727:i32[])
                      n984 = Number To Decimal String(number=w1727) -> (decimal integer string=w1726:string[])  [unwired: 1 in]
                      n985 = Index Array(array=w1726) -> (element #1=w1724:string, element #2=w1722:string)  [unwired: 2 in]
                      n986 = Concatenate Strings(w1721, " R" ("string"), w1724, "C" ("string"), w1722, "," ("string")) -> (w1719:string)
                    }
                    n987 = String Length(string=w1715) -> (length=w1713:i32)
                    n988 = Decrement(x=w1713) -> (x-1=w1712:i32)
                    n989 = Replace Substring(3:w1712, 4:"." ("substring (\"\")"), 5:w1715) -> (1:w1705:string)  [unwired: 1 in, 1 out]
                    n990 = Select(t=w1705, s=w1706, f="[Save WPS] Cancelled.\nTable is empty." ("string")) -> (s? t:f=w1703:string)
                  }
                }
              }
            }
          }
          frame True {
            n991 = control-ref of="WPS Details Master Data"() -> (w1737:refnum<vi>)
            n992 = property class="Clust (strict)"(reference=w1737) -> ("Caption.Text"=w1736:string)  [unwired: 1 in, 2 out]
            n993 = case shown="\"Master Data Delete\", Default" w1730 {
              tunnel: ["[Delete WPS]" ("string") "[Save WPS]" ("string")] -> w1729
              frame "Master Data Delete", Default {
              }
              frame "Master Data Save" {
              }
            }
            n994 = Concatenate Strings(w1729, " Not OK.", "\n") -> (w1732:string)
            n995 = Concatenate Strings(w1732, w1736, " cannot be empty." ("message")) -> (w1731:string)
            n996 = One Button Dialog(message=w1731) -> ()  [unwired: 1 in, 1 out]
          }
        }
        n997 = case shown="False" w1565 {
          tunnel: w1566 -> [_ w1575]
          frame False {
          }
          frame True {
            n998 = One Button Dialog(message=w1575) -> ()  [unwired: 1 in, 1 out]
          }
        }
        n999 = Enqueue Element(queue=w1567, element=w1566, timeout in ms (-1)=w1568) -> ()  [unwired: 1 in, 3 out]
      }
      event Mouse Down? {
        n1000 = event-data() -> ("Time"=→"Time":u32, "CtlRef"=w1741:refnum<vi>)  [unwired: 1 in, 6 out]
        n1001 = local read "MasterData\\WPS"() -> (w1745:path)
        n1002 = List Folder(path=w1745, pattern="*.wps") -> (filenames=w1743:string[])  [unwired: 2 in, 3 out]
        "Temp Array" <- w1743
        n1003 = call "String - Extract Unique Headers_.vi"("Array In"=w1743) -> ("Array Out"=w1742:string[])  [unwired: 10 in]
        n1004 = property class="CmbBox (strict)"(reference=w1741, "Strings[]"=w1742) -> ()  [unwired: 1 in, 2 out]
        n1005 = event-data() -> ()  [unwired: 2 in, 1 out]
      }
      event Value Change {
        n1006 = event-data() -> ("CtlRef"=w1751:refnum<vi>)  [unwired: 1 in, 5 out]
        n1007 = property class="CmbBox (strict)"(reference=w1751) -> ("Label.Text"=w1750:string, "Value"=w1747:T5)  [unwired: 1 in, 2 out]
        n1008 = case shown="\"Additional WPS/Ref\"" w1750 {
          tunnel: [w1760 w1766 _] -> _
          tunnel: [w1759 w1765 _] -> _
          tunnel: [w1758 w1764 w1767] -> w1749
          tunnel: [w1757 w1763 _] -> _
          tunnel: w1747 -> [w1755 _ _]
          frame "WPS/Ref", Default {
            n1009 = control-ref of="WPS Details Setup"() -> ()  [unwired: 1 out]
            n1010 = control-ref of="WPS/Ref"() -> ()  [unwired: 1 out]
            n1011 = control-ref of="Rev"() -> (w1758:refnum<vi>)
            n1012 = control-ref of="Hold Temperature"() -> (w1759:refnum<vi>)
            n1013 = control-ref of="Hold Time (HH:MM)"() -> (w1757:refnum<vi>)
            n1014 = control-ref of="MCListBox FHS Setup"() -> (w1760:refnum<vi>)
            n1015 = control-ref of="Extra WPS"() -> (w1756:refnum<vi>)
            n1016 = property on="Property Node" class="Str"(reference=w1756, "Value"=w1755) -> (error out=w1754:errorcluster)  [unwired: 1 in, 1 out]
            n1017 = flat-sequence {
              tunnel: w1754 -> [_]
              frame #0 {
                n1018 = property on="Extra WPS" class="Str"("Key Focus"=TRUE, "Text.Selection"=T32 {"Selection Start"=0, "Selection End"=100}) -> ()  [unwired: 2 in, 2 out]
              }
            }
          }
          frame "Master Data WPS/Ref" {
            n1019 = control-ref of="WPS Details Master Data"() -> ()  [unwired: 1 out]
            n1020 = control-ref of="Master Data WPS/Ref"() -> ()  [unwired: 1 out]
            n1021 = control-ref of="Master Data Rev"() -> (w1764:refnum<vi>)
            n1022 = control-ref of="Master Data Hold Temperature"() -> (w1765:refnum<vi>)
            n1023 = control-ref of="Master Data Hold Time (HH:MM)"() -> (w1763:refnum<vi>)
            n1024 = control-ref of="MCListBox FHS Master Data"() -> (w1766:refnum<vi>)
          }
          frame "Additional WPS/Ref" {
            n1025 = control-ref of="Additional Rev"() -> (w1767:refnum<vi>)
          }
        }
        n1026 = local read "Temp Array"() -> (w1753:string[])
        n1027 = call "String - Extract _Body_.vi"("Temp Array"=w1753, "<wps>"=w1747) -> ("<rev>"=w1752:string[])  [unwired: 9 in]
        n1028 = property on="Property Node" class="CmbBox (strict)"(reference=w1749, "Strings[]"=w1752, "Val(Sgnl)"="") -> ()  [unwired: 1 in, 2 out]
      }
      event Value Change {
        n1029 = event-data() -> ("CtlRef"=w1788:refnum<vi>)  [unwired: 1 in, 5 out]
        n1030 = property class="CmbBox (strict)"(reference=w1788) -> (reference out=w1779:refnum<vi>, "Label.Text"=w1784:string, "Value"=w1770:T5)  [unwired: 1 in, 1 out]
        n1031 = case shown="\"Rev\", Default" w1784 {
          tunnel: [w1795 w1807] -> w1785
          tunnel: [w1798 w1805] -> w1783
          tunnel: [w1797 w1809] -> w1772
          tunnel: [w1796 w1808] -> w1771
          tunnel: [w1794 w1806] -> w1781
          tunnel: [w1793 w1804] -> _
          tunnel: w1770 -> [w1790 _]
          tunnel: [w1789 w1803] -> w1769
          tunnel: [w1789 w1802] -> w1768
          frame "Rev", Default {
            n1032 = control-ref of="WPS Details Temperature Units"() -> (w1793:refnum<vi>)
            n1033 = control-ref of="WPS Details Setup"() -> (w1794:refnum<vi>)
            n1034 = control-ref of="WPS/Ref"() -> (w1795:refnum<vi>)
            n1035 = control-ref of="Rev"() -> ()  [unwired: 1 out]
            n1036 = control-ref of="Hold Temperature"() -> (w1797:refnum<vi>)
            n1037 = control-ref of="Hold Time (HH:MM)"() -> (w1796:refnum<vi>)
            n1038 = control-ref of="MCListBox FHS Setup"() -> (w1798:refnum<vi>)
            n1039 = local read "CellBG Unused Cells"() -> (w1789:u32)
            n1040 = control-ref of="Extra Rev"() -> (w1791:refnum<vi>)
            n1041 = property on="Property Node" class="Str"(reference=w1791, "Value"=w1790) -> (error out=w1792:errorcluster)  [unwired: 1 in, 1 out]
            n1042 = disable-structure shown="Disabled" {
              disable-tunnel: w1792 -> [w1799 _]
              frame Disabled {
                n1043 = flat-sequence {
                  tunnel: w1799 -> [_]
                  frame #0 {
                    n1044 = property on="Extra Rev" class="Str"("Key Focus"=TRUE, "Text.Selection"=T32 {"Selection Start"=0, "Selection End"=100}) -> ()  [unwired: 2 in, 2 out]
                  }
                }
              }
              frame Enabled {
              }
            }
          }
          frame "Master Data Rev" {
            n1045 = control-ref of="Master Data Temperature Units"() -> (w1804:refnum<vi>)
            n1046 = control-ref of="WPS Details Master Data"() -> (w1806:refnum<vi>)
            n1047 = control-ref of="Master Data WPS/Ref"() -> (w1807:refnum<vi>)
            n1048 = control-ref of="Master Data Rev"() -> ()  [unwired: 1 out]
            n1049 = control-ref of="Master Data Hold Temperature"() -> (w1809:refnum<vi>)
            n1050 = control-ref of="Master Data Hold Time (HH:MM)"() -> (w1808:refnum<vi>)
            n1051 = control-ref of="MCListBox FHS Master Data"() -> (w1805:refnum<vi>)
            n1052 = local read "CellBG Unused Cells"() -> (w1803:u32)
            n1053 = local read "CellBG New Cells"() -> (w1802:u32)
          }
        }
        n1054 = property on="Property Node" class="CmbBox (strict)"(reference=w1785) -> ("Value"=w1778:T5)  [unwired: 1 in, 2 out]
        n1055 = Concatenate Strings(w1778, "_" ("string"), w1770, ".wps" ("string")) -> (w1776:string)
        n1056 = local read "MasterData\\WPS"() -> (w1775:path)
        n1057 = Build Path(base path=w1775, name or relative path=w1776) -> (appended path=w1786:path)
        n1058 = call <vilib>:"Check if File or Folder Exists.vi"("path"=w1786) -> ("file or folder exists?"=w1773:bool, "dup path"=w1774:path)  [unwired: 8 in, 1 out]
        n1059 = control-ref of="MCListBox FHS Master Data"() -> (w1782:refnum<vi>)
        n1060 = control-ref of="WPS Details Master Data"() -> (w1780:refnum<vi>)
        n1061 = case shown="True" w1773 {
          tunnel: w1774 -> [_ w1834]
          tunnel: w1781 -> [_ w1827]
          tunnel: w1783 -> [w1816 w1824]
          tunnel: w1780 -> [_ w1826]
          tunnel: w1782 -> [_ w1825]
          tunnel: w1779 -> [_ _]
          tunnel: w1772 -> [w1815 _]
          tunnel: w1771 -> [w1814 _]
          tunnel: w1769 -> [w1812 w1823]
          tunnel: w1768 -> [w1811 w1822]
          frame False {
            w1813 = "" ("Value")
            w1818 = 3 ("dimension size")
            n1062 = Initialize Array("", w1818) -> (w1821:string[])
            n1063 = property on="Property Node" class="Str"(reference=w1814, "Value"=w1813) -> ()  [unwired: 1 in, 2 out]
            n1064 = property on="Property Node" class="Str"(reference=w1815, "Value"=w1813) -> ()  [unwired: 1 in, 2 out]
            n1065 = Build Array(w1821) -> (w1820:string[][])
            n1066 = property on="Property Node" class="MCListbox (strict)"(reference=w1816, "ItemNames"=w1820, "NumCols"=w1818) -> (reference out=w1817:refnum<vi>)  [unwired: 1 in, 1 out]
            n1067 = call "MCListbox Refresh.vi"("Which Cells"=T29."Exisiting and Blank Cells", "color of New Cells"=w1811, "color of Blank cells"=w1812, "MulticolumnListbox in"=w1817) -> ()  [unwired: 6 in, 2 out]
          }
          frame True {
            n1068 = call <vilib>:"Open Config Data.vi"("create file if necessary (T)"=FALSE, "configuration file path"=w1834) -> ("error out"=w1840:errorcluster, "refnum"=w1841:T33)  [unwired: 7 in, 1 out]
            n1069 = call "Key - Cluster Read.vi"("error in (no error)"=w1840, "New Ctl Ref"=w1827, "Original Ctl Ref"=w1826, "Refnum in"=w1841) -> ("error out"=w1839:errorcluster, "Refnum out"=w1838:T33)  [unwired: 5 in, 1 out]
            n1070 = call "Key - MCListbox Read.vi"("error in (no error)"=w1839, "New MulticolumnListbox Ref"=w1824, "Original MulticolumnListbox Ref"=w1825, "refnum"=w1838) -> ("error out"=w1837:errorcluster, "size(s)"=w1832:i32[], "Refnum out"=w1836:T33)  [unwired: 4 in, 1 out]
            n1071 = call <vilib>:"Close Config Data.vi"("error in (no error)"=w1837, "refnum"=w1836) -> ("error out"=w1829:errorcluster)  [unwired: 8 in, 1 out]
            n1072 = Add Array Elements(numeric array=w1832) -> (sum=w1831:i32)
            n1073 = case shown="0" w1831 {
              tunnel: w1824 -> [w1843 w1847]
              tunnel: [w1843 w1846] -> w1830
              tunnel: w1829 -> [w1842 w1845]
              tunnel: [w1842 w1844] -> w1828
              frame 1, Default {
              }
              frame 0 {
                w1851 = 3 ("dimension size")
                # "Minimum 1 row"
                n1074 = Initialize Array("", w1851) -> (w1849:string[])
                n1075 = Build Array(w1849) -> (w1848:string[][])
                n1076 = property on="Property Node" class="MCListbox (strict)"(reference=w1847, error in=w1845, "ItemNames"=w1848, "NumCols"=w1851) -> (reference out=w1846:refnum<vi>, error out=w1844:errorcluster)
              }
            }
            n1077 = call "MCListbox Refresh.vi"("Which Cells"=T29."Exisiting and Blank Cells", "Error In"=w1828, "color of New Cells"=w1822, "color of Blank cells"=w1823, "MulticolumnListbox in"=w1830) -> ()  [unwired: 5 in, 2 out]
          }
        }
      }
      event "WPS Details Master Data.Master Data Hold Temperature", "WPS Details Master Data.Master Data Hold Time (HH:MM)", "WPS Details Setup.Hold Temperature", "WPS Details Setup.Hold Time (HH:MM)": Value Change {
        n1078 = event-data() -> ("CtlRef"=w1856:refnum<vi>, "NewVal"=w1854:string)  [unwired: 1 in, 4 out]
        n1079 = property class="Str"(reference=w1856) -> (reference out=w1853:refnum<vi>, "Label.Text"=w1855:string)  [unwired: 1 in, 1 out]
        n1080 = case shown="\"Hold Temperature\", \"Master Data Hold Temperature\"" w1855 {
          tunnel: w1854 -> [w1857 w1864]
          tunnel: [w1858 w1863] -> w1852
          frame "False", Default {
            # "Formats String to (HH:SS)"
            n1081 = call "String - Format to (HH_colon_MM).vi"("xx:xx"=w1857) -> ("(HH:mm)"=w1858:string)  [unwired: 9 in, 1 out]
          }
          frame "Hold Temperature", "Master Data Hold Temperature" {
            n1082 = Decimal String To Number(string=w1864) -> (number=w1862:i32)  [unwired: 2 in, 1 out]
            n1083 = In Range and Coerce(upper limit=1000 ("y"), x=w1862, lower limit=23 ("x")) -> (coerced(x)=w1859:i32)  [unwired: 1 out]
            n1084 = Number To Decimal String(number=w1859) -> (decimal integer string=w1863:string)  [unwired: 1 in]
          }
        }
        n1085 = property class="Str"(reference=w1853, "Value"=w1852) -> ()  [unwired: 1 in, 2 out]
      }
      event "WPS Details Setup.Hold Temperature", "WPS Details Setup.Hold Time (HH:MM)", "WPS Details Master Data.Master Data Hold Temperature", "WPS Details Master Data.Master Data Hold Time (HH:MM)": Key Down? {
        n1086 = event-data() -> ("Char"=w1866:i16, "VKey"=w1865:T31)  [unwired: 1 in, 8 out]
        n1087 = case "Only NUMBERS, colon, BackSpace, TAB, (Enter, Return, Up, Down, Right, Left, Delete)" shown="0, Default" w1866 {
          tunnel: [w1869 w1872] -> w1867
          tunnel: w1865 -> [w1868 _]
          frame 0, Default {
            # "Exception"
            n1088 = case shown="Default" w1868 {
              tunnel: [w1870 w1871] -> w1869
              frame Default {
                w1870 = TRUE  # Discard
              }
              frame "Enter", "Return", "Up".."Right", "Delete" {
                w1871 = FALSE  # Do Not Discard
                # "Up, Down, Left, Right, Delete"
              }
            }
          }
          frame 8, 9, 48..58 {
            w1872 = FALSE  # Do not discard
            # "Backspace, TAB, Numbers, colon"
          }
        }
        n1089 = event-data("Discard?"=w1867) -> ()  [unwired: 1 in, 1 out]
      }
      event "WPS Details Setup.Extra WPS", "WPS Details Setup.Extra Rev", "WPS Details Setup.Hold Temperature", "WPS Details Setup.Hold Time (HH:MM)", "WPS Details Master Data.Master Data Hold Temperature", "WPS Details Master Data.Master Data Hold Time (HH:MM)": Key Down {
        n1090 = event-data() -> ("CtlRef"=w1877:refnum<vi>, "Char"=w1879:i16, "VKey"=w1878:T31)  [unwired: 1 in, 7 out]
        n1091 = property on="Hold Temperature" class="Str"() -> ("OwningPane"=w1873:refnum<vi>)  [unwired: 2 in, 2 out]
        n1092 = property class="Str"(reference=w1877) -> ("OwningPane"=w1876:refnum<vi>)  [unwired: 1 in, 2 out]
        n1093 = case shown="\"ASCII\", Default" w1878 {
          tunnel: w1879 -> [w1920 _]
          tunnel: [w1919 TRUE] -> w1880
          frame "ASCII", Default {
            n1094 = Equal?(x=w1920, y=i16 9) -> (x = y?=w1919:bool)
          }
          frame "Enter", "Return" {
          }
        }
        n1095 = Equal?(x=w1873, y=w1876) -> (x = y?=w1875:bool)
        n1096 = case shown="True" w1875 {
          tunnel: [w1917 w1918] -> w1874
          frame False {
            n1097 = control-ref of="WPS Details Master Data"() -> (w1917:refnum<vi>)
          }
          frame True {
            n1098 = control-ref of="WPS Details Setup"() -> (w1918:refnum<vi>)
          }
        }
        n1099 = case shown="True" w1880 {
          tunnel: w1877 -> [_ w1887]
          tunnel: w1874 -> [_ w1883]
          frame False {
          }
          frame True {
            n1100 = property class="Clust"(reference=w1883) -> ("Controls[]"=w1885:refnum<vi>[])  [unwired: 1 in, 2 out]
            n1101 = Search 1D Array(1D array=w1885, element=w1887) -> (index of element=w1890:i32)  [unwired: 1 in]
            n1102 = property class="Str"(reference=w1887) -> (reference out=w1889:refnum<vi>, "Label.Text"=w1888:string, "Value"=w1881:string)  [unwired: 1 in, 1 out]
            n1103 = Increment(x=w1890) -> (x+1=w1884:i32)
            n1104 = case shown="\"Hold Temperature\", \"Master Data Hold Temperature\"" w1888 {
              tunnel: w1889 -> [w1892 _ _ _ _]
              tunnel: [w1899 w1903 w1907 w1911 w1914] -> w1886
              tunnel: w1885 -> [w1901 w1905 w1909 w1913 w1916]
              tunnel: w1884 -> [w1900 _ _ w1912 _]
              tunnel: [TRUE ("Key Focus") TRUE ("Key Focus") TRUE ("Key Focus") TRUE ("Key Focus") _] -> w1882
              tunnel: w1881 -> [w1893 _ _ _ _]
              frame "Hold Temperature", "Master Data Hold Temperature" {
                # "Min 25 degC, SKIP Temperature Units"
                n1105 = Decimal String To Number(string=w1893) -> (number=w1896:i32)  [unwired: 2 in, 1 out]
                n1106 = Max & Min(x=23, y=w1896) -> (max(x,y)=w1894:i32)  [unwired: 1 out]
                n1107 = Number To Decimal String(number=w1894) -> (decimal integer string=w1891:string)  [unwired: 1 in]
                n1108 = property class="Str"(reference=w1892, "Value"=w1891) -> ()  [unwired: 1 in, 2 out]
                n1109 = Increment(x=w1900) -> (x+1=w1897:i32)
                n1110 = Index Array(array=w1901, index=w1897) -> (element=w1899:refnum<vi>)
              }
              frame "Extra Rev" {
                # "Goto Hold Tempeterature"
                n1111 = Index Array(array=w1905, index=2) -> (element=w1903:refnum<vi>)
              }
              frame "Rev" {
                # "Goto WPS"
                n1112 = Index Array(array=w1909, index=5) -> (element=w1907:refnum<vi>)
              }
              frame Default {
                # "TAB to next"
                n1113 = Index Array(array=w1913, index=w1912) -> (element=w1911:refnum<vi>)
              }
              frame "Hold Time (HH:MM)", "Master Data Hold Time (HH:MM)" {
                # "Last"
                n1114 = Index Array(array=w1916, index=0) -> (element=w1914:refnum<vi>)
              }
            }
            n1115 = property class="Ctl"(reference=w1886, "Key Focus"=w1882) -> ()  [unwired: 1 in, 2 out]
          }
        }
      }
      event "---------------------------------       Master Data (Material)      -----------------------------": Value Change {
        n1116 = event-data() -> ()  [unwired: 1 in, 6 out]
      }
      event "Material New": Value Change {
        w1923 = ""
        n1117 = event-data() -> ()  [unwired: 1 in, 6 out]
        n1118 = control-ref of="Master Data Material Description"() -> (w1924:refnum<vi>)
        n1119 = control-ref of="Master Data Thermocouple Location"() -> (w1925:refnum<vi>)
        n1120 = invoke class="Pict" method="Reinit To Default"(reference=w1925) -> ()  [unwired: 2 in, 3 out]
        n1121 = invoke class="Str" method="Reinit To Default"(reference=w1924) -> ()  [unwired: 2 in, 3 out]
        n1122 = property on="Master Data Material" class="CmbBox"("Value"=w1923) -> ()  [unwired: 2 in, 2 out]
        n1123 = property on="Master Data Rev" class="CmbBox"("Value"=w1923) -> ()  [unwired: 2 in, 2 out]
      }
      event "Material Save", "Material Delete": Value Change {
        n1124 = event-data() -> ("CtlRef"=w1936:refnum<vi>)  [unwired: 1 in, 5 out]
        n1125 = Unbundle By Name("Material") -> ("Master Data Material"=w1932:string, "Master Data Rev"=w1931:string, "Master Data Material Description"=w1933:string)
        n1126 = property class="Bool"(reference=w1936) -> ("Label.Text"=w1935:string)  [unwired: 1 in, 2 out]
        n1127 = Empty String/Path?(string/path=w1932) -> (empty?=w1926:bool)
        n1128 = case shown="False" w1926 {
          tunnel: w1935 -> [w1951 _]
          tunnel: [w1947 _] -> _
          tunnel: w1933 -> [w1946 _]
          tunnel: w1932 -> [w1942 _]
          tunnel: w1931 -> [w1941 _]
          tunnel: [w1939 "[Save/Delete Material] Some Fields Are Invalid." ("string")] -> w1928
          tunnel: [w1938 FALSE] -> w1927
          frame False {
            w1950 = "_"
            # "Valid Fields"
            n1129 = local read "MasterData\\JPG"() -> (w1944:path)
            n1130 = Concatenate Strings(w1942, w1950, w1941, w1950) -> (w1943:string)
            n1131 = local read "Image File Path"() -> (w1949:path)
            n1132 = Concatenate Strings(w1943, w1946, ".jpg" ("string")) -> (w1940:string)
            n1133 = Build Path(base path=w1944, name or relative path=w1940) -> (appended path=w1948:path)
            n1134 = case shown="\"Material Save\"" w1951 {
              tunnel: w1949 -> [_ w1994]
              tunnel: w1948 -> [w1953 w1982]
              tunnel: [w1958 w1983] -> w1947
              tunnel: w1944 -> [_ w1992]
              tunnel: w1943 -> [_ w1993]
              tunnel: w1940 -> [_ _]
              tunnel: [w1957 w1981] -> w1939
              tunnel: [w1956 TRUE] -> w1938
              frame "Material Delete", Default {
                n1135 = Delete(path (use dialog)=w1953, confirm (F)=TRUE) -> (cancelled=w1954:bool, error out=w1952:errorcluster)  [unwired: 3 in, 1 out]
                n1136 = case shown="False" w1954 {
                  tunnel: w1953 -> [w1962 _]
                  tunnel: [w1959 _] -> w1958
                  tunnel: [w1961 "[Delete Material] Cancelled By User." ("string")] -> w1957
                  tunnel: [TRUE _] -> w1956
                  tunnel: w1952 -> [w1959 _]
                  frame False {
                    n1137 = control-ref of="Master Data Material Description"() -> (w1964:refnum<vi>)
                    n1138 = control-ref of="Master Data Thermocouple Location"() -> (w1965:refnum<vi>)
                    n1139 = invoke class="Pict" method="Reinit To Default"(reference=w1965) -> ()  [unwired: 2 in, 3 out]
                    n1140 = invoke class="Str" method="Reinit To Default"(reference=w1964) -> ()  [unwired: 2 in, 3 out]
                    n1141 = case shown="No Error" w1959 {
                      tunnel: w1962 -> [w1974 _]
                      tunnel: [w1970 w1977] -> w1961
                      tunnel: "[Delete Material]" ("string") -> [w1968 w1976]
                      frame No Error {
                        w1972 = "\"" ("string")
                        # "File Delete OK"
                        n1142 = Path To String(path=w1974) -> (string=w1973:string)
                        n1143 = Concatenate Strings(w1968, " OK." ("string"), "\n") -> (w1967:string)
                        n1144 = Concatenate Strings(w1967, w1972, w1973, w1972, " deleted. " ("string")) -> (w1970:string)
                      }
                      frame Error {
                        # "File Delete Not OK"
                        n1145 = Concatenate Strings(w1976, " Not OK.", "\n") -> (w1977:string)
                      }
                    }
                  }
                  frame True {
                  }
                }
              }
              frame "Material Save" {
                n1146 = Concatenate Strings(w1993, "*.*" ("string")) -> (w1986:string)
                n1147 = List Folder(path=w1992, pattern=w1986) -> (path out=w1988:path, filenames=w1987:string[])  [unwired: 2 in, 2 out]
                n1148 = for {
                  tunnel: w1988 -> [w2014]
                  tunnel: w1987 -> [w2013] mode=indexing
                  tunnel: [w2012] -> w1990 mode=indexing
                  tunnel: w1982 -> [w2011]
                  # "Delete all other <material>_<rev>_*.*"
                  n1149 = Build Path(base path=w2014, name or relative path=w2013) -> (appended path=w2010:path)
                  n1150 = Not Equal?(x=w2010, y=w2011) -> (x != y?=w2009:bool)
                  n1151 = case shown="True" w2009 {
                    tunnel: [_ w2016] -> w2012
                    tunnel: w2010 -> [_ w2015]
                    frame False {
                    }
                    frame True {
                      n1152 = Delete(path (use dialog)=w2015) -> (error out=w2016:errorcluster)  [unwired: 4 in, 2 out]
                    }
                  }
                }
                n1153 = Copy(9:TRUE ("overwrite (F)"), 10:w1982, 11:w1994) -> (0:w1991:errorcluster)  [unwired: 2 in, 2 out]
                n1154 = Merge Errors(w1991, w1990) -> (w1983:errorcluster)
                n1155 = case shown="Error" w1983 {
                  tunnel: w1982 -> [w2003 _]
                  tunnel: [w1999 w2007] -> w1981
                  tunnel: "[Save Material]" ("string") -> [w1997 w2006]
                  frame No Error {
                    w2001 = "\"" ("string")
                    # "File Save OK"
                    n1156 = Path To String(path=w2003) -> (string=w2002:string)
                    n1157 = Concatenate Strings(w1997, " OK." ("string"), "\n") -> (w1996:string)
                    n1158 = Concatenate Strings(w1996, w2001, w2002, w2001, " saved. " ("string")) -> (w1999:string)
                  }
                  frame Error {
                    # "File Save Not OK"
                    n1159 = Concatenate Strings(w2006, " Not OK.", "\n", "Possibe Cause: Browsed Material file is the same as Material file to be saved." ("string")) -> (w2007:string)
                  }
                }
              }
            }
          }
          frame True {
            # "Some Fields are empty"
            n1160 = One Button Dialog(message="Some Fields Are Invalid") -> ()  [unwired: 1 in, 1 out]
          }
        }
        n1161 = case shown="True" w1927 {
          tunnel: w1928 -> [_ w1937]
          frame False {
          }
          frame True {
            n1162 = One Button Dialog(message=w1937) -> ()  [unwired: 1 in, 1 out]
          }
        }
        n1163 = Enqueue Element(queue=w1929, element=w1928, timeout in ms (-1)=w1930) -> ()  [unwired: 1 in, 3 out]
      }
      event "Material Browse": Value Change {
        n1164 = event-data() -> ()  [unwired: 1 in, 6 out]
        n1165 = local read "MasterData\\JPG"() -> (w2024:path)
        n1166 = call "File Dialog2"("start path"=w2024, "prompt"="Select Material image", "pattern (all files)"="*.jpg;*.jpeg") -> ("selected path"=w2023:path, "exists"=w2022:bool, "error out"=w2021:errorcluster)  [unwired: 9 in, 1 out]
        n1167 = case shown="True" w2022 {
          tunnel: w2023 -> [_ w2027]
          tunnel: w2021 -> [_ _]
          frame False {
          }
          frame True {
            n1168 = call <vilib>:"Read JPEG File.vi"("path to JPEG file"=w2027) -> ("image data"=w2026:T34)  [unwired: 8 in, 2 out]
            n1169 = call <vilib>:"Draw Flattened Pixmap.vi"("image data"=w2026, "picture"=picture data[5B]) -> ("new picture"=→"Master Data Thermocouple Location":picture)  [unwired: 7 in]
            "Image File Path" <- w2027
          }
        }
      }
      event "Material.Master Data Material", "Item Details.Material": Mouse Down? {
        n1170 = event-data() -> ("CtlRef"=w2032:refnum<vi>)  [unwired: 1 in, 7 out]
        n1171 = local read "MasterData\\JPG"() -> (w2030:path)
        n1172 = List Folder(path=w2030, pattern="*.jpg") -> (filenames=w2031:string[])  [unwired: 2 in, 3 out]
        n1173 = local write "Temp Array"(w2031) -> ()
        n1174 = call "String - Extract Unique Headers_.vi"("Array In"=w2031) -> ("Array Out"=w2033:string[])  [unwired: 10 in]
        n1175 = property class="CmbBox"(reference=w2032, "Strings[]"=w2033) -> ()  [unwired: 1 in, 2 out]
        n1176 = event-data() -> ()  [unwired: 2 in, 1 out]
      }
      event "Material.Master Data Material", "Item Details.Material": Value Change {
        n1177 = event-data() -> ("CtlRef"=w2037:refnum<vi>)  [unwired: 1 in, 5 out]
        n1178 = property class="CmbBox"(reference=w2037) -> ("Label.Text"=w2038:string, "Value"=w2039:string)  [unwired: 1 in, 2 out]
        n1179 = local read "Temp Array"() -> (w2043:string[])
        n1180 = call "String - Extract _Body_.vi"("Temp Array"=w2043, "<wps>"=w2039) -> ("<rev>"=w2041:string[])  [unwired: 9 in]
        n1181 = case shown="\"Setup Material\", Default" w2038 {
          tunnel: [w2046 w2049] -> w2042
          tunnel: [w2045 w2048] -> w2036
          tunnel: [w2044 w2047] -> w2035
          frame "Setup Material", Default {
            n1182 = control-ref of="Revision"() -> (w2046:refnum<vi>)
            n1183 = control-ref of="Setup Thermocouple Location"() -> (w2044:refnum<vi>)
            n1184 = control-ref of="Material Description"() -> (w2045:refnum<vi>)
          }
          frame "Master Data Material" {
            n1185 = control-ref of="Master Data Thermocouple Location"() -> (w2047:refnum<vi>)
            n1186 = control-ref of="Master Data Material Description"() -> (w2048:refnum<vi>)
            n1187 = control-ref of="Master Data Rev"() -> (w2049:refnum<vi>)
          }
        }
        n1188 = property class="CmbBox"(reference=w2042, "Strings[]"=w2041, "Val(Sgnl)"="") -> ()  [unwired: 1 in, 2 out]
        n1189 = invoke class="Pict" method="Reinit To Default"(reference=w2035) -> ()  [unwired: 2 in, 3 out]
        n1190 = invoke class="Str" method="Reinit To Default"(reference=w2036) -> ()  [unwired: 2 in, 3 out]
      }
      event "Material.Master Data Rev", "Item Details.Revision": Value Change {
        w2070 = "_" ("string")
        n1191 = event-data() -> ("CtlRef"=w2071:refnum<vi>)  [unwired: 1 in, 5 out]
        n1192 = property class="CmbBox"(reference=w2071) -> ("Label.Text"=w2050:string, "Value"=w2056:string)  [unwired: 1 in, 2 out]
        n1193 = case shown="\"Revision\", Default" w2050 {
          tunnel: [w2078 w2081] -> w2054
          tunnel: [w2077 w2080] -> w2052
          tunnel: [w2076 w2079] -> w2053
          frame "Revision", Default {
            n1194 = control-ref of="Material"() -> (w2078:refnum<vi>)
            n1195 = control-ref of="Setup Thermocouple Location"() -> (w2076:refnum<vi>)
            n1196 = control-ref of="Material Description"() -> (w2077:refnum<vi>)
          }
          frame "Master Data Rev" {
            n1197 = control-ref of="Master Data Thermocouple Location"() -> (w2079:refnum<vi>)
            n1198 = control-ref of="Master Data Material"() -> (w2081:refnum<vi>)
            n1199 = control-ref of="Master Data Material Description"() -> (w2080:refnum<vi>)
          }
        }
        n1200 = property on="Property Node" class="CmbBox"(reference=w2054) -> ("Value"=w2055:string)  [unwired: 1 in, 2 out]
        n1201 = Concatenate Strings(w2055, w2070, w2056, w2070) -> (w2061:string)
        n1202 = Concatenate Strings(w2061, "*.jpg" ("string")) -> (w2060:string)
        n1203 = local read "MasterData\\JPG"() -> (w2067:path)
        n1204 = List Folder(path=w2067, pattern=w2060) -> (filenames=w2069:string[])  [unwired: 2 in, 3 out]
        n1205 = Index Array(array=w2069, index=0) -> (element=w2063:string)
        n1206 = Match Pattern(string=w2063, regular expression=w2061) -> (after substring=w2059:string)  [unwired: 1 in, 3 out]
        n1207 = Build Path(base path=w2067, name or relative path=w2063) -> (appended path=w2066:path)
        n1208 = Match Pattern(string=w2059, regular expression="[.]") -> (before substring=w2057:string)  [unwired: 1 in, 3 out]
        n1209 = call <vilib>:"Check if File or Folder Exists.vi"("path"=w2066) -> ("file or folder exists?"=w2065:bool, "dup path"=w2064:path)  [unwired: 8 in, 1 out]
        n1210 = property class="Str"(reference=w2052, "Value"=w2057) -> ()  [unwired: 1 in, 2 out]
        n1211 = case shown="True" w2065 {
          tunnel: w2064 -> [_ w2087]
          tunnel: w2053 -> [w2083 w2089]
          tunnel: w2052 -> [w2084 _]
          tunnel: [w2082 _] -> w2051
          tunnel: w2050 -> [_ w2086]
          frame False {
            n1212 = invoke class="Str" method="Reinit To Default"(reference=w2084) -> (error out=w2082:errorcluster)  [unwired: 2 in, 2 out]
            n1213 = invoke class="Pict" method="Reinit To Default"(reference=w2083) -> ()  [unwired: 2 in, 3 out]
          }
          frame True {
            n1214 = Path To String(path=w2087) -> (string=w2085:string)
            n1215 = case shown="\"Revision\"" w2086 {
              tunnel: w2085 -> [_ w2092]
              frame "False", Default {
              }
              frame "Revision" {
                n1216 = property on="Material Filename" class="Str"("Value"=w2092) -> ()  [unwired: 2 in, 2 out]
              }
            }
            n1217 = local write "Image File Path"(w2087) -> ()
            n1218 = call <vilib>:"Read JPEG File.vi"("path to JPEG file"=w2087) -> ("image data"=w2091:T34)  [unwired: 8 in, 2 out]
            n1219 = call <vilib>:"Draw Flattened Pixmap.vi"("image data"=w2091, "picture"=picture data[5B]) -> ("new picture"=w2090:picture)  [unwired: 7 in]
            n1220 = property on="Property Node" class="Pict"(reference=w2089, "Value"=w2090, "Desc"=w2085) -> ()  [unwired: 1 in, 2 out]
          }
        }
        n1221 = disable-structure shown="Disabled" {
          disable-tunnel: w2051 -> [w2073 _]
          disable-tunnel: w2050 -> [w2072 _]
          frame Disabled {
            n1222 = case shown="\"Revision\"" w2072 {
              tunnel: w2073 -> [_ _]
              frame "False", Default {
              }
              frame "Revision" {
                # "Do a Part Details Add to update table once Revision is selected"
                n1223 = property on="Part Details Add" class="Bool (strict)"() -> ("BoolText.Text"=w2074:string)  [unwired: 2 in, 2 out]
                n1224 = case shown="\"Edit\"" w2074 {
                  frame "False", Default {
                  }
                  frame "Edit" {
                    n1225 = property on="Part Details Add" class="Bool (strict)"("Val(Sgnl)"=TRUE) -> ()  [unwired: 2 in, 2 out]
                  }
                }
              }
            }
          }
          frame Enabled {
          }
        }
      }
    }
  }
  n1226 = while {
    shift-right: [w2104] -> _
    shift-left: Enum_-_SRTRS_State."READY TO START" ("Enum") -> [w2100]
    shift-right: [w2113] -> _
    shift-left: w9 -> [w2112]
    shift-right: [w2105] -> _
    shift-left: w24 -> [w2111]
    shift-right: [w2107] -> _
    shift-left: w8 -> [w2108]
    tunnel: [w2103] -> w21
    tunnel: w17 -> [w2106]
    shift-left: Enum_-_SRTRS_State."QUIT" ("Enum") -> [w2101]
    shift-right: [w2097] -> _
    shift-left: ET3500_Program_Status."Wait For RUN" -> [w2098]
    shift-right: [w2096] -> _
    shift-left: w5 -> [w2095]
    stop <- w2103 stop-if-true
    # "StateMachine For MainProcess"
    n1227 = Format Into String(w2100) -> (resulting string=→"State":string)  [unwired: 3 in, 1 out]
    n1228 = case shown="\"READY TO START\", Default" w2100 {
      selector: w2100 -> [w2139 _ _ _ w2342 _ _ _ _ _ _ w2685]
      tunnel: [w2140 Enum_-_SRTRS_State."START Recovery" ("Enum") Enum_-_SRTRS_State."BEGIN Process" ("Enum") Enum_-_SRTRS_State."RUNNING Process" ("Enum") w2343 Enum_-_SRTRS_State."ERROR Handling" ("Enum") Enum_-_SRTRS_State."END Recipe" ("Enum") Enum_-_SRTRS_State."ERROR Handling" ("Enum") w2555 Enum_-_SRTRS_State."READY TO START" ("Enum") w2631 w2685] -> w2110
      tunnel: [_ 0 ("Index") w2282 w2300 w2320 w2529 w2534 w2539 w2544 w2568 w2623 _] -> w2113
      tunnel: w2112 -> [_ _ w2282 w2300 w2320 w2529 w2534 w2539 w2547 _ w2623 _]
      tunnel: [w2126 w2233 _ w2291 w2324 w2528 _ w2540 _ w2572 w2628 w2681] -> w2105
      tunnel: w2111 -> [_ _ _ _ _ w2528 _ w2540 _ _ w2626 _]
      tunnel: [_ _ _ _ _ _ _ _ _ _ w2630 TRUE] -> w2103
      tunnel: w2108 -> [_ _ _ _ w2318 _ w2531 w2538 _ _ w2624 _]
      tunnel: [w2128 0 _ _ w2333 _ w2531 w2538 0 _ w2624 _] -> w2107
      tunnel: w2106 -> [w2136 w2245 w2284 w2301 w2316 _ w2535 _ w2553 w2571 w2636 w2682]
      tunnel: 1000 ("timeout in ms (-1)") -> [w2137 w2239 w2277 w2299 w2315 _ w2533 _ w2552 w2569 w2627 w2680]
      tunnel: w2101 -> [w2138 _ _ _ _ _ _ _ _ _ w2625 _]
      tunnel: w2098 -> [_ _ _ _ w2330 _ _ _ _ _ w2622 _]
      tunnel: [_ _ _ ET3500_Program_Status."Wait For RUN" w2329 _ _ _ _ _ w2622 _] -> w2097
      tunnel: [_ _ _ _ w2327 _ _ _ _ _ w2621 _] -> w2096
      tunnel: w2095 -> [_ _ _ _ w2326 _ _ _ _ _ w2621 _]
      tunnel: string[] ["1"] ("Index") -> [_ _ w2275 _ _ _ _ _ w2542 _ _ _]
      frame "READY TO START", Default {
        n1229 = local read "Tab Body"() -> (w2125:T1)
        n1230 = local read "Transaction No"() -> (w2134:string)
        n1231 = Equal?(x=w2139, y=w2138) -> (x = y?=w2124:bool)
        n1232 = case shown="\"Setup\", Default" w2125 {
          tunnel: [_ w2159] -> w2128
          tunnel: [FALSE ("DAQ Start") w2158] -> w2127
          tunnel: [_ w2157] -> w2126
          tunnel: w2124 -> [_ _]
          frame "Setup", Default {
            n1233 = First Call?() -> (First Call?: T/F=w2145:bool)
            n1234 = case shown="True" w2145 {
              frame False {
              }
              frame True {
                # "Folder Maintanence for both cRIO and Host."
                n1235 = local read "Logs_Host"() -> (w2152:path)
                n1236 = Format Date/Time String "Date_Time"(time format string (%c)="%Y%m") -> (date/time string=w2150:string)  [unwired: 2 in]
                n1237 = call "Folder - Subtract Number of Months.vi"("- # of Months"=3, "YYYYmm"=w2150, "Folder"=w2152) -> ("< Range (Folder\\YYYY\\mm)"=w2148:path[])  [unwired: 6 in, 2 out]
                n1238 = for {
                  tunnel: w2148 -> [w2154] mode=indexing
                  n1239 = Delete(path (use dialog)=w2154, entire hierarchy (F)=TRUE) -> ()  [unwired: 3 in, 3 out]
                }
              }
            }
            n1240 = local write "Time to next sample (s)"(0.0 ("Scale.Range:Maximum")) -> ()
            n1241 = local write "Time Target (s)"(0.0 ("Time Target (s)")) -> ()
          }
          frame "Execute" {
            n1242 = call "Elapsed Time"("Time Target (s)"="Time Target (s)") -> ("Time has Elapsed"=w2155:bool)  [unwired: 11 in, 7 out]
            n1243 = case shown="True" w2155 {
              tunnel: [_ w2177] -> w2159
              tunnel: [_ w2160] -> w2158
              tunnel: [_ w2172] -> w2157
              frame False {
              }
              frame True {
                n1244 = local read "cRIO shared variable RT Library"() -> (w2179:string)
                n1245 = local write "Time Target (s)"(10.0 ("Time Target (s)")) -> ()
                n1246 = local read "VISA resource name RS232"() -> (w2175:string)
                n1247 = control-ref of="cRIO Status"() -> (w2162:refnum<vi>)
                n1248 = control-ref of="ET3504 Status"() -> (w2163:refnum<vi>)
                n1249 = call "cRIO - Shared Variable RW.vi"("shared variable RT Library"=w2179, "Read/Write"=enum16{"Write", "Read"}."Read", "Simulate cRIO"="Simulate cRIO", "cRIO Status"=w2162) -> ("Probe List Out"=w2168:i32[], "cRIO Timestamp"=→"cRIO Timestamp (only updated when a Shared Variable is Read)":timestamp, "Data Path Name"=→"Data Path Name":string, "Cycle Count"=w2177:i32, "DAQ Started"=w2160:bool, "Error Out"=w2164:errorcluster)  [unwired: 7 in, 3 out]
                "cRIO DAQ Start" <- w2160
                "cRIO Cycle Count" <- w2177
                "cRIO Error" <- w2164
                n1250 = call "ET3500 - Read Program Parameters.vi"("Simulate"="Simulate ET3500", "ET3500 Status"=w2163, "error in (no error)"=w2164, "subVI (Auto Interactive)"=TRUE ("subVI"), "Option"=cluster{"Init":bool, "Close":bool} {"Init"=TRUE, "Close"=TRUE}, "VISA resource name"=w2175) -> ("error out"=w2173:errorcluster, "Parameter Cluster (Scaled)"=w2167:T36)  [unwired: 1 in, 3 out]
                "ET3500 Error" <- w2173
                n1251 = Unbundle By Name(w2167) -> ("PVIn (degC)"=w2166:dbl)
                n1252 = property on="Current Temp" class="DigNum (strict)"("Value"=w2166) -> ()  [unwired: 2 in, 2 out]
                n1253 = Merge Errors(w2173, w2164) -> (w2172:errorcluster)
                n1254 = case shown="True" w2160 {
                  tunnel: w2168 -> [_ w2214]
                  frame False {
                  }
                  frame True {
                    # "DAQ Started, Probe already Loaded in"
                    n1255 = local write "Probe List"(w2214) -> ()
                  }
                }
                n1256 = case shown="True" w2160 {
                  frame False {
                  }
                  frame True {
                    # "Recovery"
                    n1257 = local read "Latest stp file"() -> (w2182:path)
                    n1258 = call <vilib>:"Check if File or Folder Exists.vi"("path"=w2182) -> ("file or folder exists?"=w2181:bool, "dup path"=w2180:path)  [unwired: 8 in, 1 out]
                    n1259 = case shown="True" w2181 {
                      tunnel: w2180 -> [_ w2210]
                      frame False {
                      }
                      frame True {
                        n1260 = Strip Path(path=w2210) -> (name=w2211:string)  [unwired: 1 out]
                        n1261 = control-ref of="WPS Details Buffer"() -> (w2196:refnum<vi>)
                        n1262 = Match Pattern(string=w2211, regular expression="_") -> (before substring=w2212:string)  [unwired: 1 in, 3 out]
                        n1263 = call <vilib>:"Open Config Data.vi"("create file if necessary (T)"=FALSE, "configuration file path"=w2210) -> ("error out"=w2206:errorcluster, "refnum"=w2208:T33)  [unwired: 7 in, 1 out]
                        n1264 = control-ref of="WPS Details Setup"() -> (w2207:refnum<vi>)
                        n1265 = local write "Transaction No"(w2212) -> ()
                        n1266 = local write "Transaction No 2"(w2212) -> ()
                        n1267 = call "Key - Cluster Read.vi"("error in (no error)"=w2206, "New Ctl Ref"=w2196, "Original Ctl Ref"=w2207, "Refnum in"=w2208) -> ("error out"=w2193:errorcluster, "Refnum out"=w2194:T33)  [unwired: 5 in, 1 out]
                        n1268 = control-ref of="Parameter Buffer"() -> (w2192:refnum<vi>)
                        n1269 = call "Key - Cluster Read.vi"("error in (no error)"=w2193, "New Ctl Ref"=w2192, "Original Ctl Ref"=w2192, "Refnum in"=w2194) -> ("error out"=w2189:errorcluster, "Refnum out"=w2191:T33)  [unwired: 5 in, 1 out]
                        n1270 = control-ref of="Final Target Temperature"() -> (w2187:refnum<vi>)
                        n1271 = call "Key - Cluster Read.vi"("error in (no error)"=w2189, "New Ctl Ref"=w2187, "Original Ctl Ref"=w2187, "Refnum in"=w2191) -> ("error out"=w2188:errorcluster, "Refnum out"=w2190:T33)  [unwired: 5 in, 1 out]
                        n1272 = call <vilib>:"Close Config Data.vi"("error in (no error)"=w2188, "write file if changed (T)"=FALSE, "refnum"=w2190) -> ("error out"=w2195:errorcluster)  [unwired: 7 in, 1 out]
                        n1273 = local write "stp file Error Out"(w2195) -> ()
                        n1274 = property class="Clust (strict)"(reference=w2196, error in=w2195) -> (error out=w2197:errorcluster, "Value"=w2204:T7)  [unwired: 1 out]
                        n1275 = Unbundle By Name(w2204) -> ("WPS/Ref"=w2200:T5, "WPS Details Temperature Units"=w2201:string, "Hold Temperature"=w2202:string, "Hold Time (HH:MM)"=w2203:string)
                        n1276 = local write "Property Node Error"(w2197) -> ()
                        n1277 = local read "Info."() -> (w2198:T8)
                        n1278 = Bundle By Name(cluster=w2198, "Info. WPS/Ref."=w2200, "Info. Temperature Units"=w2201, "Info. Temperature Units 2"=w2201, "Hold. Temp."=w2202, "Hold. Time (hour:minute)"=w2203) -> (w2199:T8)
                        n1279 = local write "Info."(w2199) -> ()
                      }
                    }
                    n1280 = disable-structure shown="Disabled" {
                      frame Disabled {
                        # "Recover Transaction No from Data Path Name (from cRIO)"
                        n1281 = local read "Data Path Name"() -> (w2186:string)
                        n1282 = Reverse String(1:w2186) -> (0:w2183:string)
                        n1283 = Match Pattern(string=w2183, regular expression="./") -> (before substring=w2185:string)  [unwired: 1 in, 3 out]
                        n1284 = Reverse String(1:w2185) -> ()  [unwired: 1 out]
                      }
                      frame Enabled {
                      }
                    }
                  }
                }
              }
            }
          }
        }
        n1285 = Empty String/Path?(string/path=w2134) -> (empty?=w2133:bool)
        n1286 = case shown="False" w2124 {
          tunnel: w2137 -> [w2217 _]
          tunnel: w2136 -> [w2215 _]
          frame False {
            # "1st Time"
            n1287 = Enqueue Element(queue=w2215, element="Ready to Start.", timeout in ms (-1)=w2217) -> ()  [unwired: 1 in, 3 out]
          }
          frame True {
            # "Repeating READY TO START"
          }
        }
        n1288 = Select(t=T27."Disabled and Grayed Out" ("Disabled"), s=w2133, f=T27."Enabled" ("Disabled")) -> (s? t:f=w2135:T27)
        n1289 = Wait Until Next ms Multiple(millisecond multiple=u32 100) -> ()  [unwired: 1 out]
        n1290 = property on="Recipe Start" class="Bool"("DisabledEnum"=w2135) -> ()  [unwired: 2 in, 2 out]
        n1291 = property on="Close" class="Bool (strict)"("DisabledEnum"=T27."Enabled" ("Disabled")) -> ()  [unwired: 2 in, 2 out]
        n1292 = local read "Recipe Start Flag"() -> (w2130:bool)
        n1293 = Or(x=w2130, y=w2127) -> (x .or. y?=w2129:bool)
        n1294 = Select(t=Enum_-_SRTRS_State."START Recipe" ("Enum"), s=w2129, f=Enum_-_SRTRS_State."READY TO START" ("Enum")) -> (s? t:f=w2140:T16)
      }
      frame "START Recipe" {
        w2229 = T23 [enum."Page Disabled & Grayed", enum."Page Enabled", enum."Page Disabled & Grayed", enum."Page Disabled & Grayed", enum."Page Enabled"] items=["Page Enabled", "Page Disabled", "Page Disabled & Grayed"]
        w2242 = "\"" ("string")
        # "Create Logged File"
        n1295 = local read "Transaction No"() -> (w2234:string)
        n1296 = property on="Tab Body" class="TabCtl (strict)"() -> ("Pages"=w2230:refnum<vi>[])  [unwired: 2 in, 2 out]
        n1297 = Format Date/Time String(time format string (%c)="%Y%m%d_%H%M%S") -> (date/time string=w2237:string)  [unwired: 2 in]
        n1298 = for {
          tunnel: w2230 -> [w2273] mode=indexing
          tunnel: w2229 -> [w2272] mode=indexing
          n1299 = property class="Page"(reference=w2273, "PageEnb"=w2272) -> ()  [unwired: 1 in, 2 out]
        }
        n1300 = local read "Data_Host"() -> (w2221:path)
        n1301 = Concatenate Strings(w2234, "_" ("string"), w2237, ".dat" ("string")) -> (w2232:string)
        n1302 = property on="Close" class="Bool (strict)"("DisabledEnum"=T27."Disabled and Grayed Out" ("Disabled")) -> ()  [unwired: 2 in, 2 out]
        n1303 = call "Folder - Create Year-Month.vi"("Folder Name"=w2221) -> ("error out"=w2220:errorcluster, "Folder with Year\\Month"=w2219:path)  [unwired: 9 in]
        n1304 = local write "Recipe Start Flag"(FALSE ("Recipe Start Flag")) -> ()
        n1305 = local write "Tab Body"(T1."Execute" ("Tab Body")) -> ()
        n1306 = Build Path(base path=w2219, name or relative path=w2232) -> (appended path=w2244:path)
        "Data File" <- w2244
        n1307 = Path To String(path=w2244) -> (string=w2243:string)
        n1308 = flat-sequence "EXECUTE TAB" {
          frame #0 {
            w2264 = timestamp(3471350400 s since 1904-01-01) ("Parameter (Start Dwell Time)")
            # "Clear Data on EXECUTE TAB"
            n1309 = local write "Parameter (Start Dwell Time)"(w2264) -> ()
            n1310 = local write "Parameter (End Dwell Time)"(w2264) -> ()
            n1311 = property on="% Hold. Time Completed" class="Slide (strict)"("Scale.Maximum"=100.0 ("Scale.Range:Maximum"), "Scale.Minimum"=0.0 ("Scale.Range:Minimum"), "Fill Color"=u32 16777216 ("Color Box 2"), "Value"=0.0 ("% Hold Time Completed")) -> ()  [unwired: 2 in, 2 out]
            n1312 = property on="Variant Allowed" class="Bool (strict)"("Colors [4]"=cluster{"Color Box":u32, "Color Box 2":u32}[] [{"Color Box"=16711680, "Color Box 2"=16711680}, {"Color Box"=9868950, "Color Box 2"=9868950}, {"Color Box"=4934475, "Color Box 2"=4934475}, {"Color Box"=6618880, "Color Box 2"=6618880}], "Value"=TRUE) -> ()  [unwired: 2 in, 2 out]
            n1313 = property on="Hold. Time (hour:minute)" class="Str"() -> ("Value"=w2257:string)  [unwired: 2 in, 2 out]
            n1314 = call "String - Format to (HH_colon_MM).vi"("xx:xx"=w2257) -> ("seconds"=w2255:dbl)  [unwired: 9 in, 1 out]
            n1315 = disable-structure shown="Disabled" {
              frame Disabled {
                # "Will be updated below"
                n1316 = local write "Raw Data File"("") -> ()
              }
              frame Enabled {
              }
            }
            n1317 = flat-sequence {
              frame #0 {
                w2268 = 12  # 12 Probes Max
                n1318 = property on="Chart" class="WFChart (strict)"("History Data"=dynamicdata[] []) -> ()  [unwired: 2 in, 2 out]
                n1319 = for {
                  N: w2268 -> [_]
                  i -> [w2270]
                  n1320 = property on="Chart" class="WFChart (strict)"("Active Plot"=w2270, "Plot.Plot Name"="") -> ()  [unwired: 2 in, 2 out]
                }
              }
            }
            n1321 = property on="Recording Duration" class="DigNum (strict)"("Value"=0.0) -> ()  [unwired: 2 in, 2 out]
            n1322 = property on="Remaining Hold Time" class="DigNum (strict)"("Value"=w2255) -> ()  [unwired: 2 in, 2 out]
            n1323 = property on="Recipe Stop" class="Bool"("DisabledEnum"=T27."Enabled" ("Disabled")) -> ()  [unwired: 2 in, 2 out]
            n1324 = property on="Recipe Start" class="Bool"("DisabledEnum"=T27."Disabled and Grayed Out" ("Disabled")) -> ()  [unwired: 2 in, 2 out]
            n1325 = local write "Process Completed"(FALSE ("Overall Status")) -> ()
            n1326 = local write "Hold Time Completed"(FALSE ("Hold Time Completed")) -> ()
          }
        }
        n1327 = local read "Probe List"() -> (w2227:i32[])
        n1328 = Concatenate Strings(w2242, w2243, w2242, " Raw Data File Created." ("string")) -> (w2240:string)
        n1329 = Open/Create/Replace File(file path (use dialog)=w2244, error in=w2220, operation (0:open)=T28."replace or create") -> (refnum out=w2248:refnum<file>, error out=w2246:errorcluster)  [unwired: 3 in, 1 out]
        n1330 = Array To Spreadsheet String(delimiter (Tab)=",", array=w2227, 3:"%d" ("format string")) -> (spreadsheet string=w2223:string)
        n1331 = Concatenate Strings("Time," ("string"), w2223) -> (w2222:string)
        n1332 = Enqueue Element(queue=w2245, element=w2240, timeout in ms (-1)=w2239) -> ()  [unwired: 1 in, 3 out]
        n1333 = Write to Text File(file (use dialog)=w2248, text=w2222, error in=w2246) -> (refnum out=→"Logged File Ref":refnum<file>, error out=w2233:errorcluster)  [unwired: 1 in, 1 out]
        "Data File Error" <- w2233
        n1334 = case shown="No Error" w2233 {
          tunnel: w2232 -> [w2274 _]
          frame No Error {
            # "Display on Front Panel"
            n1335 = local write "Raw Data File"(w2274) -> ()
          }
          frame Error {
          }
        }
      }
      frame "START Recovery" {
        # "Starts Process1"
        n1336 = Tick Count (ms)() -> (millisecond timer value=→"Start Cycle":u32)
        n1337 = Index Array(array=w2275, index=w2282) -> (element=w2281:string)
        n1338 = Concatenate Strings("Cycle Started. ", "Cycle Number =  ", w2281, "." ("string")) -> (w2278:string)
        n1339 = Enqueue Element(queue=w2284, element=w2278, timeout in ms (-1)=w2277) -> ()  [unwired: 1 in, 3 out]
      }
      frame "BEGIN Process" {
        # "Begin Process 1"
        n1340 = local read "cRIO DAQ Start"() -> (w2287:bool)
        n1341 = case shown="False" w2287 {
          tunnel: [w2304 _] -> w2290
          frame False {
            w2312 = TRUE  # DAQ Start
            # "Not Started Yet"
            n1342 = local read "Simulate cRIO"() -> (w2305:bool)
            n1343 = local read "cRIO shared variable RT Library"() -> (w2308:string)
            n1344 = local read "cRIO Folder"() -> (w2311:string)
            n1345 = local read "Transaction No"() -> (w2310:string)
            n1346 = local read "Probe List"() -> (w2307:i32[])
            n1347 = local read "cRIO Channel List"() -> (w2306:i32[])
            n1348 = control-ref of="cRIO Status"() -> (w2303:refnum<vi>)
            n1349 = call "cRIO - Shared Variable RW.vi"("shared variable RT Library"=w2308, "Read/Write"=enum16{"Write", "Read"}."Write", "Data Path Name"=w2311, "cRIO Channel List (In)"=w2310, "Simulate cRIO"=w2305, "Probe List In"=w2307, "DAQ Start"=w2312, "File IO Status"=w2306, "cRIO Status"=w2303) -> ("Error Out"=w2304:errorcluster)  [unwired: 3 in, 7 out]
          }
          frame True {
            # "Already Started in \"Ready to Start\" \ni.e. PC crashed in previous run\nSo no need to resend DAQ Start"
          }
        }
        n1350 = local read "Simulate ET3500"() -> (w2294:bool)
        n1351 = local read "VISA resource name RS232"() -> (w2296:string)
        n1352 = Enqueue Element(queue=w2301, element="Process 1 Started. ", timeout in ms (-1)=w2299) -> ()  [unwired: 1 in, 3 out]
        n1353 = control-ref of="ET3504 Status"() -> (w2286:refnum<vi>)
        n1354 = call "ET3500 - Read Program Parameters.vi"("Simulate"=w2294, "ET3500 Status"=w2286, "subVI (Auto Interactive)"=TRUE ("subVI"), "Option"=cluster{"Init":bool, "Close":bool} {"Init"=TRUE, "Close"=FALSE}, "VISA resource name"=w2296) -> ("error out"=w2292:errorcluster, "Parameter Cluster (Scaled)"=w2288:T36)  [unwired: 2 in, 3 out]
        n1355 = Unbundle By Name(w2288) -> ("PVIn (degC)"=w2289:dbl)
        n1356 = local write "Parameter Cluster (Scaled)"(w2288) -> ()
        n1357 = local write "cRIO Error"(w2290) -> ()
        n1358 = local write "ET3500 Error"(w2292) -> ()
        n1359 = property on="Current Temp" class="DigNum (strict)"("Value"=w2289) -> ()  [unwired: 2 in, 2 out]
        n1360 = Merge Errors(w2292, w2290) -> (w2291:errorcluster)
        n1361 = flat-sequence {
          frame #0 {
            n1362 = Wait Until Next ms Multiple(millisecond multiple=u32 200) -> ()  [unwired: 1 out]
          }
          frame #1 {
            n1363 = Tick Count (ms)() -> (millisecond timer value=→"Process 1 t0":u32)
          }
        }
      }
      frame "RUNNING Process" {
        n1364 = local read "Host Sampling Interval (s)"() -> (w2322:dbl)
        n1365 = local read "Process 1 t0"() -> (w2339:u32)
        n1366 = call "Elapsed Time"("Time Target (s)"=w2322) -> ("Elapsed Time (s)"=w2335:dbl, "Time has Elapsed"=w2332:bool)  [unwired: 11 in, 6 out]
        "Time has Elapsed" <- w2332
        n1367 = Tick Count (ms)() -> (millisecond timer value=w2337:u32)
        n1368 = Equal To 0?(x=w2318) -> (x = 0?=w2328:bool)
        n1369 = Subtract(x=w2337, y=w2339) -> (x-y=w2336:u32)
        n1370 = Subtract(x=w2322, y=w2335) -> (x-y=w2334:dbl)
        n1371 = Or(x=w2332, y=w2328) -> (x .or. y?=w2319:bool)
        n1372 = Max & Min(x=0.0, y=w2334) -> (max(x,y)=→"Time to next sample (s)":dbl)  [unwired: 1 out]
        n1373 = Divide(x=w2336, y=u32 1000) -> (x/y=w2331:dbl)
        n1374 = case shown="True" w2319 {
          tunnel: w2331 -> [_ w2498]
          tunnel: [_ w2478] -> w2325
          tunnel: w2318 -> [w2465 w2469]
          tunnel: [w2465 w2468] -> w2333
          tunnel: [_ w2484] -> w2323
          tunnel: w2316 -> [_ w2477]
          tunnel: w2315 -> [_ w2475]
          frame False {
            # "Not Time Yet => SKIP Logging Of Data"
          }
          frame True {
            w2504 = "," ("delimiter (Tab)")
            (unwired) "%.1f" ("format string")
            # "New Data\nDelimiter is ,"
            n1375 = local read "cRIO shared variable RT Library"() -> (w2492:string)
            n1376 = local read "cRIO Error"() -> (w2494:errorcluster)
            n1377 = local read "Simulate cRIO"() -> (w2493:bool)
            n1378 = control-ref of="cRIO Status"() -> (w2466:refnum<vi>)
            n1379 = call "cRIO - Shared Variable RW.vi"("shared variable RT Library"=w2492, "Read/Write"=enum16{"Write", "Read"}."Read", "Error In"=w2494, "Simulate cRIO"=w2493, "cRIO Status"=w2466) -> ("Probe List Out"=w2497:i32[], "data out"=w2471:dbl[], "cRIO Timestamp"=w2488:timestamp, "Cycle Count"=w2499:i32, "DAQ Started"=w2495:bool, "Error Out"=w2485:errorcluster)  [unwired: 6 in, 3 out]
            n1380 = Number To Decimal String(number=w2497) -> (decimal integer string=w2496:string[])  [unwired: 1 in]
            n1381 = local write "cRIO Timestamp (only updated when a Shared Variable is Read)"(w2488) -> ()
            n1382 = for {
              tunnel: w2496 -> [w2516] mode=indexing
              i -> [w2517]
              n1383 = property on="Chart" class="WFChart (strict)"("Active Plot"=w2517, "Plot.Plot Name"=w2516) -> ()  [unwired: 2 in, 2 out]
            }
            n1384 = local write "cRIO Cycle Count"(w2499) -> ()
            n1385 = local write "cRIO DAQ Start"(w2495) -> ()
            n1386 = Add(x=0.0, y=w2498) -> (x+y=w2491:dbl)
            n1387 = Divide(x=w2491, y=60.0) -> (x/y=w2489:dbl)
            n1388 = Select(t=errorcluster {"status"=TRUE, "code"=-1000, "source"="Simulate cRIO Comm Error. "} ("Error Out"), s="Simulate cRIO Comm Error", f=w2485) -> (s? t:f=w2484:errorcluster)
            n1389 = Select(t=dbl[] [], s="Simulate cRIO No Data", f=w2471) -> (s? t:f=w2470:dbl[])
            n1390 = Array Size(array=w2470) -> (size(s)=w2483:i32)
            n1391 = Number To Fractional String(number=w2489, precision (6)=i16 1) -> (F-format string=w2503:string)  [unwired: 2 in]
            n1392 = local write "cRIO Error"(w2484) -> ()
            n1393 = call "Convert to Dynamic Data"("Array"=w2470) -> ("Dynamic Data Type"=→"Chart":dynamicdata)  [unwired: 3 in]
            n1394 = Array To Spreadsheet String(delimiter (Tab)=w2504, array=w2470, 3:"%#_4" ("format string")) -> (spreadsheet string=w2505:string)
            n1395 = Greater Than 0?(x=w2483) -> (x > 0?=w2476:bool)
            n1396 = Concatenate Strings(w2503, w2504, w2505) -> (w2480:string)
            n1397 = local read "Logged File Ref"() -> (w2506:refnum<file>)
            n1398 = Concatenate Strings(w2480, "\r\n" ("string")) -> (w2482:string)
            n1399 = Select(t=w2480, s=w2476, f=w2482) -> (s? t:f=w2479:string)
            n1400 = case shown="True" w2476 {
              tunnel: w2477 -> [w2513 _]
              tunnel: w2475 -> [w2512 _]
              tunnel: w2469 -> [w2511 w2515]
              tunnel: [w2511 w2514] -> w2468
              frame False {
                # "Array = 0, cRIO No data"
                n1401 = Number To Decimal String(number=w2511) -> (decimal integer string=w2509:string)  [unwired: 1 in]
                n1402 = Concatenate Strings("cRIO No Data. Current Samples/ch Count = " ("element"), w2509, ". " ("string")) -> (w2508:string)
                n1403 = Enqueue Element(queue=w2513, element=w2508, timeout in ms (-1)=w2512) -> ()  [unwired: 1 in, 3 out]
              }
              frame True {
                # "Array >0 , cRIO Data OK"
                n1404 = Increment(x=w2515) -> (x+1=w2514:i32)
              }
            }
            n1405 = Write to Text File(file (use dialog)=w2506, text=w2479) -> (error out=w2478:errorcluster)  [unwired: 2 in, 2 out]
            n1406 = local write "Data File Error"(w2478) -> ()
          }
        }
        "Samples/ch Count" <- w2333
        n1407 = case shown="True" w2319 {
          tunnel: w2331 -> [w2344 w2360]
          tunnel: w2330 -> [w2348 w2369]
          tunnel: [w2348 w2367] -> w2329
          tunnel: [_ w2361] -> w2317
          tunnel: [w2347 w2351] -> w2327
          tunnel: w2326 -> [w2347 w2365]
          tunnel: [_ w2353] -> w2321
          tunnel: w2318 -> [_ w2357]
          frame False {
            n1408 = local read "Key Values"() -> (w2346:T9)
            n1409 = Bundle By Name(cluster=w2346, "Recording Duration"=w2344) -> (w2345:T9)
            n1410 = local write "Key Values"(w2345) -> ()
          }
          frame True {
            # "Time Elapsed"
            n1411 = local read "ET3500 Error"() -> (w2363:errorcluster)
            n1412 = local read "VISA resource name RS232"() -> (w2364:string)
            n1413 = local read "Simulate ET3500"() -> (w2362:bool)
            n1414 = control-ref of="ET3504 Status"() -> (w2350:refnum<vi>)
            n1415 = call "ET3500 - Read Program Parameters.vi"("Sample/ch per Count"=w2357, "Simulate"=w2362, "ET3500 Status"=w2350, "error in (no error)"=w2363, "subVI (Auto Interactive)"=TRUE ("subVI"), "Option"=cluster{"Init":bool, "Close":bool} {"Init"=FALSE, "Close"=FALSE}, "VISA resource name"=w2364) -> ("error out"=w2354:errorcluster, "Segment.Type"=w2351:i16, "Parameter Cluster (Scaled)"=w2372:T36, "Segment.Duration (min)"=w2366:dbl)  [unwired: 1 out]
            "Parameter Cluster (Scaled)" <- w2372
            n1416 = Unbundle By Name(w2372) -> ("SegTimeLeft (min)"=w2371:dbl, "PVIn (degC)"=w2349:dbl, "ProgStatus"=w2370:i16)
            n1417 = Select(t=errorcluster {"status"=TRUE, "code"=-1000, "source"="Simulate ET3500 Error. "} ("Error Out"), s="Simulate ET3500 Error", f=w2354) -> (s? t:f=w2353:errorcluster)
            n1418 = local write "ET3500 Error"(w2353) -> ()
            n1419 = To Long Integer(number=w2370) -> (32bit integer=w2368:i32)
            n1420 = case shown="3" w2351 {
              tunnel: [w2408 w2443] -> w2358
              tunnel: w2371 -> [_ w2445]
              tunnel: w2366 -> [_ w2448]
              tunnel: w2365 -> [w2404 w2433]
              tunnel: w2349 -> [w2409 w2438]
              frame 0, Default {
                # "End (0) or Rate (1)"
                n1421 = local read "Parameter (End Dwell Time)"() -> (w2407:timestamp)
                n1422 = case shown="3" w2404 {
                  tunnel: w2409 -> [_ w2429]
                  frame 0, Default {
                  }
                  frame 3 {
                    # "Previous State is Dwell (3)"
                    n1423 = property on="% Hold. Time Completed" class="Slide (strict)"() -> ("Scale.Maximum"=w2431:dbl)  [unwired: 2 in, 2 out]
                    n1424 = Get Date/Time In Seconds() -> (seconds since 1Jan1904=w2430:timestamp)
                    "Parameter (End Dwell Time)" <- w2430
                    n1425 = call "Parameters - Update.vi"("Parameter (End Dwell Temp)"=w2429, "Parameter (End Dwell Time)"=w2430) -> ("Cluster"=w2428:T37)  [unwired: 6 in, 3 out]
                    n1426 = Unbundle By Name(w2428) -> ("End Holding Time & Date"=w2420:string, "End Holding Temperature"=w2419:string)
                    n1427 = local write "% Hold. Time Completed"(w2431) -> ()
                    n1428 = local write "Hold Time Completed"(TRUE ("Hold Time Completed")) -> ()
                    n1429 = local read "Latest stp file"() -> (w2422:path)
                    n1430 = property on="End Holding Time and Date" class="Str"("Value"=w2420) -> (error out=w2418:errorcluster)  [unwired: 2 in, 1 out]
                    n1431 = property on="End Holding Temperature" class="Str"("Value"=w2419) -> (error out=w2417:errorcluster)  [unwired: 2 in, 1 out]
                    n1432 = Merge Errors(w2418, w2417) -> (w2416:errorcluster)
                    n1433 = control-ref of="Parameter Buffer"() -> (w2421:refnum<vi>)
                    n1434 = call <vilib>:"Open Config Data.vi"("error in (no error)"=w2416, "create file if necessary (T)"=FALSE, "configuration file path"=w2422) -> ("error out"=w2425:errorcluster, "refnum"=w2423:T33)  [unwired: 6 in, 1 out]
                    n1435 = call "Key - Cluster Write.vi"("error in (no error)"=w2425, "Cluster Ref in"=w2421, "Refnum in"=w2423) -> ("error out"=w2426:errorcluster, "Refnum out"=w2424:T33)  [unwired: 7 in]
                    n1436 = call <vilib>:"Close Config Data.vi"("error in (no error)"=w2426, "write file if changed (T)"=TRUE, "refnum"=w2424) -> ("error out"=w2415:errorcluster)  [unwired: 7 in, 1 out]
                    n1437 = local write "stp file Error Out"(w2415) -> ()
                  }
                }
                n1438 = Equal?(x=w2407, y=timestamp(3471350400 s since 1904-01-01)) -> (x = y?=w2405:bool)
                n1439 = case shown="True" w2405 {
                  tunnel: [0.0 ("(HH:mm)") w2411] -> w2408
                  frame False {
                    # "Started and Ended"
                  }
                  frame True {
                    # "Not Started Yet"
                    n1440 = local read "Info."() -> (w2413:T8)
                    n1441 = Unbundle By Name(w2413) -> ("Hold. Time (hour:minute)"=w2412:string)
                    n1442 = call "String - Format to (HH_colon_MM).vi"("xx:xx"=w2412) -> ("seconds"=w2411:dbl)  [unwired: 9 in, 1 out]
                  }
                }
              }
              frame 3 {
                w2444 = 60.0  # 60sec
                # "Dwell (3)"
                n1443 = local read "Info."() -> (w2441:T8)
                n1444 = Unbundle By Name(w2441) -> ("Hold. Temp."=w2440:string)
                n1445 = case shown="1" w2433 {
                  tunnel: w2438 -> [_ w2463]
                  frame 0, Default {
                    # "Dwelling"
                  }
                  frame 1 {
                    # "Previous State is Rate (1) => Just Entering Dwell"
                    n1446 = Get Date/Time In Seconds() -> (seconds since 1Jan1904=w2464:timestamp)
                    "Parameter (Start Dwell Time)" <- w2464
                    n1447 = call "Parameters - Update.vi"("Parameter (Start Dwell Temp)"=w2463, "Parameter (Start Dwell Time)"=w2464) -> ("Cluster"=w2462:T37)  [unwired: 6 in, 3 out]
                    n1448 = Unbundle By Name(w2462) -> ("Start Holding Time & Date"=w2454:string, "Start Holding Temperature"=w2453:string)
                    n1449 = property on="Start Holding Temperature" class="Str"("Value"=w2453) -> (error out=w2451:errorcluster)  [unwired: 2 in, 1 out]
                    n1450 = property on="Start Holding Time and Date" class="Str"("Value"=w2454) -> (error out=w2452:errorcluster)  [unwired: 2 in, 1 out]
                    n1451 = local read "Latest stp file"() -> (w2456:path)
                    n1452 = Merge Errors(w2452, w2451) -> (w2450:errorcluster)
                    n1453 = control-ref of="Parameter Buffer"() -> (w2455:refnum<vi>)
                    n1454 = call <vilib>:"Open Config Data.vi"("error in (no error)"=w2450, "create file if necessary (T)"=FALSE, "configuration file path"=w2456) -> ("error out"=w2459:errorcluster, "refnum"=w2457:T33)  [unwired: 6 in, 1 out]
                    n1455 = call "Key - Cluster Write.vi"("error in (no error)"=w2459, "Cluster Ref in"=w2455, "Refnum in"=w2457) -> ("error out"=w2460:errorcluster, "Refnum out"=w2458:T33)  [unwired: 7 in]
                    n1456 = call <vilib>:"Close Config Data.vi"("error in (no error)"=w2460, "refnum"=w2458) -> ("error out"=→"stp file Error Out":errorcluster)  [unwired: 8 in, 1 out]
                  }
                }
                n1457 = property on="% Hold. Time Completed" class="Slide (strict)"("Scale.Maximum"=w2448, "Fill Color"=u32 65421) -> ()  [unwired: 2 in, 2 out]
                n1458 = Fract/Exp String To Number(string=w2440) -> (number=w2439:dbl)  [unwired: 3 in, 1 out]
                n1459 = Subtract(x=w2448, y=w2445) -> (x-y=w2446:dbl)
                n1460 = Equal To 0?(x=w2445) -> (x = 0?=w2447:bool)
                n1461 = call "Parameters - Update.vi"("Parameter (End Dwell Temp)"=w2438, "Parameter (Start Dwell Temp)"=w2439, "Info."=w2441) -> ("Variant Allowed (Current Hold Temp)"=w2435:bool)  [unwired: 5 in, 3 out]
                n1462 = local write "% Hold. Time Completed"(w2446) -> ()
                n1463 = local write "Hold Time Completed"(w2447) -> ()
                n1464 = property on="Variant Allowed" class="Bool (strict)"() -> ("Value"=w2436:bool)  [unwired: 2 in, 2 out]
                n1465 = And(x=w2436, y=w2435) -> (x .and. y?=w2434:bool)
                n1466 = property on="Variant Allowed" class="Bool (strict)"("Colors [4]"=cluster{"Color Box":u32, "Color Box 2":u32}[] [{"Color Box"=16711680, "Color Box 2"=16711680}, {"Color Box"=6618880, "Color Box 2"=6618880}, {"Color Box"=4934475, "Color Box 2"=4934475}, {"Color Box"=6618880, "Color Box 2"=6618880}], "Value"=w2434) -> ()  [unwired: 2 in, 2 out]
                n1467 = Multiply(x=w2444, y=w2445) -> (x*y=w2443:dbl)
              }
            }
            n1468 = case shown="\"Running\"" w2369 {
              selector: w2369 -> [w2375 w2384 w2403]
              tunnel: w2368 -> [w2379 w2387 _]
              tunnel: [w2376 w2385 w2403] -> w2367
              tunnel: [_ _ TRUE] -> w2361
              tunnel: w2349 -> [_ w2383 _]
              frame "Wait For RUN", Default {
                n1469 = Equal?(x=w2379, y=2) -> (x = y?=w2377:bool)
                n1470 = case shown="True" w2377 {
                  tunnel: [w2380 ET3500_Program_Status."Running"] -> w2376
                  tunnel: w2375 -> [w2380 _]
                  frame False {
                  }
                  frame True {
                  }
                }
              }
              frame "Running" {
                # "Wait For Stop"
                n1471 = case shown="True" "Stop On Final Target Temperature" {
                  tunnel: w2387 -> [w2390 _]
                  tunnel: [w2388 w2396] -> w2386
                  tunnel: w2383 -> [_ w2399]
                  frame False {
                    n1472 = Equal?(x=w2390, y=1) -> (x = y?=w2388:bool)
                  }
                  frame True {
                    n1473 = local read "Final Target Temperature"() -> (w2393:cluster{"Final Target Temperature":string})
                    n1474 = Unbundle By Name(w2393) -> ("Final Target Temperature"=w2392:string)
                    n1475 = local read "Hold Time Completed"() -> (w2397:bool)
                    n1476 = Decimal String To Number(string=w2392) -> (number=w2391:i32)  [unwired: 2 in, 1 out]
                    n1477 = Add(x=w2391, y="Final Target Temp Offset") -> (x+y=w2395:i32)
                    "Final Target + Offset\n(Updated Only when active)" <- w2395
                    n1478 = Less Or Equal?(x=w2399, y=w2395) -> (x <= y?=w2398:bool)
                    n1479 = And(x=w2398, y=w2397) -> (x .and. y?=w2396:bool)
                  }
                }
                n1480 = case shown="True" w2386 {
                  tunnel: [w2400 ET3500_Program_Status."Stopped"] -> w2385
                  tunnel: w2384 -> [w2400 _]
                  frame False {
                    # "Keep Waiting"
                  }
                  frame True {
                    # "Stopped"
                  }
                }
              }
              frame "Stopped" {
              }
            }
            n1481 = local write "Process Completed"(w2361) -> ()
            n1482 = local read "Key Values"() -> (w2359:T9)
            n1483 = Bundle By Name(cluster=w2359, "Recording Duration"=w2360, "Remaining Hold Time"=w2358, "Current Temp"=w2349) -> (w2352:T9)
            n1484 = local write "Key Values"(w2352) -> ()
          }
        }
        n1485 = case shown="True" w2317 {
          tunnel: [w2519 Enum_-_SRTRS_State."END Process" ("Enum")] -> w2343
          tunnel: w2342 -> [w2519 _]
          frame False {
            # "Keep Checking"
            n1486 = Wait Until Next ms Multiple(millisecond multiple=u32 10) -> ()  [unwired: 1 out]
          }
          frame True {
            # "Goto Next Process"
          }
        }
        n1487 = Merge Errors(w2325, w2323, w2321) -> (w2324:errorcluster)
      }
      frame "END Process" {
        n1488 = local read "Simulate ET3500"() -> (w2525:bool)
        n1489 = local read "VISA resource name RS232"() -> (w2527:string)
        n1490 = control-ref of="ET3504 Status"() -> (w2521:refnum<vi>)
        n1491 = call "ET3500 - Read Program Parameters.vi"("Simulate"=w2525, "ET3500 Status"=w2521, "subVI (Auto Interactive)"=TRUE ("subVI"), "Option"=cluster{"Init":bool, "Close":bool} {"Init"=FALSE, "Close"=TRUE}, "VISA resource name"=w2527) -> ("error out"=w2523:errorcluster, "Parameter Cluster (Scaled)"=w2522:T36)  [unwired: 2 in, 3 out]
        n1492 = local write "Parameter Cluster (Scaled)"(w2522) -> ()
        n1493 = local write "ET3500 Error"(w2523) -> ()
      }
      frame "Spare Enum" {
        # "Begin Process 2"
        n1494 = Tick Count (ms)() -> (millisecond timer value=→"Process 2 t0":u32)
        n1495 = Enqueue Element(queue=w2535, element="Process 2 Started. ", timeout in ms (-1)=w2533) -> ()  [unwired: 1 in, 3 out]
      }
      frame "END Recipe" {
      }
      frame "ERROR Handling" {
        # "Check if Recipe has ended"
        n1496 = Increment "Goto Next INDEX"(x=w2547) -> (x+1=w2544:i32)
        n1497 = Index Array(array=w2542, index=w2547) -> (element=w2546:string)
        n1498 = Equal?(x=1, y=w2544) -> (x = y?=w2554:bool)
        n1499 = Select(t=Enum_-_SRTRS_State."END Recipe" ("Enum"), s=w2554, f=Enum_-_SRTRS_State."START Recovery" ("Enum")) -> (s? t:f=w2555:T16)
        n1500 = Concatenate Strings("Cycle Ended. ", "Cycle Number = ", w2546, "." ("string")) -> (w2548:string)
        n1501 = Enqueue Element(queue=w2553, element=w2548, timeout in ms (-1)=w2552) -> ()  [unwired: 1 in, 3 out]
      }
      frame "END Recipe" {
        w2561 = T23 [enum."Page Enabled", enum."Page Enabled", enum."Page Enabled", enum."Page Enabled", enum."Page Enabled"] items=["Page Enabled", "Page Disabled", "Page Disabled & Grayed"]
        w2568 = 0  # Reset Cycle Count
        n1502 = local read "Logged File Ref"() -> (w2575:refnum<file>)
        n1503 = property on="Tab Body" class="TabCtl (strict)"() -> ("Pages"=w2562:refnum<vi>[])  [unwired: 2 in, 2 out]
        n1504 = Close File(refnum=w2575) -> (error out=w2560:errorcluster)  [unwired: 1 in, 1 out]
        n1505 = case shown="True" "Report.Create.Excel" {
          tunnel: w2560 -> [w2617 _]
          tunnel: [w2617 w2618] -> w2574
          frame False {
          }
          frame True {
            n1506 = local read "Data File"() -> (w2620:path)
            n1507 = property on="Report Generate" class="Bool (strict)"("Val(Sgnl)"=TRUE) -> (error out=w2618:errorcluster)  [unwired: 2 in, 1 out]
            n1508 = local write "Raw Data File"(w2620) -> ()
          }
        }
        n1509 = for {
          tunnel: w2562 -> [w2602] mode=indexing
          tunnel: w2561 -> [w2601] mode=indexing
          n1510 = property class="Page"(reference=w2602, "PageEnb"=w2601) -> ()  [unwired: 1 in, 2 out]
        }
        n1511 = flat-sequence {
          tunnel: w2560 -> [_]
          frame #0 {
            n1512 = local read "Data File"() -> (w2580:path)
            n1513 = Strip Path(path=w2580) -> (stripped path=w2593:path, name=w2582:string)
            n1514 = Strip Path(path=w2593) -> (stripped path=w2592:path, name=w2590:string)
            n1515 = Strip Path(path=w2592) -> (name=w2591:string)  [unwired: 1 out]
            n1516 = local read "Data"() -> (w2589:path)
            n1517 = Concatenate Strings(w2591, "\\" ("string"), w2590) -> (w2588:string)
            n1518 = Build Path(base path=w2589, name or relative path=w2588) -> (appended path=w2583:path)
            n1519 = Build Path(base path=w2583, name or relative path=w2582) -> (appended path=w2579:path)
            n1520 = call <vilib>:"Check if File or Folder Exists.vi"("path"=w2583) -> ("error out"=w2584:errorcluster, "file or folder exists?"=w2586:bool, "dup path"=w2585:path)  [unwired: 8 in]
            n1521 = case shown="False" w2586 {
              tunnel: w2585 -> [w2598 w2600]
              tunnel: [w2597 w2600] -> _
              tunnel: [w2596 w2599] -> w2581
              tunnel: w2584 -> [w2595 w2599]
              frame False {
                # "Create Folder if NOT found\nCreate NEW"
                n1522 = Create Folder(path (use dialog)=w2598, error in=w2595) -> (created path=w2597:path, error out=w2596:errorcluster)  [unwired: 1 in, 1 out]
              }
              frame True {
                # "Folder Found"
              }
            }
            n1523 = Copy(8:w2581, 10:w2579, 11:w2580) -> (0:w2578:errorcluster)  [unwired: 2 in, 2 out]
            n1524 = local write "Data File Error"(w2578) -> ()
            n1525 = case shown="Error" w2578 {
              frame No Error {
              }
              frame Error {
                n1526 = One Button Dialog(message=".dat File copy failed.") -> ()  [unwired: 1 in, 1 out]
              }
            }
          }
        }
        n1527 = local read "cRIO shared variable RT Library"() -> (w2558:string)
        n1528 = property on="Recipe Stop" class="Bool"("DisabledEnum"=T27."Disabled and Grayed Out" ("Disabled")) -> ()  [unwired: 2 in, 2 out]
        n1529 = local read "Simulate cRIO"() -> (w2563:bool)
        n1530 = control-ref of="cRIO Status"() -> (w2559:refnum<vi>)
        n1531 = local write "Recipe Stop Flag"(FALSE ("Recipe Stop Flag")) -> ()
        n1532 = call "cRIO - Shared Variable RW.vi"("shared variable RT Library"=w2558, "Read/Write"=enum16{"Write", "Read"}."Write", "Simulate cRIO"=w2563, "DAQ Start"=FALSE, "cRIO Status"=w2559) -> ("Error Out"=w2564:errorcluster)  [unwired: 6 in, 8 out]
        n1533 = while {
          tunnel: w2564 -> [w2616]
          tunnel: w2563 -> [w2615]
          tunnel: w2559 -> [w2604]
          tunnel: w2558 -> [w2603]
          i -> [w2610]
          stop <- w2612 stop-if-true
          # "Check for cRIO DAQ Stop"
          n1534 = Wait Until Next ms Multiple(millisecond multiple=u32 100) -> ()  [unwired: 1 out]
          n1535 = call "cRIO - Shared Variable RW.vi"("shared variable RT Library"=w2603, "Read/Write"=enum16{"Write", "Read"}."Read", "Error In"=w2616, "Simulate cRIO"=w2615, "cRIO Status"=w2604) -> ("Cycle Count"=w2613:i32, "DAQ Started"=w2606:bool, "Error Out"=w2605:errorcluster)  [unwired: 6 in, 6 out]
          n1536 = local write "cRIO Cycle Count"(w2613) -> ()
          n1537 = local write "cRIO DAQ Start"(w2606) -> ()
          n1538 = Not(x=w2606) -> (.not. x?=w2611:bool)
          n1539 = Greater Or Equal?(x=w2610, y=50) -> (x >= y?=w2608:bool)
          n1540 = local write "cRIO Error"(w2605) -> ()
          n1541 = Compound Arithmetic op=OR(w2608, w2611, w2605) -> (w2612:bool)
        }
        n1542 = Enqueue Element(queue=w2571, element="Recipe Ended.", timeout in ms (-1)=w2569) -> ()  [unwired: 1 in, 3 out]
        n1543 = Merge Errors(w2574, w2560) -> (w2572:errorcluster)
      }
      frame "ERROR Handling" {
        # "Clear Error, STOP Processes"
        n1544 = Unbundle By Name(w2626) -> ("code"=w2632:i32, "source"=w2634:string)
        n1545 = flat-sequence {
          frame #0 {
            # "STOP cRIO"
          }
        }
        n1546 = case shown="0, Default" w2632 {
          tunnel: [w2637 _] -> w2631
          tunnel: [_ w2677] -> w2630
          tunnel: [w2642 w2676] -> w2629
          tunnel: w2626 -> [w2643 _]
          tunnel: w2625 -> [w2639 _]
          frame 0, Default {
            # "Normal Error, \nNot Serious, we clear error and go back to READY TO START"
            n1547 = local read "Show LabVIEW Error"() -> (w2640:bool)
            n1548 = local read "ET3500 Error"() -> (w2646:errorcluster)
            n1549 = local read "cRIO Error"() -> (w2645:errorcluster)
            n1550 = Merge Errors(w2646, w2645) -> (w2644:errorcluster)
            n1551 = disable-structure shown="Disabled" {
              frame Disabled {
                w2657 = T23 [enum."Page Enabled", enum."Page Enabled", enum."Page Enabled", enum."Page Enabled", enum."Page Enabled"] items=["Page Enabled", "Page Disabled", "Page Disabled & Grayed"]
                n1552 = property on="Tab Body" class="TabCtl (strict)"() -> ("Pages"=w2658:refnum<vi>[])  [unwired: 2 in, 2 out]
                n1553 = for {
                  tunnel: w2658 -> [w2660] mode=indexing
                  tunnel: w2657 -> [w2659] mode=indexing
                  n1554 = property class="Page"(reference=w2660, "PageEnb"=w2659) -> ()  [unwired: 1 in, 2 out]
                }
              }
              frame Enabled {
              }
            }
            n1555 = case shown="False" w2640 {
              tunnel: w2643 -> [_ w2656]
              frame False {
              }
              frame True {
                n1556 = call <vilib>:"Simple Error Handler.vi"("error in (no error)"=w2656) -> ()  [unwired: 4 in, 5 out]
              }
            }
            n1557 = case shown="Error" w2645 {
              selector: w2645 -> [_ w2667]
              tunnel: [_ w2664] -> w2641
              frame No Error {
              }
              frame Error {
                n1558 = Unbundle By Name(w2667) -> ("source"=w2665:string)  [unwired: 1 out]
                n1559 = control-ref of="cRIO Status"() -> (w2662:refnum<vi>)
                n1560 = property class="Str"(reference=w2662, "Text.BG Color"=u32 16777216 ("ET3500 Transparent Color"), "Value"="Offline. " ("cRIO Status")) -> ()  [unwired: 1 in, 2 out]
                n1561 = Concatenate Strings("cRIO communication ERROR. \n" ("element"), w2665) -> (w2664:string)
              }
            }
            n1562 = case shown="Error" w2646 {
              selector: w2646 -> [_ w2675]
              tunnel: [_ w2672] -> w2647
              frame No Error {
              }
              frame Error {
                n1563 = Unbundle By Name(w2675) -> ("source"=w2673:string)  [unwired: 1 out]
                n1564 = control-ref of="ET3504 Status"() -> (w2670:refnum<vi>)
                n1565 = property class="Str"(reference=w2670, "Text.BG Color"=u32 16777216 ("ET3500 Transparent Color"), "Value"="Offline." ("ET3500 Program Status")) -> ()  [unwired: 1 in, 2 out]
                n1566 = Concatenate Strings("ET3500 communication ERROR. \n" ("element"), w2673, "\n\n" ("string")) -> (w2672:string)
              }
            }
            n1567 = Concatenate Strings(w2647, w2641) -> (w2642:string)
            n1568 = case shown="\"READY TO START\", Default" w2639 {
              tunnel: w2644 -> [w2652 _]
              tunnel: w2642 -> [w2651 _]
              tunnel: [errorcluster {"status"=FALSE, "code"=0, "source"=""} ("ET3500 Error") _] -> w2638
              tunnel: [Enum_-_SRTRS_State."READY TO START" ("Enum") Enum_-_SRTRS_State."RUNNING Process" ("Enum")] -> w2637
              frame "READY TO START", Default {
                # "Prompt Error"
                n1569 = case shown="Error" w2652 {
                  tunnel: w2651 -> [_ w2654]
                  frame No Error {
                  }
                  frame Error {
                    # "Error Statements"
                    n1570 = One Button Dialog(message=w2654) -> ()  [unwired: 1 in, 1 out]
                    n1571 = local write "Tab Body"(T1."Setup" ("Tab Body")) -> ()
                  }
                }
              }
              frame "RUNNING Process" {
                # "Continue to go back to the same STATE. \nOnly Status will update that there is an ERROR. User can still choose to STOP the Recipe or CLOSE the program."
              }
            }
            n1572 = flat-sequence {
              tunnel: w2638 -> [w2648]
              frame #0 {
                n1573 = local write "ET3500 Error"(w2648) -> ()
                n1574 = local write "cRIO Error"(w2648) -> ()
              }
            }
          }
          frame -88888 {
            w2676 = " QUIT."  # Send to MessageQ
            w2677 = TRUE  # STOP While Loop
            # "Serious Error,  QUIT Now"
          }
        }
        n1575 = flat-sequence {
          frame #0 {
            # "Clear RS232"
          }
        }
        n1576 = Concatenate Strings("Error Handling. [Error] " ("element"), w2634, w2629) -> (w2633:string)
        n1577 = Enqueue Element(queue=w2636, element=w2633, timeout in ms (-1)=w2627) -> (error out=w2628:errorcluster)  [unwired: 1 in, 2 out]
      }
      frame "QUIT" {
        # "Clear All Hardware States"
        n1578 = local read "cRIO DAQ Start"() -> (w2678:bool)
        n1579 = local write "Quit Flag"(FALSE ("Quit Flag")) -> ()
        n1580 = case shown="True" w2678 {
          frame False {
          }
          frame True {
            # "If cRIO DAQ Started already"
            n1581 = local read "cRIO shared variable RT Library"() -> (w2686:string)
            n1582 = local read "Simulate cRIO"() -> (w2689:bool)
            n1583 = control-ref of="cRIO Status"() -> (w2687:refnum<vi>)
            n1584 = call "cRIO - Shared Variable RW.vi"("shared variable RT Library"=w2686, "Read/Write"=enum16{"Write", "Read"}."Write", "Simulate cRIO"=w2689, "DAQ Start"=FALSE, "cRIO Status"=w2687) -> ("Error Out"=w2688:errorcluster)  [unwired: 6 in, 8 out]
            n1585 = local write "cRIO Error"(w2688) -> ()
          }
        }
        n1586 = Enqueue Element(queue=w2682, element="QUIT", timeout in ms (-1)=w2680) -> (error out=w2681:errorcluster)  [unwired: 1 in, 2 out]
      }
    }
    "State Machine Error Out" <- w2105
    n1587 = Format Date/Time String(time format string (%c)="%b %d, %Y  %H:%M:%S") -> (date/time string=→"date/time string":string)  [unwired: 2 in]
    n1588 = case shown="Error" w2105 {
      tunnel: w2110 -> [w2121 _]
      tunnel: [w2116 Enum_-_SRTRS_State."ERROR Handling" ("Enum")] -> w2104
      frame No Error {
        n1589 = local read "Recipe Stop Flag"() -> (w2115:bool)
        n1590 = local read "Quit Flag"() -> (w2114:bool)
        n1591 = Or(x=w2115, y=w2114) -> (x .or. y?=w2120:bool)
        n1592 = Select(t=Enum_-_SRTRS_State."END Recipe" ("Enum"), s=w2115, f=Enum_-_SRTRS_State."QUIT" ("Enum")) -> (s? t:f=w2117:T16)
        n1593 = Select(t=w2117, s=w2120, f=w2121) -> (s? t:f=w2116:T16)
      }
      frame Error {
      }
    }
    "Enum" <- w2100
  }
  n1594 = Close File(refnum=w15, error in=w14) -> (error out=→"Event File Error":errorcluster)  [unwired: 1 out]
  n1595 = disable-structure "Templates" shown="Disabled" {
    frame Disabled {
      n1596 = case shown="Error" {
        selector: _ -> [_ _]
        tunnel: _ -> [w2706 _]
        tunnel: [w2702 w2709] -> _
        tunnel: "[Save WPS]" ("string") -> [w2700 w2708]
        frame No Error {
          w2704 = "\"" ("string")
          # "File Save OK"
          n1597 = Path To String(path=w2706) -> (string=w2705:string)
          n1598 = Concatenate Strings(w2700, " OK." ("string"), "\n") -> (w2699:string)
          n1599 = Concatenate Strings(w2699, w2704, w2705, w2704, " saved. " ("string")) -> (w2702:string)
        }
        frame Error {
          # "File Save Not OK"
          n1600 = Concatenate Strings(w2708, " Cancelled.", "\n") -> (w2709:string)
        }
      }
      n1601 = local read "CellBG Unused Cells"() -> (w2692:u32)
      n1602 = local read "CellBG New Cells"() -> (w2693:u32)
      n1603 = Concatenate Strings("Confirm Delete " ("string")) -> (w2696:string)  [unwired: 1 in]
      n1604 = Two Button Dialog(message=w2696) -> ()  [unwired: 2 in, 1 out]
      n1605 = call "MCListbox Refresh.vi"("Which Cells"=T29."Exisiting and Blank Cells", "color of New Cells"=w2693, "color of Blank cells"=w2692) -> ()  [unwired: 7 in, 2 out]
    }
    frame Enabled {
    }
  }
  n1606 = flat-sequence {
    tunnel: [w2712] -> w22
    tunnel: w21 -> [_]
    frame #0 {
      # "If the Main Loop was not stopped due to user clicking on QUIT button, we need to Create Quit Event to STOP Edit Recipe Event Loop."
      n1607 = property on="Close" class="Bool (strict)"("Val(Sgnl)"=TRUE ("Value (Signaling)")) -> (error out=w2712:errorcluster)  [unwired: 2 in, 1 out]
    }
  }
  n1608 = flat-sequence {
    tunnel: w23 -> [_]
    tunnel: w22 -> [_]
    tunnel: w17 -> [w2715]
    tunnel: [w2713] -> w4
    frame #0 {
      # "MessageQ is the last to release\nMSGBox to release also"
      n1609 = call "Msgbox - Release Q.vi"() -> ()  [unwired: 11 in, 1 out]
      n1610 = local write "Close"(FALSE ("Quit")) -> ()
      n1611 = Release Queue "MessageQ"(queue=w2715) -> (error out=w2713:errorcluster)  [unwired: 2 in, 2 out]
    }
  }
  n1612 = flat-sequence {
    tunnel: w4 -> [_]
    tunnel: w2 -> [_]
    frame #0 {
      n1613 = local read "Application:Name"() -> (w2721:string)
      n1614 = To Upper Case(1:w2721) -> (0:w2720:string)
      n1615 = To Upper Case(1:"LabVIEW.exe" ("regular expression")) -> (0:w2718:string)
      n1616 = Match Pattern(string=w2720, regular expression=w2718) -> (offset past match=w2717:i32)  [unwired: 1 in, 3 out]
      n1617 = Greater Or Equal To 0?(x=w2717) -> (x >= 0?=w2716:bool)
      n1618 = case shown="False" w2716 {
        frame False {
          # "Executable"
          n1619 = control-ref of="This VI"() -> (w2722:refnum<vi>)
          n1620 = invoke class="VI" method="FP.Close"(reference=w2722) -> ()  [unwired: 2 in, 3 out]
        }
        frame True {
          # "LabVIEW Development"
          n1621 = property on="Tab Body" class="TabCtl (strict)"() -> ("Pages"=w2723:refnum<vi>[])  [unwired: 2 in, 2 out]
          n1622 = for {
            tunnel: w2723 -> [w2728] mode=indexing
            n1623 = property class="Page"(reference=w2728) -> (reference out=w2724:refnum<vi>, "PageLabel"=w2727:string)  [unwired: 1 in, 1 out]
            n1624 = Equal?(x=w2727, y="Debug") -> (x = y?=w2725:bool)
            n1625 = case shown="True" w2725 {
              tunnel: w2724 -> [_ w2730]
              frame False {
              }
              frame True {
                n1626 = property class="Page"(reference=w2730, "PageVis"=TRUE) -> ()  [unwired: 1 in, 2 out]
              }
            }
          }
        }
      }
    }
  }
